vi "Core_Chem_User_Interface_v4.0_Scroll_Pump.vi"() -> ()   [LabVIEW 2014]
uses:
  <vilib>/dex/Stream Element Allocation Mode.ctl
  C:/Program Files (x86)/National Instruments/LabVIEW 2014/examples/Data Communication/Network Streams/Simple Network Streams/support/Network Stream Command.ctl
  <vilib>/Platform/TimedLoop/XDataNode/timing_clust.ctl
  <vilib>/Platform/TimedLoop/XDataNode/nitl_modes.ctl
  <vilib>/Platform/TimedLoop/XDataNode/wakeup.ctl
  <vilib>/NI/STM/TCP/Read Meta Data (TCP Ref).vi
  <vilib>/NI/STM/TCP/Get Connection Reference (TCP).vi
  <vilib>/Utility/tcp.llb/UDP Multicast Read-Only Open.vi
  <vilib>/NI/STM/TCP/Read Meta Data (TCP Clst).vi
  <vilib>/NI/STM/TCP/Read Message (TCP).vi
  <vilib>/platform/TimedLoop/XDataNode/XDataNode.xnode
  <vilib>/Platform/TimedLoop/XDataNode/XDNodeRunTimeDep.lvlib
  <vilib>/FTP/NI_FTP.lvlib
  <vilib>/NI/STM/NI STM.lvlib
panel:
  out "FGGA Scroll Pump\ncommand sender error out":errorcluster
  out "FGGA preflight Des 19":string="This tab controls ONLY for advanced operators."
  out "Scroll Pump not running":string
  out "Network Check error out":errorcluster
  out "Scroll Pump Read Error":errorcluster[](array[cluster])
  out "System status register":bool[](array[boolean])
  out "System status register 2":bool[](array[boolean])
  out "Warning register":bool[](array[boolean])
  out "Fault register":bool[](array[boolean])
  in  "Target IP Address":string="192.168.101.17"
  out "Network error out":errorcluster
  out "Create folder error out 3":errorcluster
  out "Network disconnected":bool
  out "cRIO connection status":bool
  out "SO2 Zeroing (Inflight)\nTime Remain (sec)":u32
  in  "eV6 User set time \n(Inflight) (sec)":i32=120
  in  "SO2 Inflight \nZeroing":bool
  out "Create folder error out 2":errorcluster
  out "Create folder error out":errorcluster
  in  "Confirm Flight Number":bool
  out "PRTAFT_UDP_In":string
  out "TWBOZO01":string
  out "CABOZO01":string
  out "TEIOZO01":string
  out "CHTSOO01":string
  out "CHFGGA01":string
  out "AL52CO01":string
  in  "Flight Number":string
  in  "Tab Control":T1(tab)
  out "FGGA preflight Des 17":string="Preflight - Start minimum 2 hours before take-off\n\n1. Ensure no bags/jackets are stowed on seat backs and behind seats in front of core chemistry rack at all times.\n\n2. Remove inlet covers if applicable.\n\n3. Connect Lilliput mini TFT/LCD VGA cable to FGGA VIDEO (back panel) and PS2 Keyboard/Mouse cables to FGGA Connectors (back panel). TFT/LCD screen kept in WAS/GAS rack Zargers Box. Keyboard/Mouse kept bottom of chemistry rack. (DO NOT disconnect PS2 cable). Connect TFT/LCD AC/DC PSU to 6026-8-98 Amphenol (SSP9) and make 230 Vac CB.\n\n4. Ensure all circuit breakers are pushed in, except 230Vac and 28Vdc, UPS switch off (down) and AL5002 CO Plasma Lamp switch off (down), WoW key to normal (horizontal).\n\n5. Wait for ALL network switches on the aircraft to be up and running before start-up. On the Flight Manager's Interface on the Flight Manager laptop, check SSP icons status (top row) should be all green.  \n\n6. Check AboutTime has synchronised laptop clock to aircraft timeservers (Filiberto/Gaston).\n\nClick the PowerUp Tab."
  out "FGGA preflight Des 16":string="PowerUp\n\n1.\tSSP9 forward face\tMake 3 CBs\n\n2.\tPWRDIST \t\tMake 230Vac CB \n                     Switch UPS On \t[UP]\n                     Make 28Vdc CB\n                     Check 28VDC OK Green Light comes on\n\n3.\tCore Chemistry e-Log\nComplete Core Chemistry e-Log in WordPad (Bnnn_CoreChemLog_v2.2), save on Flight Manager's laptop (192.168.101.180/      flt_folders/Bnnn); Fill in header with date, flight number and your name/initials.\n\n4. Wait for MFM flow rate to display non zero value.\n\n5.\tSAMPUMP\t\t\n - Switch WoW override key (vertical) to check pump starts, and MFM flowrate increase (>20 LPM) on the right hand plot. \n - Switch off WoW override\t\t\t\t [NORM, key horizontal]\n\nClick the 2B Ozone tab if operated, otherwise, click the UDP tab.\n\n\n"
  out "MFM":dbl(graph)
  in  "Ambient = OFF\nCabin = ON":bool
  out "FGGA preflight Des 15":string="2B Ozone Preflight\n\n1.\tSelect either Ambient or Cabin Air mode (default should be OFF for Ambient air mode).\n\n2. Check flowrate is greater than 2000 sccm on the right hand plot.\n\nClick the UDP tab."
  out "2B Ozone concentration":dbl(graph)
  out "2B Ozone flow rate":dbl(graph)
  out "2BOzone Event error out":errorcluster
  out "2BOzone command sender error out":errorcluster
  out "FGGA preflight Des 20":string="4. Check derived parameters in DECADES (192.168.101.110 & 192.168.101.108). 574 Ozone TEi49C; 588 CO AL5002; 611 SO2 TEi43i; 903 - 905 FGGA; 910 / 920 Ozone 2B."
  out "FGGA preflight Des 14":string="UDP Preflight\n1. Check all UDP packets are updating.  Unix time increasing by 1 sec (3rd parameter).\n2. Check flight number is correct.\n3. Confirm flight number and check it appears in the UDP packet (6th parameter). "
  in  "name":string="239.1.4.6"
  in  "Port":u16=50001
  out "FGGA":string
  out "CO":string
  out "TEi49 Ozone":string
  out "2B Cabin Ozone":string
  out "2B Ambient Ozone":string
  out "SO2":string
  in  "Ozone Zeroing Abort":bool
  out "Ozone Zeroing\nTime Remain (sec)":u32
  in  "Ozone Zeroing":bool
  out "TEI49 Sample Flow B":dbl(graph)
  out "TEi49 Concentration":dbl(graph)
  out "TEI49 Sample Flow A":dbl(graph)
  out "FGGA preflight Des 13":string="TEi49 Ozone PRE-FLIGHT - LAST ACTIONS BEFORE SEAT-BELTING DOWN (PRIOR TO ENGINES START)\n\n1. Ozone monitor zeroing\t\t[10 min minimum]\n\n\n2. Check TEi49 zero value and note down value in e-Log. \n"
  out "FGGA preflight Des 12":string="TEi49 Ozone Preflight\n\n1. Check nominal sample flowrate on both channels is ~0.7 LPM."
  out "Ozone Event error out":errorcluster
  out "Ozone command sender error out":errorcluster
  in  "Ozone UDP Time Offset":i32=1
  in  "eV8 span\n(sec)":i32=120
  in  "eV9 span\nflush (sec)":i32=60
  in  "SO2 Span Calibration":bool
  in  "eV9 zero\nflush (sec)":i32=15
  in  "SO2 Zero Calibration":bool
  in  "eV8 zero\n(sec)":i32=30
  in  "SO2 Calibration Abort":bool
  out "SO2 react pressure":dbl(graph)
  in  "Prepare SO2 Zero Gas":bool
  in  "Prepare SO2 Span Gas":bool
  in  "Auto Zeroing \ninterval (sec)":i32=600
  out "Next Auto Zero\nStarts in (sec)":u32
  out "Auto Zero\nIndicator":string="Auto Zero Inactive; Manual Zero Allow"
  out "SO2 Resume Zeroing\nCount down timer (sec)":u32
  in  "SO2 Pause\nAuto Zeroing":bool
  out "TEi43i Concentration scaled / raw":cluster{dbl, dbl}(graph)
  in  "SO2 Auto Zeroing":bool
  out "mean zero\ncal status":bool
  out "SO2 Sensitivity":dbl format="%.2g"
  out "SO2 Zero":dbl format="%.2g"
  in  "eV9 Flush User\nset time (sec)":i32=15
  in  "MFC_3 User Set Value":dbl=2.0
  in  "MFC_2 User Set Value":dbl=2.5
  in  "eV6 User\nset time (sec)":i32=600
  out "SO2 Flush\nTime Remain (sec)":u32
  out "TEI43i MFC3 Sample Flow":dbl(graph)
  out "TEI43C Sample Flow":dbl(graph)
  out "TEI43i MFC2 Cal Flow":dbl(graph)
  out "SO2 Zero CAL\nTime Remain (sec)":u32
  out "SO2 Zero CAL Flush\nTime Remain (sec)":u32
  in  "SO2 Zero CAL":bool
  out "FGGA preflight Des 11":string="TEi43 SO2 Inflight Zero Calibration"
  in  "SO2 GND Zeroing":bool
  out "SO2 Zeroing\nTime Remain (sec)":u32
  out "FGGA preflight Des 10":string="TEi43 SO2 PRE-FLIGHT - LAST ACTIONS BEFORE SEAT-BELTING DOWN (PRIOR TO ENGINES START)\n\n1. SO2 monitors zeroing\t\t[10 min minimum]\n\n2. Check TEi43i or TEi43C zero value and note down value in e-Log.\n\n3. Enable SO2 auto zeroing (if required) and check zeroing interval. "
  in  "SO2 Flush":bool
  out "FGGA preflight Des 9":string="TEi43 SO2 Preflight\n\n1. Check nominal sample flowrate is (2.0 LPM / 1.5 LPM) on the (TEi43i / TEi43c) right hand plot.\n\nSPAN GAS\n1. Connect SO2 Calibration gas to caldeck, then.\n\n2. Press SO2 flush button, MFC2 cal flow should increase to 2.5 SLPM.\nMonitor MFC2 flow rate to make sure the reading decreases from 2.5 SLPM to 0.0 SLPM.\nCheck pressure content and delivery gauges also reads zero.\nIf pressure content & delivery gauges do NOT read zero, press SO2 flush button again until they do.\n\n3. Back out V2, Quickly open and close cylinder valve 1, Set delivery pressure to 3 bar on V2. \n\n4. Repeat step 2) to 3) three times.\n\n5. Open cylinder valve 1, system is ready. Note down content pressure in elog.\n\n6. Press SO2 Span Calibration button to start Span calibration. \n\nZERO AIR\n1. Connect BTCA Zero Air gas to caldeck, then.\n\n2. Set ev9 flush user time to 60 secs and press SO2 Flush button.\n\n3. Press SO2 Zero Calibration button to start Zero Air calibration."
  in  "eV9 flush User\nset time (sec)":i32=30
  in  "eV8 User\nset time (sec)":i32=60
  out "SO2 Event error out":errorcluster
  out "SO2 command sender \nerror out":errorcluster
  in  "SO2 UDP Time Offset":i32=1
  in  "CO Monitor Troubleshooting":bool
  out "Lamp Temperature":dbl(graph)
  out "CO CAL Status":bool
  in  "CO CAL":bool
  out "FGGA preflight Des 8":string="CO Preflight and Inflight Calibrations\nHold down the CAL button for 2 secs then release, CAL status should then lit up.\nCheck CO LED lit up at front instrument. If not, refer to\nInflight calibration performed on 45 minutes interval or more frequently if lamp temperature > 35.5 degC."
  in  "Prepare Gases":bool
  out "FGGA preflight Des 7":string="AL5002 CO Preflight Checks\n\n1.\n\n2. Start CO Vacuum. NB: If there is problem with the software control, use manual override switch [up] on CALDECK front panel\n\n3. CO Checks - charts on the right hand side\n    Lamp Flow Controller ~ 40 ml/min\n    Monochromator Flow Controller ~ 30 ml/min\n    Fluorescence Cell Pressure ~ 7.5 Torr\n\nIf Lamp/Mono flows are low, manual valves (V1 -> V5) may still be shut, or pressure adjusting valves (ALREG1 & 2) have not been set > 2 bar\n\nIf Cell pressure is 10 Torr (max range), check that COPUMP is running and eV7 is opened (CO Vacuum eV7 is ON).\n\n4. Switch Plasma Lamp at the front panel UP\n\nDetector count rate (on 'Raw Signal' or F2 instrument touchscreen) should increase to >=10000 Hz within a minute.  Recycle plasma lamp switch (off/on) if no significant increase in count rate after 10 mins.  CO concentration should increase (100s ppb). \n     \n\n"
  in  "CO Vaccum (eV7)":bool
  out "Raw Signal":dbl(graph)
  out "CO Concentration":dbl(graph)
  out "Fluorescence Cell Pressure":dbl(graph)
  out "Monochromator Flow":dbl(graph)
  out "Lamp Flow Controller":dbl(graph)
  in  "CO UDP Time Offset":i32=1
  out "CO2 Pressure\nDelivery (PSIA)":dbl(slide) scale=0.0..100.0
  out "Std\nContent (barG)":dbl(slide) scale=0.0..220.0
  out "N2\nContent (barG)":dbl(slide) scale=0.0..220.0
  out "CO2\nContent (barG)":dbl(slide) scale=0.0..170.0
  out "CO Event error out":errorcluster
  out "CO command sender error out":errorcluster
  out "CO Zero":T2(array[cluster])
  out "CO Sensitivity":T3(array[cluster])
  in  "NEW\nFGGA Restart":bool
  in  "FGGA Calibration Abort":bool
  out "Ring Down Time RDA & RDB":cluster{dbl, dbl}(graph)
  in  "Line Lock Setting Change":bool
  out "Cell temperature":dbl(graph)
  out "Cell pressure":dbl(graph)
  in  "Manual FGGA Pump":bool
  out "CO2":dbl(graph)
  out "CH4":dbl(graph)
  out "H2O":dbl(graph)
  out "WoW Flag":string="0"
  in  "FGGA pump\nsync to WoW":bool
  out "CH4 Dry":dbl(graph)
  out "CO2 Dry":dbl(graph)
  out "MFC1 Cal Flow":dbl(graph)
  out "Flush Target Tank\nTime Remain (sec)":u32
  out "Flush Low Tank\nTime Remain (sec)":u32
  out "Flush High Tank\nTime Remain (sec)":u32
  in  "Flush Target Tank":bool
  in  "Flush Low Tank":bool
  in  "Flush High Tank":bool
  in  "OLD\nFGGA Restart":bool
  out "FGGA preflight Des 6":string="FGGA Instrument Controls"
  in  "High Cal":bool
  out "High Cal\nFlush Time Remain (sec)":u32
  out "High Cal\nCal Time Remain (sec)":u32
  in  "Low Cal":bool
  in  "Target Cal":bool
  in  "Span Cal - \nHigh Cal, CO Cal, Low Cal":bool
  out "Low Cal\nFlush Time Remain (sec)":u32
  out "Low Cal\nCal Time Remain (sec)":u32
  out "Target Cal\nFlush Time Remain (sec)":u32
  out "Target Cal\nCal Time Remain (sec)":u32
  in  "MFC_1 User Set Value":dbl=2.0
  out "FGGA preflight Des 5":string="FGGA Inflight Calibrations"
  out "FGGA preflight Des 4":string="FGGA Ground Preflight Checks\n\n1. Switch FGGA pump ON\n\n2. Check cavity pressure ~50 Torr\n\n3. Switch FGGA pump OFF\n\n4. Enable FGGA pump sync to WoW\n\n5.. Check Time Synchronisation\n\n6. Check CO2 & CH4 values\n\nIf CO2 & CH4 values are -1 ppm, follow the \nchange linelock settings procedure.\n\n\n\n\n\nLAST ACTION BEFORE SEAT-BELTING \nDOWN (PRIOR TO ENGINES START)\n\n1. Disconnect Monitor & stow away. Leave Keyboard & Mouse connected. Place keyboard at the bottom\nof the rack.\n\n"
  out "FGGA preflight Des 3":string="FGGA CAL Gas Purge\n\nFor each cylinder in gas stowage, check that,\n\n1. V1 Closed\n    V3 Closed\n    V4 Make sure arrow positioned downwards (i.e. flow points to gas line)\n\n2. V3 Open (turn anti-clockwise)\n\n3. Use the button on the right according to the operating cylinder to flush the line. Monitor the MFC flow rate to make sure the reading decreases from 3 to zero. (ie fully flushed). Pressure content & delivery gauges should also read zero.\n\n4. V3 Close (turn clockwise)\n\n5. V1 Open / Close quickly\n         Check delivery pressure gauge is ~ 40 PSI \n         (Use V2 to increase if necessary)\n\n6. Repeat steps 2) to 5) three times\n\n7. V3 Close (turn clockwise)\n\n8. V1 Open, check V2 ~ 40 PSIG\n\n9. V3 Open - System is ready"
  out "FGGA command sender error out":errorcluster
  out "FGGA Event Error out":errorcluster
  in  "FGGA UDP Time Offset":i32=1
  in  "Span Low Flush Time (seconds)":i32=21
  in  "Span Low Cal Time (seconds)":i32=30
  in  "Span High, High Low, Target\nCal Time (seconds)":i32=30
  in  "Span High, High, Low, Target  Cal\nContinue Flush Time (seconds)":i32=11
  in  "Span High, High, Low, Target Cal\nFlush Start Time (seconds)":i32=10
  in  "Time delay (msec) between\nvalves switching":u32=200
  in  "FLOW ALL OFF":bool
  in  "LOW FLOW MASTER SWITCH":bool
  in  "FGGA 140 Torr\nCalibration Abort":bool
  out "Ring Down Time RDA & RDB 2":cluster{dbl, dbl}(graph)
  out "Cell temperature 2":dbl(graph)
  out "Cell pressure 2":dbl(graph)
  out "CO2 2":dbl(graph)
  out "CH4 2":dbl(graph)
  out "H2O 2":dbl(graph)
  out "CH4 Dry 2":dbl(graph)
  out "CO2 Dry 2":dbl(graph)
  in  "High Cal\n140 Torr":bool
  out "High Cal 140 Torr\nFlush Time Remain (sec)":u32
  out "High Cal 140 Torr\nCal Time Remain (sec)":u32
  in  "Low Cal\n140 Torr":bool
  in  "Target Cal\n140 Torr":bool
  in  "Span Cal 140 Torr - \nHigh Cal, CO Cal, Low Cal":bool
  out "Low Cal 140 Torr\nFlush Time Remain (sec)":u32
  out "Low Cal 140 Torr\nCal Time Remain (sec)":u32
  out "Target Cal 140 Torr\nFlush Time Remain (sec)":u32
  out "Target Cal 140 Torr\nCal Time Remain (sec)":u32
  in  "MFC_1 140 Torr\nUser Set Value":dbl=4.0
  out "FGGA preflight Des 23":string="FGGA 140 Torr Inflight Calibrations"
  in  "eV10":bool
  out "Scroll Pump \nat Fault":bool
  out "Measured Motor Current (A)":dbl(graph)
  out "Measured Link Voltage (V)":dbl(graph)
  out "Measured Motor Power (W)":dbl(graph)
  out "Motor Frequency":i32(graph)
  out "Receiver Loop Count":i32
  in  "Standby Speed %\nDefault Set Value":u32=66 min=66 max=100
  in  "Normal Speed Threshold":u32(slide)=50 min=50 max=100 scale=50.0..100.0
  in  "Standby Speed\n66% - 100%":u32=66 min=66 max=100
  in  "Use Standby Speed":bool
  in  "Scroll Pump On/Off":bool
  in  "Scroll Pump Faults":bool
  out "FGGA Scroll Pump Monitoring":string[](array[string])
  out "Pump Controller Temperature":i32(slide) scale=0.0..100.0
  in  "HIGH FLOW MASTER SWITCH":bool
  in  "NEW FGGA Shutdown":bool
  in  "Transfer NEW FGGA Files":bool
  in  "OLD FGGA Shutdown":bool
  in  "Postflight Procedures":bool
  in  "FTP ASCII Files to Local":bool
  in  "Transfer OLD FGGA Files":bool
  out "FGGA preflight Des 18":string="Postflight\n\n1. Perform SO2 Span Gas Calibration (if necessary). \n\n2. Press the FTP ASCII File to Local button to transfer ASCII files to flight folder.\n\n\n3. Press the Transfer FGGA Files button to transfer FGGA files to flight folder. \n\n\n4. Shutdown FGGA.\n\n\n5. View Postflight Procedures."
  out "File List":string[](array[string])
  out "FGGA File Transfer Error out":errorcluster
  out "Move to FM Error out":errorcluster
  out "FGGA File Transfer Error out 2":errorcluster
  out "USB Disk Space Used %":dbl(slide) scale=0.0..100.0
  out "PTP Sync":bool
  out "CPU Total %":dbl(graph)
  out "PRTAFT_DLU":string
  in  "eV12":bool
  in  "eV11":bool
  in  "Pause Auto Zero Count \nDown set time (sec)":i32=600
  out "Calibration gas cylinder \nconcentration (ppb)":dbl format="%.4g"
  in  "Save Calibration gas\ncylinder concentration to file":bool
  in  "Calibration gas cylinder \nconcentration (ppb)":dbl=500.0 format="%.4g"
  in  "Simulate MOCCA Conc":dbl
  in  "MOCCA window \ndelay time (sec)":i32=30
  in  "MOCCA Limit":i32=800
  in  "SO2 Inflight MOCCA Alarm\n(default = OFF)":bool
  in  "Offset Mean Zero Calculation (default = ON)\nOFF = User input\nOn = Mean zero calculated with ev8":bool=TRUE
  in  "Inst_alm_thresh":i32=220
  in  "3hr_alm_thresh":i32=80
  in  "Simulate Inst Conc":i32
  in  "Simulate 3hr Average Conc":dbl
  in  "Simulate 2B Conc":bool
  in  "Ozone eV6":bool
  in  "Simulate Conc":bool
  in  "8hr TWA Limit":i32=490
  in  "10mins STEL Limit":i32=800
  in  "SO2 Sensitivity":dbl=1.1
  in  "SO2 Zero":dbl
  in  "Simulate TWA Conc":dbl
  in  "Simulate STEL Conc":dbl
  in  "MFC_3\nSLPM Value":dbl=2.0
  in  "MFC_2\nSLPM Value":dbl
  in  "SO2 eV6":bool
  in  "eV8":bool
  in  "eV9":bool
  in  "eV4":bool
  in  "eV3":bool
  in  "MFC_1\nSLPM Value":dbl
  in  "eV2":bool
  in  "eV1":bool
  in  "cRIO File IO Stop\n(USB Flash Drive Unmount)":bool
  # "Stop command received and pump is stopping"
  # "Power limit is active"
  # "Accelerating / running"
  # "Acceleration is limited"
  # "Standby Active"
  # "Deceleration is limited"
  # "Above normal speed"
  # "Operating above the ramp speed threshold"
  # "Operating above the overload speed threshold"
  # "Warning Condition"
  # "Control mode"
  # "Fault Condition"
  # "Serial enable active"
  # "Unix time"
  # "Flight Number"
  # "concentration (scaled)\npmt_volt\nlamp_volt\nlamp_intens\ninternal_temper\nreact_temper\nreact_press\nflow\nflags\nten_min_so2\neight_hr_so2\nten_min_so2_alm\neight_hr_so2_alm\nMFC_2absolute_pres\nMFC_2temperature\nMFC_2volumetic_flow\nMFC_2mass_flow\nMFC_2set_point\nMFC_3_absolute_pres\nMFC_3_temperature\nMFC_3volumetic_flow\nMFC_3mass_flow\nMFC_3set_point\nV6\nV8\nV9\nMFC2_Set_Value\nMFC3_Set_Value\nconcentration (raw)\nmean calculation status\noffset\nsensitivity\nev8_user_set_time\nauto_zeroing_control\nev8_zero_interval\nMOCCA_inflight_alarm\nMOCCA_time_window_delay\nMOCCA_SO2_limit\n10 min STEL limit\n8 hour TWA limit\nSO2 cal gas cylin conc\nsimulate_SO2_conc_control\nMOCCA_SO2_sim_value\nMOCCA_SO2_alarm"
  # "Unix time"
  # "Unix time"
  # "Unix time"
  # "Unix time"
  # "Flight Number"
  # "Flight Number"
  # "Flight Number"
  # "Flight Number"
  # "conc\ntemp\npress\nflow\nthreehr_oz\nInst_alarm\nthreehr_alarm"
  # "ch4\nco2\nh2o\npress_torr\ntemp_c\nfit_flag\nrda_usec\nrdb_usec\nch4_dry\nco2_dry\nMFC_1_absolute_pres\nMFC_1_temperature\nMFC_1volumetic_flow\nMFC_1mass_flow\nMFC_1set_point\nV1\nV2\nV3\nV4\nrestart_FGGA\nFGGA_Pump\nCAL_MFC_1Set_Value"
  # "conc\ntemp\npress\nflow"
  # "conc\nbenchtemp\npress\ncellAint\ncellBint\nFlowA\nFlowB\nlamptemp\nflag\nV6"
  # "conc\ncounts\nsens\nzero\nlampflow\nlamptemp\nmonoflow\nmonotemp\nmonopress\ncellpress\ncalpress\ntemppmt\ncalconc\nerr\ncal_counter\nerr_counter\nCO_vacuum_status\nIn_Cal\nALEG1_press_delivery\nALREG1_press_content\nALREG2_press_content\nALREG3_press_content"
  # "TEi43c"
  # "TEi43i"
  # "SO2 Inflight ZERO CAL SETTINGS"
  # "FGGA Scroll Pump"
  # "FGGA"
  # "2B Ozone"
  # "TEi49C  - Ozone"
  # "TEi43 - SO2"
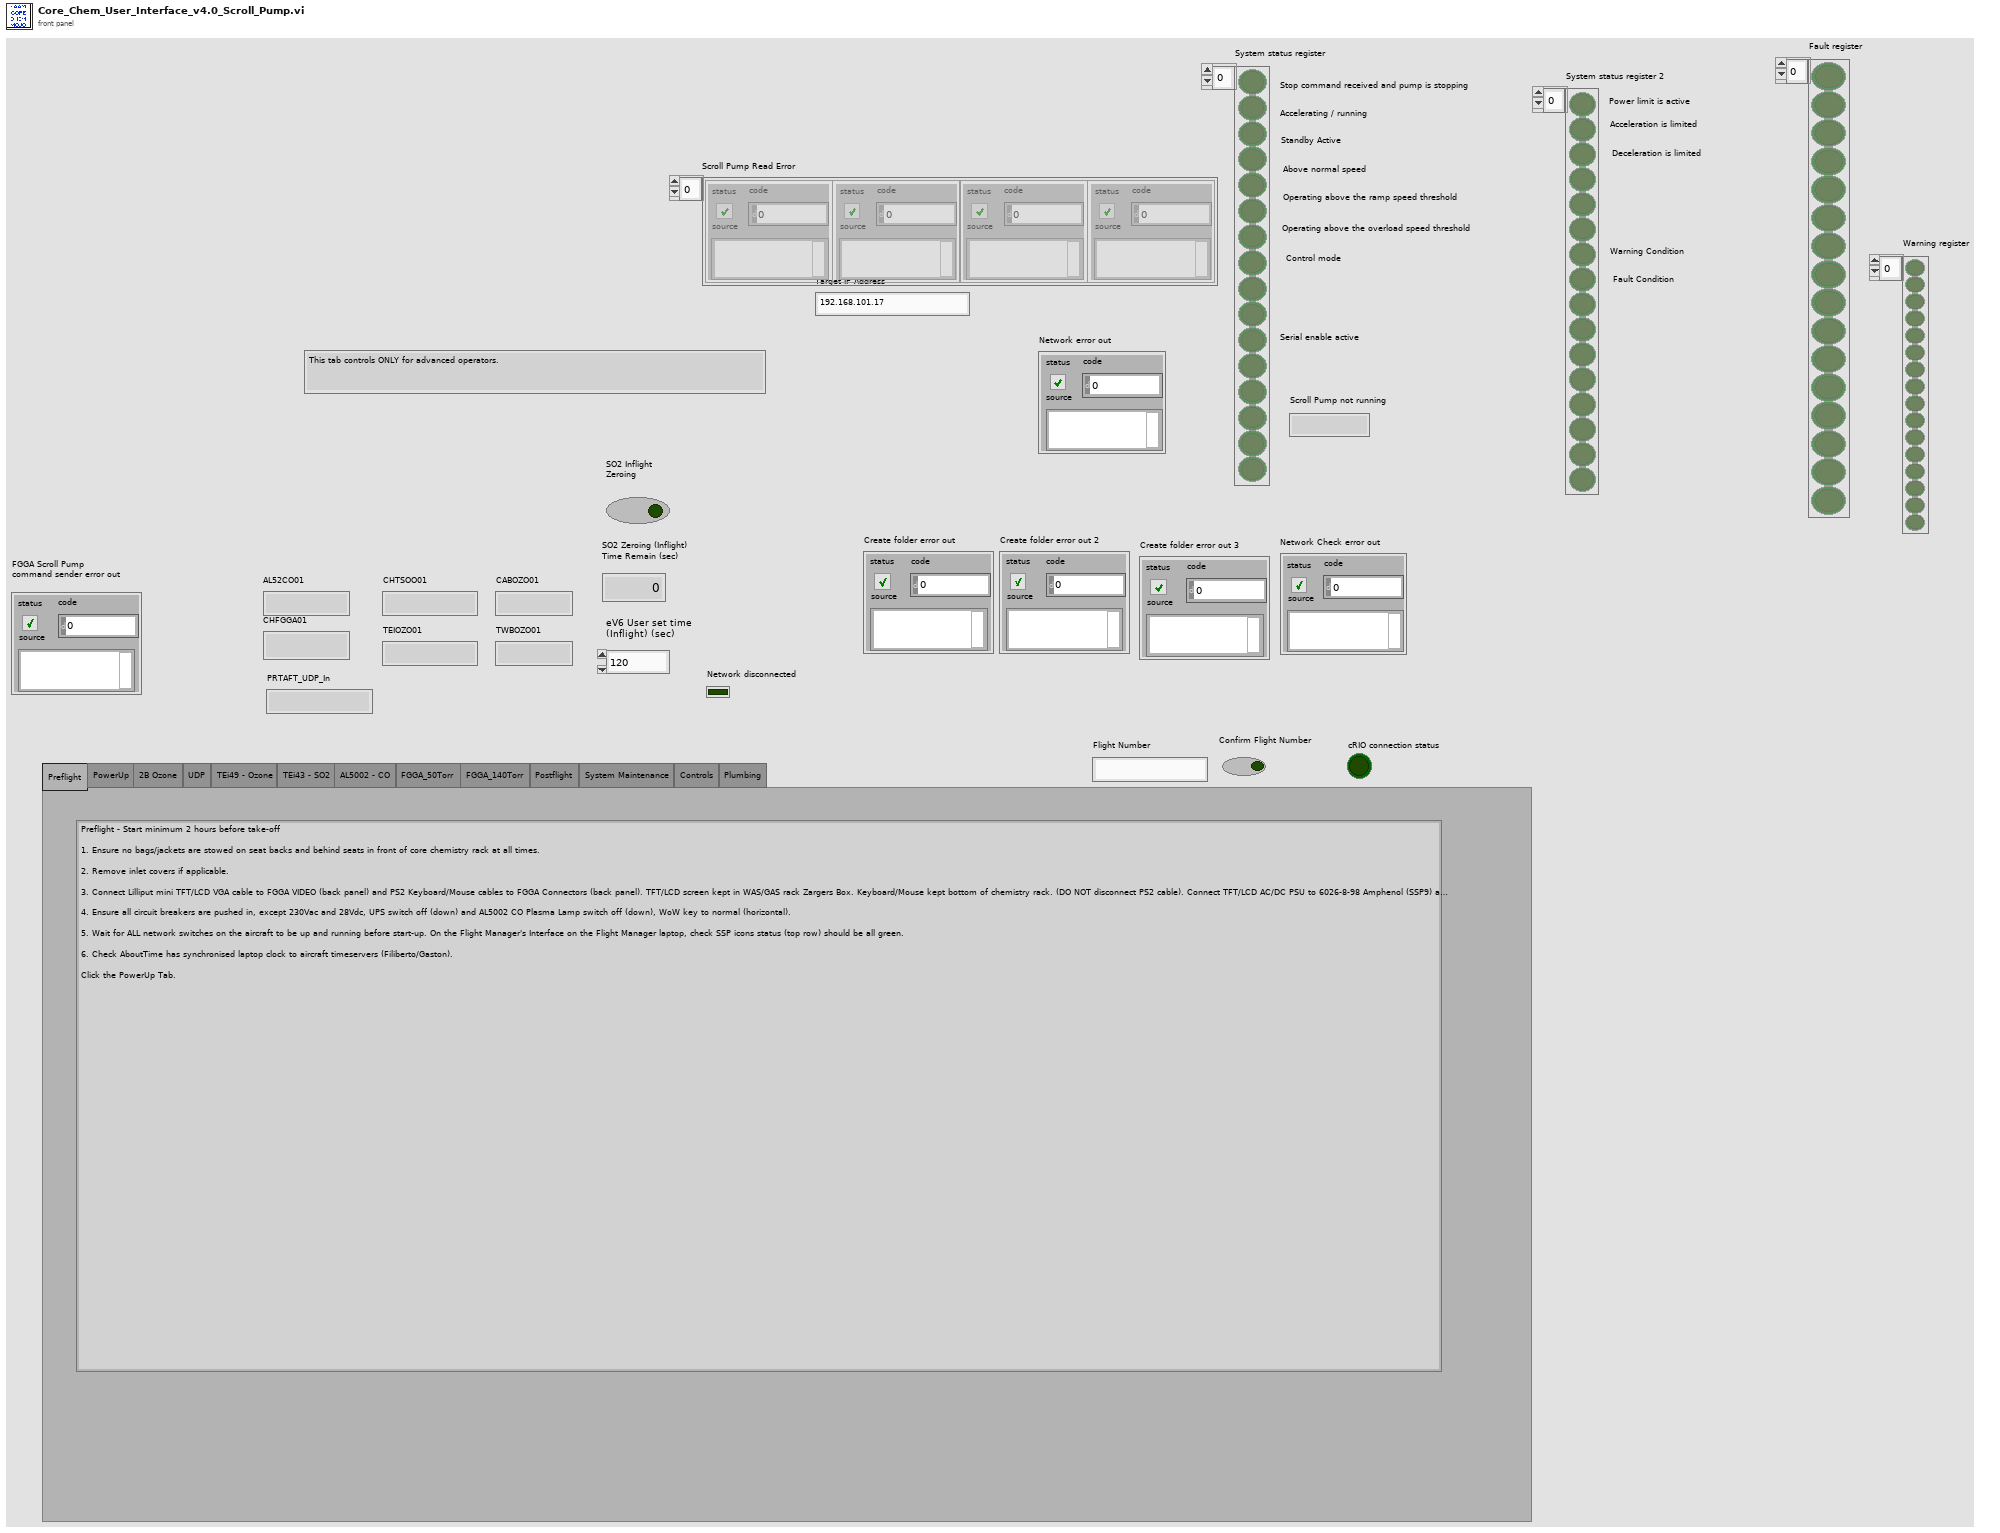
[diagram p1: front panel]
types:
  T1 = enum32{"Preflight", "PowerUp", "2B Ozone", "UDP", "TEi49 - Ozone", "TEi43 - SO2", "AL5002 - CO", "FGGA_50Torr", "FGGA_140Torr", "Postflight", "System Maintenance", "Controls", "Plumbing"}
  T2 = cluster{"time stamp":timestamp, "CO Offset":dbl}[]
  T3 = cluster{"time stamp":timestamp, "CO Sensitivity":dbl}[]
  T4 = typedef "Stream Element Allocation Mode.ctl" = u32
  T5 = typedef "Network Stream Command.ctl" = cluster{"Message":string, "Message Data":variant}
  T6 = typedef "XDNodeRunTimeDep.lvlib/timing_clust.ctl" = cluster{"Expected End [f-1]":u64, "Actual End [f-1]":u64, "Finished Late? [f-1]":bool, "Expected End [i-1]":u64, "Actual End [i-1]":u64, "Finished Late? [i-1]":bool, "Expected Start [i]":u64, "Actual Start [i]":u64, "Expected Start [f]":u64, "Actual Start [f]":u64, "Source Name":string, "Structure Name":string, "Period":i64, "Deadline":i64, "Offset":i64, "Start":i64, "Priority":i32, "Timeout":i32, "Mode":T7, "Wakeup Reason":T8, "Error":errorcluster, "Source Type":string, "Secondary Source Type":string, "Global End Time":u64, "Global Start Time":u64, "Frame Duration":u64, "Iteration Duration":u64, "Assigned CPU":i32, "I/O Scan Engine Mode":u32}
  T7 = typedef "XDNodeRunTimeDep.lvlib/nitl_modes.ctl" = enum32{"No Change", "Process missed periods, maintain original phase", "Discard missed periods, maintain original phase", "Process missed periods, ignore original phase", "Discard missed periods, ignore original phase"}
  T8 = typedef "XDNodeRunTimeDep.lvlib/wakeup.ctl" = enum32{"Normal", "Aborted", "Asynchronous wakeup", "Timing source error", "Timed loop error", "Timeout"}
  T9 = typedef "NI_FTP.lvlib/FTP Session.ctl" = refnum<k5>
  T10 = typedef "NI_FTP.lvlib/FTP File Info.ctl" = cluster{"type":enum16{"unknown", "file", "dir", "link"}, "permissions":string, "owner":string, "group":string, "size":i32, "date":string, "name":string, "link name":string}
  T11 = cluster{"Message":string, "Message 2":string, "Message 3":string}
  T12 = cluster{"Message":string, "Message 2":string, "Message 3":string, "Message 4":string}
  T13 = cluster{"Message 2":string, "Message 3":string, "Message 4":string}
  T14 = cluster{"Message":string, "Message 3":string, "Message 4":string}
  T15 = typedef "NI STM.lvlib/TCP Connection Info.ctl" = cluster{"connection ID":refnum<k5>, "meta data":T16[]}
  T16 = typedef "NI STM.lvlib/MetaDataElement.ctl" = string
  T17 = typedef "NI STM.lvlib/TCP Data Info.ctl" = cluster{"data size":i32}
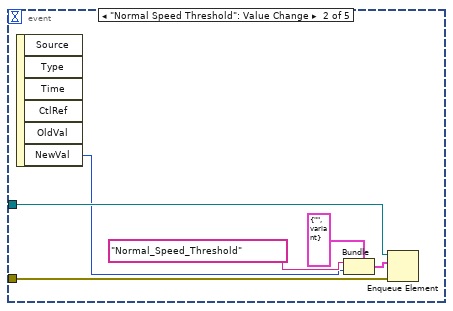
[diagram p3: hidden frame]
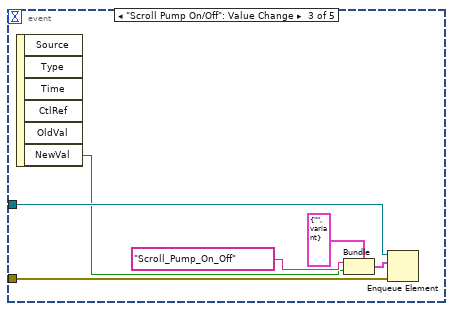
[diagram p4: hidden frame]
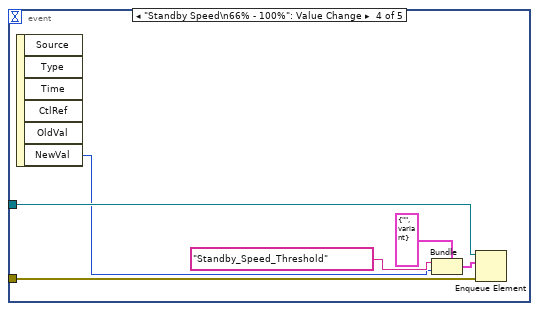
[diagram p5: hidden frame]
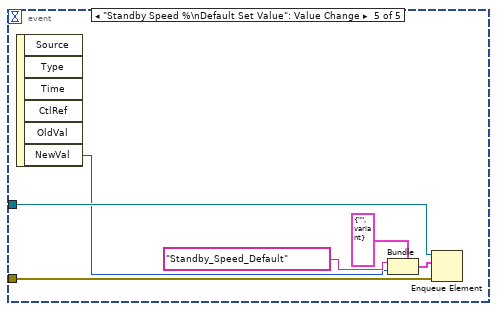
[diagram p6: hidden frame]
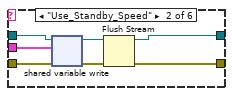
[diagram p8: hidden frame]
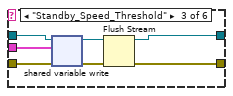
[diagram p9: hidden frame]
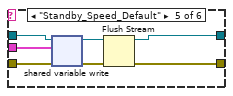
[diagram p10: hidden frame]
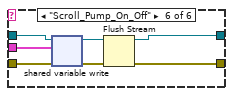
[diagram p11: hidden frame]
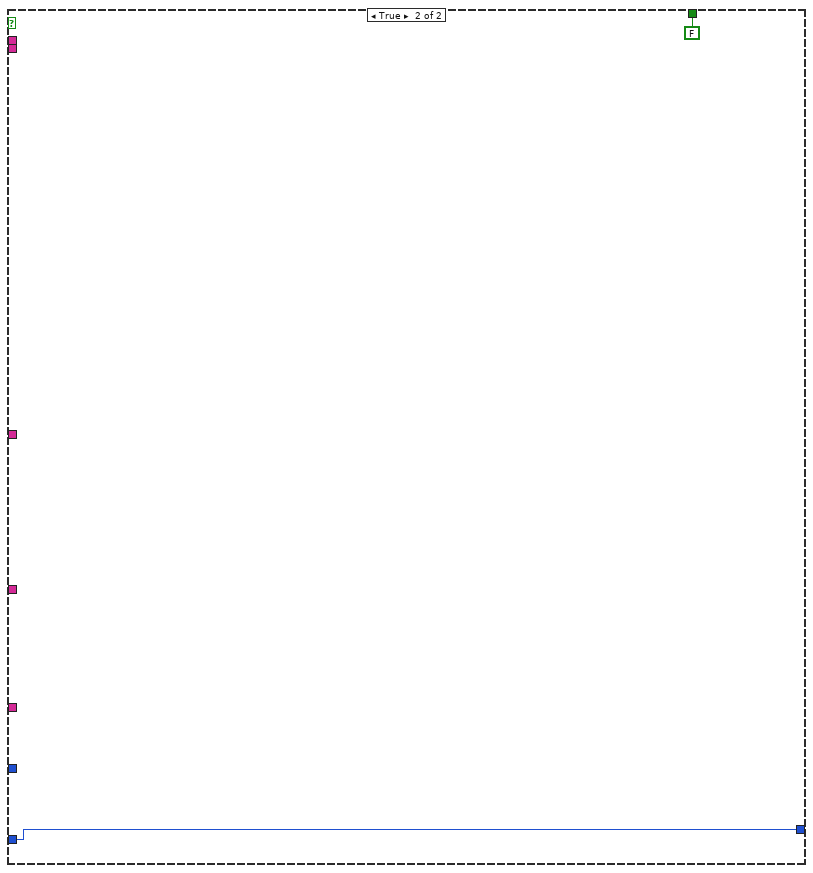
[diagram p16: hidden frame]
diagram:
  w8 = T4 0 items=["allocate as needed", "pre-allocate"] ("element allocation mode")
  w3 = T5 {"Message"="", "Message Data"=variant} ("Message Cluster")
  w19 = "XXXX"
  w21 = 0
  w22 = 0.0
  w28 = T5 {"Message"="", "Message Data"=variant} ("Message Cluster")
  w34 = T4 0 items=["allocate as needed", "pre-allocate"] ("element allocation mode")
  w40 = T5 {"Message"="", "Message Data"=variant} ("Message Cluster")
  w46 = T4 0 items=["allocate as needed", "pre-allocate"] ("element allocation mode")
  w51 = T5 {"Message"="", "Message Data"=variant} ("Message Cluster")
  w56 = T4 0 items=["allocate as needed", "pre-allocate"] ("element allocation mode")
  w65 = T4 0 items=["allocate as needed", "pre-allocate"] ("element allocation mode")
  w67 = T5 {"Message"="", "Message Data"=variant} ("Message Cluster")
  w74 = T4 0 items=["allocate as needed", "pre-allocate"] ("element allocation mode")
  w76 = T5 {"Message"="", "Message Data"=variant} ("Message Cluster")
  n1 = local write "cRIO File IO Stop\n(USB Flash Drive Unmount)"(FALSE ("Stop File Write")) -> ()
  n2 = local write "Flight Number"(w19) -> ()
  n3 = while {
    shift-right: [w80] -> _
    shift-left: w19 -> [w79]
    stop <- FALSE stop-if-true
    n4 = Not Equal?(x=w79, y="Flight Number") -> (x != y?=w82:bool)
    n5 = case shown="True" w82 {
      tunnel: [w85 w86] -> w80
      tunnel: "Flight Number" -> [_ w86]
      tunnel: w79 -> [w85 _]
      frame False {
      }
      frame True {
        n6 = One Button Dialog(message="Flight Number changed,\nPress flight number button to confirm") -> ()  [unwired: 1 in, 1 out]
      }
    }
    n7 = Wait (ms)(milliseconds to wait=u32 1000) -> ()  [unwired: 1 out]
  }
  n8 = while {
    stop <- FALSE stop-if-true
    # "UDP Read"
    n9 = String To IP(1:"name") -> (0:w93:u32)
    n10 = call-poly <vilib>:"UDP Multicast Open.vi"("multicast addr"=w93, "port"="Port") -> ("error out"=w91:errorcluster, "connection ID"=w90:refnum<k16>)  [unwired: 7 in, 1 out]
    n11 = Wait (ms)(milliseconds to wait=u32 1000) -> ()  [unwired: 1 out]
    n12 = case shown="No Error" w91 {
      selector: w91 -> [w97 _]
      tunnel: w90 -> [w96 _]
      frame No Error {
        w95 = ""
        n13 = while {
          tunnel: w97 -> [w143]
          tunnel: w96 -> [w142]
          shift-right: [w138] -> _
          shift-left: w95 -> [w139]
          shift-right: [w129] -> _
          shift-left: w95 -> [w131]
          shift-right: [w123] -> _
          shift-left: w95 -> [w125]
          shift-right: [w117] -> _
          shift-left: w95 -> [w118]
          shift-right: [w111] -> _
          shift-left: w95 -> [w112]
          shift-right: [w105] -> _
          shift-left: w95 -> [w106]
          shift-right: [w99] -> _
          shift-left: w95 -> [w100]
          stop <- w141 stop-if-true
          n14 = UDP Read(connection ID=w142, 8:w143) -> (data out=w98:string, error out=w141:errorcluster)  [unwired: 2 in, 3 out]
          n15 = Match Pattern(string=w98, regular expression="$TEIOZO") -> (match substring=w137:string, after substring=w136:string)  [unwired: 1 in, 2 out]
          n16 = Match Pattern(string=w98, regular expression="$TWBOZO01,") -> (match substring=w115:string, after substring=w114:string)  [unwired: 1 in, 2 out]
          n17 = Match Pattern(string=w98, regular expression="$CABOZO01,") -> (match substring=w121:string, after substring=w120:string)  [unwired: 1 in, 2 out]
          n18 = Match Pattern(string=w98, regular expression="$CHTSOO") -> (match substring=w109:string, after substring=w108:string)  [unwired: 1 in, 2 out]
          n19 = Match Pattern(string=w98, regular expression="$CHFGGA") -> (match substring=w133:string, after substring=w132:string)  [unwired: 1 in, 2 out]
          n20 = Match Pattern(string=w98, regular expression="$AL52CO01,") -> (match substring=w127:string, after substring=w126:string)  [unwired: 1 in, 2 out]
          n21 = Match Pattern(string=w98, regular expression="$PRTAFT01,") -> (match substring=w104:string, after substring=w103:string)  [unwired: 1 in, 2 out]
          n22 = Concatenate Strings(w137, w136) -> (w135:string)
          n23 = Concatenate Strings(w115, w114) -> (w113:string)
          n24 = Concatenate Strings(w121, w120) -> (w119:string)
          n25 = Concatenate Strings(w109, w108) -> (w107:string)
          n26 = Concatenate Strings(w133, w132) -> (w130:string)
          n27 = Concatenate Strings(w127, w126) -> (w124:string)
          n28 = Concatenate Strings(w104, w103) -> (w101:string)
          n29 = Replace Substring(4:w113, 5:w112) -> (1:w111:string)  [unwired: 2 in, 1 out]
          "TWBOZO01" <- w111
          n30 = Replace Substring(4:w135, 5:w139) -> (1:w138:string)  [unwired: 2 in, 1 out]
          "TEIOZO01" <- w138
          n31 = Replace Substring(4:w119, 5:w118) -> (1:w117:string)  [unwired: 2 in, 1 out]
          "CABOZO01" <- w117
          n32 = Replace Substring(4:w107, 5:w106) -> (1:w105:string)  [unwired: 2 in, 1 out]
          "CHTSOO01" <- w105
          n33 = Replace Substring(4:w124, 5:w125) -> (1:w123:string)  [unwired: 2 in, 1 out]
          "AL52CO01" <- w123
          n34 = Replace Substring(4:w130, 5:w131) -> (1:w129:string)  [unwired: 2 in, 1 out]
          "CHFGGA01" <- w129
          n35 = Replace Substring(4:w101, 5:w100) -> (1:w99:string)  [unwired: 2 in, 1 out]
          "PRTAFT_UDP_In" <- w99
        }
      }
      frame Error {
      }
    }
  }
  n36 = Obtain Queue(name (unnamed)="CO_Command", element data type=w76) -> (queue out=w27:refnum<queue>, error out=w70:errorcluster)  [unwired: 3 in, 1 out]
  n37 = Create Network Stream Writer Endpoint(6:w74, 7:10 ("writer buffer size"), 9:w76, 10:"//192.168.101.17/command/reader/CO" ("reader url"), 11:"/command/writer/CO" ("writer name")) -> (0:w73:errorcluster, 3:w72:refnum<k21>)  [unwired: 2 in]
  n38 = while {
    tunnel: w27 -> [w147]
    tunnel: w70 -> [w146]
    tunnel: [w144] -> _
    stop <- FALSE stop-if-true
    # "CO UI Event Handler Loop"
    n39 = event shown="[4] \"Confirm Flight Number\": Value Change" {
      selector: _ -> [_ _ _ _ _]
      dyn-events: _ -> [_ _ _ _ _]
      timeout: _ -> [_ _ _ _ _]
      tunnel: w147 -> [w154 w161 w165 w172 w180]
      tunnel: w146 -> [w153 w160 w164 w171 w179]
      tunnel: [w148 w155 w163 w170 w178] -> w144
      event "CO CAL": Value Change {
        n40 = event-data() -> ("NewVal"=w151:bool)  [unwired: 1 in]
        n41 = Bundle(cluster=T5 {"Message"="", "Message Data"=variant} ("Message Cluster"), "Message"="CO CAL", "Message Data"=w151) -> (w149:T5)
        n42 = Enqueue Element(queue=w154, element=w149, error in (no error)=w153) -> (error out=w148:errorcluster)  [unwired: 1 in, 2 out]
      }
      event "CO UDP Time Offset": Value Change {
        n43 = event-data() -> ("NewVal"=w158:i32)  [unwired: 1 in]
        n44 = Bundle(cluster=T5 {"Message"="", "Message Data"=variant} ("Message Cluster"), "Message"="UDP Time Offset", "Message Data"=w158) -> (w156:T5)
        n45 = Enqueue Element(queue=w161, element=w156, error in (no error)=w160) -> (error out=w155:errorcluster)  [unwired: 1 in, 2 out]
      }
      event "CO Vaccum (eV7)": Value Change {
        n46 = event-data() -> ("NewVal"=w162:bool)  [unwired: 1 in]
        n47 = Bundle(cluster=T5 {"Message"="", "Message Data"=variant} ("Message Cluster"), "Message"="CO Vacuum", "Message Data"=w162) -> (w166:T5)
        n48 = Enqueue Element(queue=w165, element=w166, error in (no error)=w164) -> (error out=w163:errorcluster)  [unwired: 1 in, 2 out]
      }
      event "cRIO File IO Stop\n(USB Flash Drive Unmount)": Value Change {
        n49 = event-data() -> ("NewVal"=w169:bool)  [unwired: 1 in]
        n50 = Bundle(cluster=T5 {"Message"="", "Message Data"=variant} ("Message Cluster"), "Message"="Stop File Write", "Message Data"=w169) -> (w173:T5)
        n51 = Enqueue Element(queue=w172, element=w173, error in (no error)=w171) -> (error out=w170:errorcluster)  [unwired: 1 in, 2 out]
      }
      event "Confirm Flight Number": Value Change {
        n52 = event-data() -> ()  [unwired: 1 in, 1 out]
        n53 = flat-sequence {
          tunnel: w179 -> [w182]
          tunnel: w180 -> [w183]
          tunnel: [w183] -> w177
          tunnel: [w182] -> w176
          tunnel: [w185] -> w178
          tunnel: w177 -> [w187]
          tunnel: w176 -> [w186]
          frame #0 {
            n54 = local write "cRIO File IO Stop\n(USB Flash Drive Unmount)"(FALSE ("cRIO File IO Stop\n(USB Flash Drive Unmount)")) -> ()
          }
          frame #1 {
            n55 = local read "Flight Number"() -> (w184:string)
            n56 = Bundle(cluster=T5 {"Message"="", "Message Data"=variant} ("Message Cluster"), "Message"="Flight Number", "Message Data"=w184) -> (w188:T5)
            n57 = Enqueue Element(queue=w187, element=w188, error in (no error)=w186) -> (error out=w185:errorcluster)  [unwired: 1 in, 2 out]
          }
        }
      }
    }
    "CO Event error out" <- w144
  }
  n58 = while {
    tunnel: w27 -> [w198]
    shift-right: [w193] -> _
    shift-left: w72 -> [w195]
    shift-right: [w191] -> w61
    shift-left: w73 -> [w197]
    tunnel: w70 -> [w192]
    stop <- w191 stop-if-true
    # "CO UI Command Sender"
    n59 = Dequeue Element(queue=w198, error in (no error)=w192) -> (element=w194:T5)  [unwired: 1 in, 3 out]
    n60 = Unbundle By Name(w194) -> ("Message"=w196:string)
    n61 = case shown="\"UDP Time Offset\"" w196 {
      tunnel: w197 -> [w199 w203 w210 w217 w224 w231]
      tunnel: w195 -> [w200 w206 w213 w220 w227 w234]
      tunnel: w194 -> [_ w205 w212 w219 w226 w233]
      tunnel: [w199 w202 w209 w216 w223 w230] -> w191
      tunnel: [w200 w201 w208 w215 w222 w229] -> w193
      frame "False", Default {
      }
      frame "CO CAL" {
        n62 = shared-variable-write(w206, w203, w205) -> (w204:refnum<k21>, w207:errorcluster)  [unwired: 1 in, 1 out]
        n63 = Flush Stream(8:w207, 11:w204) -> (0:w202:errorcluster, 3:w201:refnum<k21>)  [unwired: 2 in, 1 out]
      }
      frame "UDP Time Offset" {
        n64 = shared-variable-write(w213, w210, w212) -> (w211:refnum<k21>, w214:errorcluster)  [unwired: 1 in, 1 out]
        n65 = Flush Stream(8:w214, 11:w211) -> (0:w209:errorcluster, 3:w208:refnum<k21>)  [unwired: 2 in, 1 out]
      }
      frame "Stop File Write" {
        n66 = shared-variable-write(w220, w217, w219) -> (w218:refnum<k21>, w221:errorcluster)  [unwired: 1 in, 1 out]
        n67 = Flush Stream(8:w221, 11:w218) -> (0:w216:errorcluster, 3:w215:refnum<k21>)  [unwired: 2 in, 1 out]
      }
      frame "Flight Number" {
        n68 = shared-variable-write(w227, w224, w226) -> (w225:refnum<k21>, w228:errorcluster)  [unwired: 1 in, 1 out]
        n69 = Flush Stream(8:w228, 11:w225) -> (0:w223:errorcluster, 3:w222:refnum<k21>)  [unwired: 2 in, 1 out]
      }
      frame "CO Vacuum" {
        n70 = shared-variable-write(w234, w231, w233) -> (w232:refnum<k21>, w235:errorcluster)  [unwired: 1 in, 1 out]
        n71 = Flush Stream(8:w235, 11:w232) -> (0:w230:errorcluster, 3:w229:refnum<k21>)  [unwired: 2 in, 1 out]
      }
    }
  }
  "CO command sender error out" <- w61
  n72 = node-c288() -> (w26:T6)  [unwired: 4 in]
  n73 = Initialize Array(cluster{"time stamp":timestamp, "Y":dbl} {"time stamp"=timestamp(0 s since 1904-01-01), "Y"=0.0}, 30 ("dimension size")) -> (w23:cluster{"time stamp":timestamp, "Y":dbl}[])
  n74 = timed-loop {
    timing: w26 -> [_]
    timing-out: [_] -> w25
    stop <- _ stop-if-true
    # "PC Tasks"
    n75 = node-c288() -> ()  [unwired: 1 in, 1 out]
    n76 = event shown="[3] \"OLD FGGA Restart\": Value Change" {
      selector: _ -> [_ _ _ _ _ _ _]
      dyn-events: _ -> [_ _ _ _ _ _ _]
      timeout: _ -> [_ _ _ _ _ _ _]
      event "FTP ASCII Files to Local": Value Change {
        n77 = event-data() -> ()  [unwired: 1 in, 1 out]
        n78 = flat-sequence {
          tunnel: [w244] -> w238
          tunnel: [w256] -> w243
          tunnel: [w255] -> w241
          tunnel: [w254] -> w239
          tunnel: w238 -> [w254]
          tunnel: w243 -> [w314]
          tunnel: [w314] -> w242
          tunnel: w241 -> [w310]
          tunnel: [w309] -> w240
          tunnel: w239 -> [w309]
          tunnel: w242 -> [w320]
          tunnel: w240 -> [w315]
          frame #0 {
            n79 = local read "Flight Number"() -> (w246:string)
            n80 = Concatenate Strings("Confirm Flight Number" ("message"), "\n", w246) -> (w250:string)
            n81 = Two Button Dialog(message=w250, 1:"No" ("F button name (\"Cancel\")"), 2:"Yes" ("T button name (\"OK\")")) -> (T button?=w247:bool)
            n82 = case shown="False" w247 {
              tunnel: w246 -> [_ w253]
              tunnel: [w252 w253] -> w244
              frame False {
                n83 = call "Prompt User for Flight Number2"() -> ("Flight Number BXXX"=w252:string)  [unwired: 17 in, 2 out]
              }
              frame True {
              }
            }
          }
          frame #1 {
            n84 = Get Date/Time In Seconds() -> (seconds since 1Jan1904=w260:timestamp)
            n85 = Format Date/Time String(time format string (%c)="%Y%m%d", seconds (now)=w260) -> (date/time string=w258:string)  [unwired: 1 in]
            n86 = call <vilib>:"FTP Open Session.vi"("address"="192.168.101.17") -> ("error out"=w275:errorcluster, "ftp session"=w276:T9)  [unwired: 7 in, 2 out]
            n87 = Concatenate Strings("Use Today's Date" ("message"), "\r", w258) -> (w264:string)
            n88 = call <vilib>:"FTP Logon.vi"("error in (no error)"=w275, "password"="", "user"="anonymous", "ftp session"=w276) -> ("error out"=w272:errorcluster, "ftp session out"=w271:T9)  [unwired: 4 in, 2 out]
            n89 = Two Button Dialog(message=w264, 1:"No" ("F button name (\"Cancel\")"), 2:"Yes" ("T button name (\"OK\")")) -> (T button?=w261:bool)
            n90 = case shown="False" w261 {
              tunnel: [w279 w280] -> w255
              tunnel: w258 -> [_ w280]
              frame False {
                n91 = call "Prompt User for Date"() -> ("Date"=w279:string)  [unwired: 17 in, 2 out]
              }
              frame True {
              }
            }
            n92 = call <vilib>:"FTP Directory Listing.vi"("error in (no error)"=w272, "directory path"="/U:/data", "ftp session"=w271) -> ("dir list"=w270:T10[])  [unwired: 4 in, 4 out]
            n93 = for {
              tunnel: w270 -> [w300] mode=indexing
              tunnel: [w299] -> w267 mode=indexing
              tunnel: w255 -> [w298]
              # "Extract File Name According to the Date"
              n94 = Unbundle By Name(w300) -> ("name"=w306:string, "name"=w305:string)
              n95 = Match Pattern(string=w305, regular expression="_[0-9]+") -> (match substring=w303:string)  [unwired: 1 in, 3 out]
              n96 = String Subset(string=w303, offset (0)=1) -> (substring=w301:string)  [unwired: 1 in]
              n97 = Equal?(x=w301, y=w298) -> (x = y?=w307:bool)
              n98 = case shown="False" w307 {
                tunnel: w306 -> [_ w308]
                tunnel: [_ w308] -> w299
                frame False {
                }
                frame True {
                }
              }
            }
            n99 = Array Size(array=w267) -> (size(s)=w269:i32)
            n100 = for {
              N: w269 -> [_]
              shift-right: [w287] -> w257
              shift-left: w267 -> [w288]
              shift-right: [w285] -> _
              shift-left: 0 -> [w286]
              # "Remove Empty Array"
              n101 = Index Array(array=w288, index=w286) -> (element=w290:string)
              n102 = Equal?(x=w290, y="") -> (x = y?=w289:bool)
              n103 = case shown="True" w289 {
                tunnel: w288 -> [w294 w297]
                tunnel: w286 -> [w293 w295]
                tunnel: [w294 w296] -> w287
                tunnel: [w292 w295] -> w285
                frame False {
                  n104 = Increment(x=w293) -> (x+1=w292:i32)
                }
                frame True {
                  n105 = Delete From Array(array=w297, index=w295) -> (array with subset deleted=w296:string[])  [unwired: 1 in, 1 out]
                }
              }
            }
            "File List" <- w257
            n106 = for {
              tunnel: w257 -> [w283] mode=indexing
              tunnel: [w281] -> w256 mode=indexing
              # "Specify destination path for each file"
              n107 = Concatenate Strings("C:\\temp\\", w283) -> (w282:string)
              n108 = String To Path(string=w282) -> (path=w281:path)
            }
          }
          frame #2 {
            # "FTP a list of files"
            n109 = call <vilib>:"System Exec.vi"("wait until completion? (T)"=TRUE, "working directory"=path "C:/temp", "standard input"=w310, "command line"="C:\\temp\\transfer_ascii_files.bat") -> ()  [unwired: 4 in, 4 out]
          }
          frame #3 {
            # "Move file from local PC to Flight Folder"
            n110 = Build Path(base path=path "\\\\192.168.101.180\\flt_folders" ("path"), name or relative path=w315) -> (appended path=w322:path)
            n111 = Concatenate Strings(w315, "_" ("string"), "corechem" ("string")) -> (w321:string)
            n112 = Build Path(base path=w322, name or relative path=w321) -> (appended path=w317:path)
            n113 = Create Folder(path (use dialog)=w317) -> (created path=w316:path, error out=→"Create folder error out 2":errorcluster)  [unwired: 2 in, 1 out]
            n114 = for {
              tunnel: w316 -> [w329]
              tunnel: [w328] -> w319
              tunnel: w320 -> [w326] mode=indexing
              n115 = Copy(9:TRUE ("overwrite (F)"), 10:w329, 11:w326) -> (0:w328:errorcluster)  [unwired: 2 in, 2 out]
            }
            "Move to FM Error out" <- w319
          }
          frame #4 {
            n116 = local write "FTP ASCII Files to Local"(FALSE ("FTP Files to Local")) -> ()
          }
        }
      }
      event "Transfer OLD FGGA Files": Value Change {
        n117 = event-data() -> ()  [unwired: 1 in, 6 out]
        n118 = flat-sequence {
          tunnel: [w335] -> w334
          tunnel: w334 -> [w347]
          tunnel: [w347] -> w333
          tunnel: [w346] -> w332
          tunnel: [w345] -> w331
          tunnel: w333 -> [w357]
          tunnel: w332 -> [w356]
          tunnel: w331 -> [w358]
          frame #0 {
            n119 = local read "Flight Number"() -> (w336:string)
            n120 = Concatenate Strings("Confirm Flight Number" ("message"), "\n", w336) -> (w338:string)
            n121 = Two Button Dialog(message=w338, 1:"No" ("F button name (\"Cancel\")"), 2:"Yes" ("T button name (\"OK\")")) -> (T button?=w342:bool)
            n122 = case shown="False" w342 {
              tunnel: w336 -> [_ w344]
              tunnel: [w343 w344] -> w335
              frame False {
                n123 = call "Prompt User for Flight Number"() -> ("Flight Number CXXX"=w343:string)  [unwired: 17 in, 2 out]
              }
              frame True {
              }
            }
          }
          frame #1 {
            n124 = Two Button Dialog(message="Get FGGA Files\nof Today's Date?", 1:"No" ("F button name (\"Cancel\")"), 2:"Yes" ("T button name (\"OK\")")) -> (T button?=w351:bool)
            n125 = case shown="False" w351 {
              selector: w351 -> [w353 w354]
              tunnel: [w353 w354] -> w345
              tunnel: [w352 _] -> w346
              frame False {
                n126 = call "Prompt User for Date"() -> ("Date"=w352:string)  [unwired: 17 in, 2 out]
              }
              frame True {
              }
            }
          }
          frame #2 {
            n127 = Build Path(base path=path "\\\\192.168.101.180\\flt_folders" ("path"), name or relative path=w357) -> (appended path=w362:path)
            n128 = Concatenate Strings(w357, "_" ("string"), "corechem" ("string")) -> (w361:string)
            n129 = Build Path(base path=w362, name or relative path=w361) -> (appended path=w355:path)
            n130 = Create Folder(path (use dialog)=w355) -> (error out=→"Create folder error out":errorcluster)  [unwired: 2 in, 2 out]
            n131 = call "labSSH_FGGA_Files_Transfer.vi"("Flight_num"=w357, "Get current?"=w358, "Date"=w356, "Flight Folder Path"=w355) -> ("error IO"=→"FGGA File Transfer Error out":errorcluster)  [unwired: 11 in]
          }
          frame #3 {
            n132 = local write "Transfer OLD FGGA Files"(FALSE) -> ()
          }
        }
      }
      event "Transfer NEW FGGA Files": Value Change {
        n133 = event-data() -> ()  [unwired: 1 in, 6 out]
        n134 = flat-sequence {
          tunnel: [w371] -> w370
          tunnel: w370 -> [w383]
          tunnel: [w383] -> w369
          tunnel: [w382] -> w368
          tunnel: [w381] -> w367
          tunnel: w369 -> [w393]
          tunnel: w368 -> [w392]
          tunnel: w367 -> [w394]
          frame #0 {
            n135 = local read "Flight Number"() -> (w372:string)
            n136 = Concatenate Strings("Confirm Flight Number" ("message"), "\n", w372) -> (w374:string)
            n137 = Two Button Dialog(message=w374, 1:"No" ("F button name (\"Cancel\")"), 2:"Yes" ("T button name (\"OK\")")) -> (T button?=w378:bool)
            n138 = case shown="False" w378 {
              tunnel: w372 -> [_ w380]
              tunnel: [w379 w380] -> w371
              frame False {
                n139 = call "Prompt User for Flight Number3"() -> ("Flight Number CXXX"=w379:string)  [unwired: 17 in, 2 out]
              }
              frame True {
              }
            }
          }
          frame #1 {
            n140 = Two Button Dialog(message="Get FGGA Files\nof Today's Date?", 1:"No" ("F button name (\"Cancel\")"), 2:"Yes" ("T button name (\"OK\")")) -> (T button?=w387:bool)
            n141 = case shown="False" w387 {
              selector: w387 -> [w389 w390]
              tunnel: [w389 w390] -> w381
              tunnel: [w388 _] -> w382
              frame False {
                n142 = call "Prompt User for Date2"() -> ("Date"=w388:string)  [unwired: 17 in, 2 out]
              }
              frame True {
              }
            }
          }
          frame #2 {
            n143 = Build Path(base path=path "\\\\192.168.101.180\\flt_folders" ("path"), name or relative path=w393) -> (appended path=w398:path)
            n144 = Concatenate Strings(w393, "_" ("string"), "corechem" ("string")) -> (w397:string)
            n145 = Build Path(base path=w398, name or relative path=w397) -> (appended path=w391:path)
            n146 = Create Folder(path (use dialog)=w391) -> (error out=→"Create folder error out 3":errorcluster)  [unwired: 2 in, 2 out]
            n147 = call "labSSH_new_FGGA_Files_Transfer.vi"("Flight_num"=w393, "Get current?"=w394, "Date"=w392, "Flight Folder Path"=w391) -> ("error IO"=→"FGGA File Transfer Error out 2":errorcluster)  [unwired: 11 in]
          }
          frame #3 {
            n148 = local write "Transfer NEW FGGA Files"(FALSE) -> ()
          }
        }
      }
      event "OLD\nFGGA Restart": Value Change {
        n149 = event-data() -> ()  [unwired: 1 in, 6 out]
        n150 = flat-sequence {
          frame #0 {
            n151 = Two Button Dialog(message="FGGA will be restarted,\nARE YOU SURE?") -> (T button?=w404:bool)  [unwired: 2 in]
            n152 = case shown="True" w404 {
              frame False {
              }
              frame True {
                n153 = call "labSSH_Commands.vi"("Data"="reboot", "New_FGGA=T\nOld_FGGA=F"=FALSE ("New_FGGA=T\nOld_FGGA=F")) -> ()  [unwired: 13 in, 1 out]
              }
            }
          }
          frame #1 {
            n154 = local write "OLD\nFGGA Restart"(FALSE ("FGGA Restart")) -> ()
          }
        }
      }
      event "NEW\nFGGA Restart": Value Change {
        n155 = event-data() -> ()  [unwired: 1 in, 6 out]
        n156 = flat-sequence {
          frame #0 {
            n157 = Two Button Dialog(message="FGGA will be restarted,\nARE YOU SURE?") -> (T button?=w409:bool)  [unwired: 2 in]
            n158 = case shown="True" w409 {
              frame False {
              }
              frame True {
                n159 = call "labSSH_Commands.vi"("Data"="sudo -i reboot", "New_FGGA=T\nOld_FGGA=F"=TRUE ("New_FGGA=T\nOld_FGGA=F")) -> ()  [unwired: 13 in, 1 out]
              }
            }
          }
          frame #1 {
            n160 = local write "NEW\nFGGA Restart"(FALSE ("FGGA Restart")) -> ()
          }
        }
      }
      event "OLD FGGA Shutdown": Value Change {
        n161 = event-data() -> ()  [unwired: 1 in, 6 out]
        n162 = flat-sequence {
          frame #0 {
            n163 = Two Button Dialog(message="FGGA will be shutdown,\nARE YOU SURE?") -> (T button?=w414:bool)  [unwired: 2 in]
            n164 = case shown="True" w414 {
              frame False {
              }
              frame True {
                n165 = call "labSSH_Commands.vi"("Data"="halt", "New_FGGA=T\nOld_FGGA=F"=FALSE ("New_FGGA=T\nOld_FGGA=F")) -> ()  [unwired: 13 in, 1 out]
              }
            }
          }
          frame #1 {
            n166 = local write "OLD FGGA Shutdown"(FALSE ("FGGA Restart")) -> ()
          }
        }
      }
      event "NEW FGGA Shutdown": Value Change {
        n167 = event-data() -> ()  [unwired: 1 in, 6 out]
        n168 = flat-sequence {
          frame #0 {
            n169 = Two Button Dialog(message="FGGA will be shutdown,\nARE YOU SURE?") -> (T button?=w419:bool)  [unwired: 2 in]
            n170 = case shown="True" w419 {
              frame False {
              }
              frame True {
                n171 = call "labSSH_Commands.vi"("Data"="sudo -i halt", "New_FGGA=T\nOld_FGGA=F"=TRUE ("New_FGGA=T\nOld_FGGA=F")) -> ()  [unwired: 13 in, 1 out]
              }
            }
          }
          frame #1 {
            n172 = local write "NEW FGGA Shutdown"(FALSE ("FGGA Restart")) -> ()
          }
        }
      }
    }
    n173 = node-c288() -> ()  [unwired: 1 in, 1 out]
  }
  n174 = local write "Network disconnected"(FALSE ("Network disconnect")) -> ()
  n175 = while {
    shift-right: [w544] -> _
    shift-left: w22 -> [w542]
    shift-right: [w546] -> _
    shift-left: w21 -> [w547]
    shift-right: [w545] -> _
    shift-left: w23 -> [w549]
    shift-right: [w538] -> _
    shift-left: w23 -> [w540]
    shift-right: [w535] -> _
    shift-left: w22 -> [w534]
    shift-right: [w537] -> _
    shift-left: w21 -> [w539]
    stop <- FALSE stop-if-true
    w487 = ""
    w482 = "%s" ("format string")
    w666 = "%s" ("format string")
    w671 = "%s" ("format string")
    w676 = "%s" ("format string")
    w682 = "%s" ("format string")
    w688 = "%s" ("format string")
    w692 = "%s" ("format string")
    # "UDP Data Processing"
    n176 = local read "CHFGGA01"() -> (w695:string)
    n177 = local read "TWBOZO01"() -> (w670:string)
    n178 = local read "AL52CO01"() -> (w687:string)
    n179 = local read "CABOZO01"() -> (w675:string)
    n180 = local read "TEIOZO01"() -> (w681:string)
    n181 = local read "CHTSOO01"() -> (w665:string)
    n182 = local read "Ambient = OFF\nCabin = ON"() -> (w570:bool)
    n183 = Spreadsheet String To Array(delimiter (Tab)=",", format string=w692, spreadsheet string=w695, array type (2D Dbl)=string[] []) -> (array=w642:string[])
    n184 = Spreadsheet String To Array(delimiter (Tab)=",", format string=w688, spreadsheet string=w687, array type (2D Dbl)=string[] []) -> (array=w663:string[])
    n185 = Spreadsheet String To Array(delimiter (Tab)=",", format string=w676, spreadsheet string=w675, array type (2D Dbl)=string[] []) -> (array=w567:string[])
    n186 = Spreadsheet String To Array(delimiter (Tab)=",", format string=w682, spreadsheet string=w681, array type (2D Dbl)=string[] []) -> (array=w640:string[])
    n187 = Spreadsheet String To Array(delimiter (Tab)=",", format string=w671, spreadsheet string=w670, array type (2D Dbl)=string[] []) -> (array=w566:string[])
    n188 = Spreadsheet String To Array(delimiter (Tab)=",", format string=w666, spreadsheet string=w665, array type (2D Dbl)=string[] []) -> (array=w638:string[])
    n189 = Array To Spreadsheet String(delimiter (Tab)="\r", array=w642, 3:w692) -> (spreadsheet string=→"FGGA":string)
    n190 = Array To Spreadsheet String(delimiter (Tab)="\r", array=w663, 3:w688) -> (spreadsheet string=→"CO":string)
    n191 = Array To Spreadsheet String(delimiter (Tab)="\r", array=w567, 3:w676) -> (spreadsheet string=→"2B Cabin Ozone":string)
    n192 = Array To Spreadsheet String(delimiter (Tab)="\r", array=w640, 3:w682) -> (spreadsheet string=→"TEi49 Ozone":string)
    n193 = Array To Spreadsheet String(delimiter (Tab)="\r", array=w566, 3:w671) -> (spreadsheet string=→"2B Ambient Ozone":string)
    n194 = Array To Spreadsheet String(delimiter (Tab)="\r", array=w638, 3:w666) -> (spreadsheet string=→"SO2":string)
    n195 = Select(t=w567, s=w570, f=w566) -> (s? t:f=w565:string[])
    n196 = Index Array(array=w638, index #1=6 ("index"), index #2=4 ("index"), index #3=3 ("index"), index #4=7 ("index"), index #5=8 ("index"), index #6=15 ("index"), index #7=24 ("index"), index #8=29 ("index"), index #9=36 ("index"), index #10=37 ("index"), index #11=38 ("index"), index #12=39 ("index"), index #13=48 ("index"), index #14=14 ("index")) -> (element #1=w557:string, element #2=w621:string, element #3=w616:string, element #4=w609:string, element #5=w585:string, element #6=w584:string, element #7=w505:string, element #8=w504:string, element #9=w454:string, element #10=w450:string, element #11=w446:string, element #12=w444:string, element #13=w436:string, element #14=w434:string)
    n197 = Index Array(array=w565, index #1=8 ("index"), index #2=11 ("index")) -> (element #1=w559:string, element #2=w560:string)
    n198 = Index Array(array=w640, index #1=6 ("index"), index #2=4 ("index"), index #3=3 ("index"), index #4=7 ("index"), index #5=9 ("index"), index #6=14 ("index"), index #7=15 ("index")) -> (element #1=w634:string, element #2=w622:string, element #3=w617:string, element #4=w602:string, element #5=w576:string, element #6=w575:string, element #7=w574:string)
    n199 = Scan Value(string=w559, format string="%f") -> (value=→"2B Ozone concentration":dbl)  [unwired: 1 in, 1 out]
    n200 = Scan Value(string=w560, format string="%4f") -> (value=→"2B Ozone flow rate":dbl)  [unwired: 1 in, 1 out]
    n201 = Index Array(array=w642, index #1=6 ("index"), index #2=4 ("index"), index #3=3 ("index"), index #4=7 ("index"), index #5=8 ("index"), index #6=9 ("index"), index #7=10 ("index"), index #8=17 ("index"), index #9=16 ("index"), index #10=11 ("index"), index #11=12 ("index"), index #12=21 ("index"), index #13=14 ("index"), index #14=15 ("index")) -> (element #1=w636:string, element #2=w624:string, element #3=w619:string, element #4=w604:string, element #5=w522:string, element #6=w520:string, element #7=w516:string, element #8=w515:string, element #9=w514:string, element #10=w509:string, element #11=w508:string, element #12=w497:string, element #13=w463:string, element #14=w462:string)
    n202 = Index Array(array=w663, index #1=2 ("index"), index #2=27 ("index"), index #3=28 ("index"), index #4=29 ("index"), index #5=30 ("index"), index #6=31 ("index"), index #7=6 ("index"), index #8=4 ("index"), index #9=3 ("index"), index #10=8 ("index"), index #11=14 ("index"), index #12=16 ("index"), index #13=19 ("index"), index #14=12 ("index"), index #15=13 ("index"), index #16=10 ("index"), index #17=11 ("index"), index #18=15 ("index")) -> (element #1=w532:string, element #2=w606:string, element #3=w653:string, element #4=w647:string, element #5=w645:string, element #6=w646:string, element #7=w635:string, element #8=w623:string, element #9=w618:string, element #10=w607:string, element #11=w594:string, element #12=w591:string, element #13=w590:string, element #14=w552:string, element #15=w551:string, element #16=w493:string, element #17=w474:string, element #18=w468:string)
    n203 = Scan Value(string=w436, format string="%f") -> (value=→"Calibration gas cylinder \nconcentration (ppb)":dbl)  [unwired: 1 in, 1 out]
    n204 = Scan Value(string=w505, format string="%f") -> (value=→"TEI43i MFC2 Cal Flow":dbl)  [unwired: 1 in, 1 out]
    n205 = Scan Value(string=w504, format string="%f") -> (value=→"TEI43i MFC3 Sample Flow":dbl)  [unwired: 1 in, 1 out]
    n206 = Scan Value(string=w454, format string="%f") -> (value=w440:dbl)  [unwired: 1 in, 1 out]
    n207 = Scan Value(string=w450, format string="%d", default (0 dbl)=0) -> (value=w448:i32)  [unwired: 1 out]
    n208 = Scan Value(string=w434, format string="%f") -> (value=→"SO2 react pressure":dbl)  [unwired: 1 in, 1 out]
    n209 = Scan Value(string=w444, format string="%f") -> (value=→"SO2 Sensitivity":dbl)  [unwired: 1 in, 1 out]
    n210 = Scan Value(string=w446, format string="%f") -> (value=→"SO2 Zero":dbl)  [unwired: 1 in, 1 out]
    n211 = Scan Value(string=w585, format string="%f") -> (value=w441:dbl)  [unwired: 1 in, 1 out]
    n212 = Scan Value(string=w584, format string="%f") -> (value=→"TEI43C Sample Flow":dbl)  [unwired: 1 in, 1 out]
    n213 = Not Equal To 0?(x=w448) -> (x != 0?=→"mean zero\ncal status":bool)
    n214 = Decimal String To Number(string=w532) -> (number=w530:i32)  [unwired: 2 in, 1 out]
    n215 = call "Find_Data_SubVI.vi"("FGGA"=w636, "CO"=w635, "Ozone"=w634, "SO2"=w557) -> ("Output Value"=→"CPU Total %":dbl)  [unwired: 11 in]
    n216 = call "Find_Data_SubVI.vi"("FGGA"=w624, "CO"=w623, "Ozone"=w622, "SO2"=w621) -> ("Output Value"=→"MFM":dbl)  [unwired: 11 in]
    n217 = call "Find_Data_SubVI.vi"("FGGA"=w619, "CO"=w618, "Ozone"=w617, "SO2"=w616) -> ("Output Value"=w615:dbl)  [unwired: 11 in]
    n218 = call "Find_Data_SubVI.vi"("FGGA"=w604, "CO"=w607, "Ozone"=w602, "SO2"=w609) -> ("Output Value"=→"USB Disk Space Used %":dbl)  [unwired: 11 in]
    n219 = Not Equal To 0?(x=w615) -> (x != 0?=→"PTP Sync":bool)
    n220 = Add(x=w530, y=u32 2082844800) -> (x+y=w529:u32)
    n221 = Scan Value(string=w497, format string="%f") -> (value=→"MFC1 Cal Flow":dbl)  [unwired: 1 in, 1 out]
    n222 = Scan Value(string=w463, format string="%f") -> (value=w461:dbl)  [unwired: 1 in, 1 out]
    n223 = Scan Value(string=w462, format string="%f") -> (value=w460:dbl)  [unwired: 1 in, 1 out]
    n224 = Scan Value(string=w508, format string="%f") -> (value=→"Cell temperature" →"Cell temperature 2":dbl)  [unwired: 1 in, 1 out]
    n225 = Scan Value(string=w509, format string="%f") -> (value=→"Cell pressure" →"Cell pressure 2":dbl)  [unwired: 1 in, 1 out]
    n226 = Scan Value(string=w514, format string="%f") -> (value=→"CH4 Dry" →"CH4 Dry 2":dbl)  [unwired: 1 in, 1 out]
    n227 = Scan Value(string=w515, format string="%f") -> (value=→"CO2 Dry" →"CO2 Dry 2":dbl)  [unwired: 1 in, 1 out]
    n228 = Scan Value(string=w516, format string="%f") -> (value=→"H2O" →"H2O 2":dbl)  [unwired: 1 in, 1 out]
    n229 = Scan Value(string=w520, format string="%f") -> (value=→"CO2" →"CO2 2":dbl)  [unwired: 1 in, 1 out]
    n230 = Scan Value(string=w522, format string="%f") -> (value=→"CH4" →"CH4 2":dbl)  [unwired: 1 in, 1 out]
    n231 = local read "PRTAFT_UDP_In"() -> (w480:string)
    n232 = Scan Value(string=w646, format string="%f") -> (value=→"Std\nContent (barG)":dbl)  [unwired: 1 in, 1 out]
    n233 = Scan Value(string=w606, format string="%d", default (0 dbl)=u32 0) -> (value=w660:u32)  [unwired: 1 out]
    n234 = Scan Value(string=w645, format string="%f") -> (value=→"N2\nContent (barG)":dbl)  [unwired: 1 in, 1 out]
    n235 = Scan Value(string=w647, format string="%f") -> (value=→"CO2\nContent (barG)":dbl)  [unwired: 1 in, 1 out]
    n236 = Scan Value(string=w653, format string="%f") -> (value=→"CO2 Pressure\nDelivery (PSIA)":dbl)  [unwired: 1 in, 1 out]
    n237 = Bundle(w441, w440) -> (→"TEi43i Concentration scaled / raw":cluster{dbl, dbl})  [unwired: 1 in]
    n238 = To Time Stamp(1:w529) -> (0:w533:timestamp)
    n239 = Scan Value(string=w594, format string="%f") -> (value=→"Lamp Flow Controller":dbl)  [unwired: 1 in, 1 out]
    n240 = Scan Value(string=w474, format string="%f") -> (value=→"Raw Signal":dbl)  [unwired: 1 in, 1 out]
    n241 = Scan Value(string=w468, format string="%f") -> (value=→"Lamp Temperature":dbl)  [unwired: 1 in, 1 out]
    n242 = Scan Value(string=w493, format string="%f") -> (value=→"CO Concentration":dbl)  [unwired: 1 in, 1 out]
    n243 = Scan Value(string=w591, format string="%f") -> (value=→"Monochromator Flow":dbl)  [unwired: 1 in, 1 out]
    n244 = Scan Value(string=w590, format string="%f") -> (value=→"Fluorescence Cell Pressure":dbl)  [unwired: 1 in, 1 out]
    n245 = Not Equal To 0?(x=w660) -> (x != 0?=→"CO CAL Status":bool)
    n246 = Scan Value(string=w574, format string="%f") -> (value=→"TEI49 Sample Flow B":dbl)  [unwired: 1 in, 1 out]
    n247 = Scan Value(string=w576, format string="%f") -> (value=→"TEi49 Concentration":dbl)  [unwired: 1 in, 1 out]
    n248 = Scan Value(string=w575, format string="%f") -> (value=→"TEI49 Sample Flow A":dbl)  [unwired: 1 in, 1 out]
    n249 = Scan Value(string=w552, format string="%f") -> (value=w543:dbl)  [unwired: 1 in, 1 out]
    n250 = Scan Value(string=w551, format string="%f") -> (value=w536:dbl)  [unwired: 1 in, 1 out]
    n251 = Not Equal?(x=w542, y=w543) -> (x != y?=w548:bool)
    n252 = Not Equal?(x=w534, y=w536) -> (x != y?=w541:bool)
    n253 = Spreadsheet String To Array(delimiter (Tab)=",", format string=w482, spreadsheet string=w480, array type (2D Dbl)=string[] []) -> (array=w481:string[])
    n254 = case shown="True" w548 {
      tunnel: w549 -> [w716 w725]
      tunnel: w547 -> [w717 w724]
      tunnel: [w717 w723] -> w546
      tunnel: w533 -> [_ w719]
      tunnel: w543 -> [_ w720]
      tunnel: [w716 w722] -> w545
      tunnel: [w715 w721] -> w544
      tunnel: w543 -> [_ w721]
      tunnel: w542 -> [w715 _]
      frame False {
      }
      frame True {
        n255 = Bundle(w719, w720) -> (w718:cluster{timestamp, dbl})  [unwired: 1 in]
        n256 = Replace Array Subset(array=w725, new element=w718, index=w724) -> (w722:cluster{"time stamp":timestamp, "Y":dbl}[])
        n257 = Increment(x=w724) -> (x+1=w723:i32)
      }
    }
    "CO Sensitivity" <- w545
    n258 = case shown="True" w541 {
      tunnel: w540 -> [w705 w714]
      tunnel: w539 -> [w706 w713]
      tunnel: [w706 w712] -> w537
      tunnel: w533 -> [_ w711]
      tunnel: w536 -> [_ w710]
      tunnel: [w705 w709] -> w538
      tunnel: [w704 w708] -> w535
      tunnel: w536 -> [_ w708]
      tunnel: w534 -> [w704 _]
      frame False {
      }
      frame True {
        n259 = Bundle(w711, w710) -> (w707:cluster{timestamp, dbl})  [unwired: 1 in]
        n260 = Replace Array Subset(array=w714, new element=w707, index=w713) -> (w709:cluster{"time stamp":timestamp, "Y":dbl}[])
        n261 = Increment(x=w713) -> (x+1=w712:i32)
      }
    }
    "CO Zero" <- w538
    n262 = Array To Spreadsheet String(delimiter (Tab)="\r", array=w481, 3:w482) -> (spreadsheet string=→"PRTAFT_DLU":string)
    n263 = Index Array(array=w481, index #1=5 ("index"), index #2=19 ("index")) -> (element #1=w485:string, element #2=w483:string)
    n264 = Not Equal?(x=w485, y=w487) -> (x != y?=w486:bool)
    n265 = Not Equal?(x=w483, y=w487) -> (x != y?=w484:bool)
    n266 = Bundle(w461, w460) -> (→"Ring Down Time RDA & RDB" →"Ring Down Time RDA & RDB 2":cluster{dbl, dbl})  [unwired: 1 in]
    n267 = case shown="False" w484 {
      tunnel: ["1" w701] -> w477
      tunnel: w483 -> [_ w701]
      frame False {
      }
      frame True {
      }
    }
    n268 = case shown="False" w486 {
      tunnel: ["XXXX" w703] -> w478
      tunnel: w485 -> [_ w703]
      frame False {
      }
      frame True {
      }
    }
    n269 = Wait (ms)(milliseconds to wait=u32 1000) -> ()  [unwired: 1 out]
    n270 = local write "WoW Flag"(w477) -> ()
    n271 = local write "Flight Number"(w478) -> ()
  }
  n272 = while {
    stop <- FALSE stop-if-true
    # "Check Connection with the cRIO continuously"
    n273 = node-c288() -> (w727:T6)  [unwired: 4 in]
    n274 = TCP Open Connection(address="192.168.101.17", remote port or service name=u16 7001) -> (connection ID=w736:refnum<k5>, error out=w737:errorcluster)  [unwired: 3 in]
    n275 = timed-loop {
      tunnel: w737 -> [w752]
      tunnel: w736 -> [w749]
      tunnel: [w745] -> w729
      tunnel: [w746] -> w733
      shift-right: [w741] -> _
      shift-left: FALSE -> [w742]
      timing: w727 -> [_]
      timing-out: [_] -> w726
      stop <- w745 stop-if-true
      # "Maintain live connecton to cRIO for connection watchdog"
      n276 = node-c288() -> ()  [unwired: 1 in, 1 out]
      n277 = TCP Write(connection ID=w749, data in="1", error in (no error)=w752, 9:2000 ("timeout ms (25000)")) -> (connection ID out=w750:refnum<k5>, bytes written=w747:i32, error out=w751:errorcluster)
      n278 = Select(t=FALSE, s=w742, f=TRUE) -> (s? t:f=w741:bool)
      "cRIO connection status" <- w741
      n279 = local write "Network disconnected"(FALSE ("Network disconnect")) -> ()
      n280 = TCP Read(connection ID=w750, bytes to read=w747, error in (no error)=w751, 9:2000 ("timeout ms (25000)")) -> (connection ID out=w746:refnum<k5>, error out=w745:errorcluster)  [unwired: 1 in, 1 out]
      n281 = node-c288() -> ()  [unwired: 1 in, 1 out]
    }
    n282 = node-c288(w726) -> ()  [unwired: 1 out]
    n283 = TCP Close Connection(connection ID=w733, error in (no error)=w729) -> (error out=w728:errorcluster)  [unwired: 1 in, 1 out]
    "Network Check error out" <- w728
    n284 = Unbundle By Name(w728) -> ("status"=w730:bool)
    "Network disconnected" <- w730
    n285 = case shown="True" w730 {
      frame False {
      }
      frame True {
        n286 = One Button Dialog(message="Connection to cRIO lost\nAll Calibration(s) will be terminated") -> ()  [unwired: 1 in, 1 out]
      }
    }
  }
  n287 = while {
    stop <- FALSE stop-if-true
    # "Preflight Sub VI Descriptions"
    n288 = Wait (ms)(milliseconds to wait=u32 500) -> ()  [unwired: 1 out]
    n289 = case shown="True" "Line Lock Setting Change" {
      frame False {
      }
      frame True {
        n290 = call "FGGA Linelock Settings Procedures.vi"() -> ()  [unwired: 12 in]
      }
    }
  }
  n291 = while {
    stop <- FALSE stop-if-true
    # "Postflight Sub VI Descriptions"
    n292 = case shown="True" "Postflight Procedures" {
      frame False {
      }
      frame True {
        n293 = call "PostFlight Procedures.vi"() -> ()  [unwired: 12 in]
      }
    }
    n294 = Wait (ms)(milliseconds to wait=u32 500) -> ()  [unwired: 1 out]
  }
  n295 = while {
    stop <- FALSE stop-if-true
    # "Preflight Sub VI Descriptions"
    n296 = case shown="True" "Prepare Gases" {
      frame False {
      }
      frame True {
        n297 = call "CO Gas Preparation.vi"() -> ()  [unwired: 12 in]
      }
    }
    n298 = Wait (ms)(milliseconds to wait=u32 500) -> ()  [unwired: 1 out]
  }
  n299 = while {
    stop <- FALSE stop-if-true
    # "Preflight Sub VI Descriptions"
    n300 = case shown="True" "Prepare SO2 Span Gas" {
      frame False {
      }
      frame True {
        n301 = call "SO2 Span Gas Preparation.vi"() -> ()  [unwired: 12 in]
      }
    }
    n302 = Wait (ms)(milliseconds to wait=u32 500) -> ()  [unwired: 1 out]
  }
  n303 = while {
    stop <- FALSE stop-if-true
    # "Preflight Sub VI Descriptions"
    n304 = case shown="True" "Prepare SO2 Zero Gas" {
      frame False {
      }
      frame True {
        n305 = call "SO2 ZeroAir Gas Preparation.vi"() -> ()  [unwired: 12 in]
      }
    }
    n306 = Wait (ms)(milliseconds to wait=u32 500) -> ()  [unwired: 1 out]
  }
  n307 = Obtain Queue(name (unnamed)="FGGA_Command", element data type=w67) -> (queue out=w17:refnum<queue>, error out=w16:errorcluster)  [unwired: 3 in, 1 out]
  n308 = while {
    stop <- FALSE stop-if-true
    # "Preflight Sub VI Descriptions"
    n309 = case shown="True" "CO Monitor Troubleshooting" {
      frame False {
      }
      frame True {
        n310 = call "CO Monitor Troubleshooting.vi"() -> ()  [unwired: 12 in]
      }
    }
    n311 = Wait (ms)(milliseconds to wait=u32 500) -> ()  [unwired: 1 out]
  }
  n312 = while {
    shift-right: [w779] -> _
    shift-left: u8 1 -> [w780]
    tunnel: w17 -> [w777]
    tunnel: w16 -> [w776]
    stop <- FALSE stop-if-true
    # "FGGA pump synchronise to WoW Wait on Wheel Flag"
    n313 = Wait (ms)(milliseconds to wait=u32 1000) -> ()  [unwired: 1 out]
    n314 = case shown="True" "FGGA pump\nsync to WoW" {
      tunnel: [w783 w788] -> w779
      tunnel: w780 -> [w783 w787]
      tunnel: w777 -> [_ w786]
      tunnel: w776 -> [_ w785]
      frame False {
      }
      frame True {
        n315 = local read "WoW Flag"() -> (w784:string)
        n316 = Scan Value(string=w784, format string="%d", default (0 dbl)=u8 0) -> (value=w788:u8)  [unwired: 1 out]
        n317 = Not Equal?(x=w788, y=w787) -> (x != y?=w791:bool)
        n318 = case shown="True" w791 {
          tunnel: w788 -> [_ w794]
          tunnel: w786 -> [_ w793]
          tunnel: w785 -> [_ w792]
          frame False {
          }
          frame True {
            n319 = Equal?(x=w794, y=u8 0) -> (x = y?=w799:bool)
            n320 = case shown="True" w799 {
              selector: w799 -> [w801 w802]
              tunnel: [w801 w802] -> w795
              frame False {
              }
              frame True {
              }
            }
            n321 = local write "Manual FGGA Pump"(w795) -> ()
            n322 = Bundle(cluster=T5 {"Message"="", "Message Data"=variant} ("Message Cluster"), "Message"="FGGA_pump", "Message Data"=w795) -> (w796:T5)
            n323 = Enqueue Element(queue=w793, element=w796, error in (no error)=w792) -> ()  [unwired: 1 in, 3 out]
          }
        }
      }
    }
  }
  n324 = while {
    tunnel: w17 -> [w804]
    tunnel: w16 -> [w803]
    tunnel: [w806] -> _
    tunnel: w27 -> [w805]
    stop <- FALSE stop-if-true
    # "FGGA UI Event Handler Loop"
    n325 = event shown="[14] \"Span Cal 140 Torr -  High Cal, CO Cal, Low Cal\": Value Change" {
      selector: _ -> [_ _ _ _ _ _ _ _ _ _ _ _ _ _ _ _ _ _ _ _ _ _ _ _ _ _ _]
      dyn-events: _ -> [_ _ _ _ _ _ _ _ _ _ _ _ _ _ _ _ _ _ _ _ _ _ _ _ _ _ _]
      timeout: _ -> [_ _ _ _ _ _ _ _ _ _ _ _ _ _ _ _ _ _ _ _ _ _ _ _ _ _ _]
      tunnel: w804 -> [w814 w818 w825 w832 w839 w846 w853 w860 w868 w882 w889 w904 w1031 w1322 w1594 w1984 w2059 w2125 w2179 w2242 w2312 w2368 w2493 w2759 w2877 w3128 w3135]
      tunnel: w803 -> [w813 w817 w824 w831 w838 w845 w852 w859 w867 w881 w888 w903 w1030 w1321 w1593 w1983 w2058 w2124 w2178 w2241 w2311 w2367 w2492 w2758 w2876 w3127 w3134]
      tunnel: [w808 w816 w823 w830 w837 w844 w851 w858 w866 w880 w887 w894 w1025 w1301 w1575 w1976 w2055 w2123 w2177 w2234 w2304 w2358 w2485 w2751 w2871 w3126 w3133] -> w806
      tunnel: w805 -> [_ _ _ _ _ _ _ _ _ _ _ _ _ w1312 w1586 _ _ _ _ _ _ _ _ _ _ _ _]
      event "eV1": Value Change {
        n326 = event-data() -> ("NewVal"=w811:bool)  [unwired: 1 in]
        n327 = Bundle(cluster=T5 {"Message"="", "Message Data"=variant} ("Message Cluster"), "Message"="V1", "Message Data"=w811) -> (w809:T5)
        n328 = Enqueue Element(queue=w814, element=w809, error in (no error)=w813) -> (error out=w808:errorcluster)  [unwired: 1 in, 2 out]
      }
      event "eV2": Value Change {
        n329 = event-data() -> ("NewVal"=w815:bool)  [unwired: 1 in]
        n330 = Bundle(cluster=T5 {"Message"="", "Message Data"=variant} ("Message Cluster"), "Message"="V2", "Message Data"=w815) -> (w819:T5)
        n331 = Enqueue Element(queue=w818, element=w819, error in (no error)=w817) -> (error out=w816:errorcluster)  [unwired: 1 in, 2 out]
      }
      event "eV3": Value Change {
        n332 = event-data() -> ("NewVal"=w822:bool)  [unwired: 1 in]
        n333 = Bundle(cluster=T5 {"Message"="", "Message Data"=variant} ("Message Cluster"), "Message"="V3", "Message Data"=w822) -> (w826:T5)
        n334 = Enqueue Element(queue=w825, element=w826, error in (no error)=w824) -> (error out=w823:errorcluster)  [unwired: 1 in, 2 out]
      }
      event "eV4": Value Change {
        n335 = event-data() -> ("NewVal"=w829:bool)  [unwired: 1 in]
        n336 = Bundle(cluster=T5 {"Message"="", "Message Data"=variant} ("Message Cluster"), "Message"="V4", "Message Data"=w829) -> (w833:T5)
        n337 = Enqueue Element(queue=w832, element=w833, error in (no error)=w831) -> (error out=w830:errorcluster)  [unwired: 1 in, 2 out]
      }
      event "eV10": Value Change {
        n338 = event-data() -> ("NewVal"=w836:bool)  [unwired: 1 in]
        n339 = Bundle(cluster=T5 {"Message"="", "Message Data"=variant} ("Message Cluster"), "Message"="V10", "Message Data"=w836) -> (w840:T5)
        n340 = Enqueue Element(queue=w839, element=w840, error in (no error)=w838) -> (error out=w837:errorcluster)  [unwired: 1 in, 2 out]
      }
      event "eV11": Value Change {
        n341 = event-data() -> ("NewVal"=w843:bool)  [unwired: 1 in]
        n342 = Bundle(cluster=T5 {"Message"="", "Message Data"=variant} ("Message Cluster"), "Message"="V11", "Message Data"=w843) -> (w847:T5)
        n343 = Enqueue Element(queue=w846, element=w847, error in (no error)=w845) -> (error out=w844:errorcluster)  [unwired: 1 in, 2 out]
      }
      event "eV12": Value Change {
        n344 = event-data() -> ("NewVal"=w850:bool)  [unwired: 1 in]
        n345 = Bundle(cluster=T5 {"Message"="", "Message Data"=variant} ("Message Cluster"), "Message"="V12", "Message Data"=w850) -> (w854:T5)
        n346 = Enqueue Element(queue=w853, element=w854, error in (no error)=w852) -> (error out=w851:errorcluster)  [unwired: 1 in, 2 out]
      }
      event "Manual FGGA Pump": Value Change {
        n347 = event-data() -> ("NewVal"=w857:bool)  [unwired: 1 in]
        n348 = Bundle(cluster=T5 {"Message"="", "Message Data"=variant} ("Message Cluster"), "Message"="FGGA_pump", "Message Data"=w857) -> (w861:T5)
        n349 = Enqueue Element(queue=w860, element=w861, error in (no error)=w859) -> (error out=w858:errorcluster)  [unwired: 1 in, 2 out]
      }
      event "Confirm Flight Number": Value Change {
        n350 = event-data() -> ()  [unwired: 1 in, 6 out]
        n351 = flat-sequence {
          tunnel: w867 -> [w870]
          tunnel: w868 -> [w871]
          tunnel: [w871] -> w865
          tunnel: [w870] -> w864
          tunnel: [w873] -> w866
          tunnel: w865 -> [w875]
          tunnel: w864 -> [w874]
          frame #0 {
            n352 = local write "cRIO File IO Stop\n(USB Flash Drive Unmount)"(FALSE ("cRIO File IO Stop\n(USB Flash Drive Unmount)")) -> ()
          }
          frame #1 {
            n353 = local read "Flight Number"() -> (w872:string)
            n354 = Bundle(cluster=T5 {"Message"="", "Message Data"=variant} ("Message Cluster"), "Message"="Flight Number", "Message Data"=w872) -> (w876:T5)
            n355 = Enqueue Element(queue=w875, element=w876, error in (no error)=w874) -> (error out=w873:errorcluster)  [unwired: 1 in, 2 out]
          }
        }
      }
      event "OLD\nFGGA Restart": Value Change {
        n356 = event-data() -> ("NewVal"=w879:bool)  [unwired: 1 in]
        n357 = Bundle(cluster=T5 {"Message"="", "Message Data"=variant} ("Message Cluster"), "Message"="FGGA_restart", "Message Data"=w879) -> (w883:T5)
        n358 = Enqueue Element(queue=w882, element=w883, error in (no error)=w881) -> (error out=w880:errorcluster)  [unwired: 1 in, 2 out]
      }
      event "cRIO File IO Stop\n(USB Flash Drive Unmount)": Value Change {
        n359 = event-data() -> ("NewVal"=w886:bool)  [unwired: 1 in]
        n360 = Bundle(cluster=T5 {"Message"="", "Message Data"=variant} ("Message Cluster"), "Message"="Stop File Write", "Message Data"=w886) -> (w890:T5)
        n361 = Enqueue Element(queue=w889, element=w890, error in (no error)=w888) -> (error out=w887:errorcluster)  [unwired: 1 in, 2 out]
      }
      event "High Cal": Value Change {
        n362 = event-data() -> ()  [unwired: 1 in, 1 out]
        n363 = flat-sequence {
          tunnel: w904 -> [w909]
          tunnel: w903 -> [w908]
          tunnel: [w907] -> w902
          tunnel: [w906] -> w901
          tunnel: w902 -> [w925]
          tunnel: w901 -> [w924]
          tunnel: [w922] -> w900
          tunnel: [w921] -> w899
          tunnel: [w929] -> w898
          tunnel: [w930] -> w897
          tunnel: w899 -> [w934]
          tunnel: w900 -> [w933]
          tunnel: w898 -> [w987]
          tunnel: w897 -> [w986]
          tunnel: [w984] -> w896
          tunnel: [w983] -> w895
          tunnel: w896 -> [w1001]
          tunnel: w895 -> [w1000]
          tunnel: [w998] -> w893
          tunnel: [w1006] -> w894
          tunnel: w893 -> [w1006]
          frame #0 {
            w905 = TRUE
            n364 = Cluster To Array(cluster=T11 {"Message"="V2", "Message 2"="V3", "Message 3"="V4"}) -> (array=w910:string[])
            n365 = for {
              tunnel: w910 -> [w917] mode=indexing
              tunnel: w909 -> [w916]
              tunnel: w908 -> [w915]
              tunnel: [w914] -> w907
              tunnel: [w913] -> w906
              tunnel: w905 -> [w912]
              n366 = Bundle(cluster=T5 {"Message"="", "Message Data"=variant} ("Message Cluster"), "Message"=w917, "Message Data"=w912) -> (w919:T5)
              n367 = Enqueue Element(queue=w916, element=w919, error in (no error)=w915) -> (queue out=w914:refnum<queue>, error out=w913:errorcluster)  [unwired: 1 in, 1 out]
            }
            n368 = local write "eV2"(w905) -> ()
            n369 = local write "eV4"(w905) -> ()
            n370 = local write "eV3"(w905) -> ()
          }
          frame #1 {
            n371 = local read "MFC_1 User Set Value"() -> (w920:dbl)
            n372 = local write "MFC_1\nSLPM Value"(w920) -> ()
            n373 = Bundle(cluster=T5 {"Message"="", "Message Data"=variant} ("Message Cluster"), "Message"="MFC_1", "Message Data"=w920) -> (w923:T5)
            n374 = Enqueue Element(queue=w925, element=w923, error in (no error)=w924) -> (queue out=w922:refnum<queue>, error out=w921:errorcluster)  [unwired: 1 in, 1 out]
          }
          frame #2 {
            n375 = for {
              N: 45 -> [w977]
              tunnel: w934 -> [w967]
              tunnel: w933 -> [w968]
              tunnel: [w968] -> w932
              tunnel: [w967] -> w931
              tunnel: [w966] -> w928
              i -> [w976]
              stop <- w966 stop-if-true
              n376 = Subtract(x=w977, y=w976) -> (x-y=w975:i32)
              n377 = Decrement(x=w975) -> (x-1=w974:i32)
              n378 = local read "FGGA Calibration Abort"() -> (w971:bool)
              n379 = case shown="True" w971 {
                selector: w971 -> [w980 _]
                tunnel: [w980 w981] -> w969
                frame False {
                }
                frame True {
                  n380 = Two Button Dialog(message="Are you sure to abort FGGA High Cal?") -> (T button?=w981:bool)  [unwired: 2 in]
                }
              }
              n381 = Wait (ms)(milliseconds to wait=u32 1000) -> ()  [unwired: 1 out]
              n382 = local read "Network disconnected"() -> (w970:bool)
              n383 = Or(x=w970, y=w969) -> (x .or. y?=w966:bool)
              n384 = Select(t=0, s=w966, f=w974) -> (s? t:f=→"High Cal\nFlush Time Remain (sec)":i32)
              n385 = case shown="False" w969 {
                selector: w969 -> [w979 _]
                frame False {
                  n386 = local write "FGGA Calibration Abort"(w979) -> ()
                }
                frame True {
                }
              }
            }
            n387 = case shown="False" w928 {
              tunnel: w932 -> [w941 w965]
              tunnel: w931 -> [w940 w964]
              tunnel: [w937 w964] -> w930
              tunnel: [w936 w965] -> w929
              frame False {
                w942 = TRUE
                # "Carry on if connection to cRIO is made\nor calibration not abort"
                n388 = Bundle(cluster=T5 {"Message"="", "Message Data"=variant} ("Message Cluster"), "Message"="V1", "Message Data"=w942) -> (w943:T5)
                n389 = local write "eV1"(w942) -> ()
                n390 = Enqueue Element(queue=w941, element=w943, error in (no error)=w940) -> (queue out=w938:refnum<queue>, error out=w939:errorcluster)  [unwired: 1 in, 1 out]
                n391 = for {
                  N: 60 -> [w958]
                  tunnel: w939 -> [w948]
                  tunnel: w938 -> [w947]
                  tunnel: [w948] -> w937
                  tunnel: [w947] -> w936
                  i -> [w957]
                  stop <- w949 stop-if-true
                  n392 = local read "FGGA Calibration Abort"() -> (w952:bool)
                  n393 = Subtract(x=w958, y=w957) -> (x-y=w956:i32)
                  n394 = local read "Network disconnected"() -> (w951:bool)
                  n395 = Wait (ms)(milliseconds to wait=u32 1000) -> ()  [unwired: 1 out]
                  n396 = Decrement(x=w956) -> (x-1=w953:i32)
                  n397 = case shown="True" w952 {
                    selector: w952 -> [w961 _]
                    tunnel: [w961 w962] -> w950
                    frame False {
                    }
                    frame True {
                      n398 = Two Button Dialog(message="Are you sure to abort FGGA High Cal?") -> (T button?=w962:bool)  [unwired: 2 in]
                    }
                  }
                  n399 = Or(x=w951, y=w950) -> (x .or. y?=w949:bool)
                  n400 = case shown="False" w950 {
                    selector: w950 -> [w960 _]
                    frame False {
                      n401 = local write "FGGA Calibration Abort"(w960) -> ()
                    }
                    frame True {
                    }
                  }
                  n402 = Select(t=0, s=w949, f=w953) -> (s? t:f=→"High Cal\nCal Time Remain (sec)":i32)
                }
              }
              frame True {
              }
            }
          }
          frame #3 {
            w985 = FALSE
            n403 = Cluster To Array(cluster=T12 {"Message"="V2", "Message 2"="V3", "Message 3"="V4", "Message 4"="V1"}) -> (array=w988:string[])
            n404 = for {
              tunnel: w988 -> [w995] mode=indexing
              tunnel: [w994] -> w984
              tunnel: [w993] -> w983
              tunnel: w985 -> [w992]
              tunnel: w987 -> [w991]
              tunnel: w986 -> [w990]
              n405 = Bundle(cluster=T5 {"Message"="", "Message Data"=variant} ("Message Cluster"), "Message"=w995, "Message Data"=w992) -> (w997:T5)
              n406 = Enqueue Element(queue=w991, element=w997, error in (no error)=w990) -> (queue out=w994:refnum<queue>, error out=w993:errorcluster)  [unwired: 1 in, 1 out]
            }
            n407 = local write "eV2"(w985) -> ()
            n408 = local write "eV4"(w985) -> ()
            n409 = local write "eV3"(w985) -> ()
            n410 = local write "eV1"(w985) -> ()
          }
          frame #4 {
            w999 = 0.0 ("MFC_1\nSLPM Value")
            n411 = local write "MFC_1\nSLPM Value"(w999) -> ()
            n412 = Bundle(cluster=T5 {"Message"="", "Message Data"=variant} ("Message Cluster"), "Message"="MFC_1", "Message Data"=w999) -> (w1003:T5)
            n413 = Enqueue Element(queue=w1001, element=w1003, error in (no error)=w1000) -> (error out=w998:errorcluster)  [unwired: 1 in, 2 out]
          }
          frame #5 {
            w1005 = FALSE ("High Cal")
            n414 = local write "High Cal"(w1005) -> ()
            n415 = local write "FGGA Calibration Abort"(w1005) -> ()
          }
        }
      }
      event "High Cal\n140 Torr": Value Change {
        n416 = event-data() -> ()  [unwired: 1 in, 1 out]
        n417 = flat-sequence {
          tunnel: w1031 -> [w1036]
          tunnel: w1030 -> [w1035]
          tunnel: [w1034] -> w1029
          tunnel: [w1033] -> w1028
          tunnel: w1029 -> [w1052]
          tunnel: w1028 -> [w1051]
          tunnel: [w1049] -> w1016
          tunnel: [w1048] -> w1017
          tunnel: w1017 -> [w1058]
          tunnel: w1016 -> [w1059]
          tunnel: [w1057] -> w1015
          tunnel: [w1056] -> w1014
          tunnel: [w1055] -> w1009
          tunnel: w1015 -> [w1082]
          tunnel: w1014 -> [w1081]
          tunnel: [w1080] -> w1013
          tunnel: [w1079] -> w1012
          tunnel: [w1078] -> w1010
          tunnel: w1009 -> [w1078]
          tunnel: w1013 -> [w1143]
          tunnel: w1012 -> [w1142]
          tunnel: [w1141] -> w1011
          tunnel: w1010 -> [w1139]
          tunnel: [w1138] -> w1008
          tunnel: [w1137] -> w1007
          tunnel: [w1165] -> w1021
          tunnel: [w1166] -> w1019
          tunnel: w1011 -> [w1164]
          tunnel: w1008 -> [w1163]
          tunnel: w1007 -> [w1162]
          tunnel: w1021 -> [w1198]
          tunnel: [w1198] -> w1020
          tunnel: w1019 -> [w1197]
          tunnel: [w1197] -> w1018
          tunnel: w1020 -> [w1203]
          tunnel: w1018 -> [w1202]
          tunnel: [w1200] -> w1027
          tunnel: [w1199] -> w1026
          tunnel: w1027 -> [w1218]
          tunnel: w1026 -> [w1217]
          tunnel: [w1215] -> w1024
          tunnel: [w1214] -> w1022
          tunnel: w1024 -> [w1224]
          tunnel: [w1223] -> w1023
          tunnel: w1022 -> [w1225]
          tunnel: [w1287] -> w1025
          tunnel: w1023 -> [w1287]
          frame #0 {
            w1032 = TRUE
            n418 = Cluster To Array(cluster=T11 {"Message"="V2", "Message 2"="V3", "Message 3"="V4"}) -> (array=w1037:string[])
            n419 = for {
              tunnel: w1037 -> [w1044] mode=indexing
              tunnel: w1036 -> [w1043]
              tunnel: w1035 -> [w1042]
              tunnel: [w1041] -> w1034
              tunnel: [w1040] -> w1033
              tunnel: w1032 -> [w1039]
              n420 = Bundle(cluster=T5 {"Message"="", "Message Data"=variant} ("Message Cluster"), "Message"=w1044, "Message Data"=w1039) -> (w1046:T5)
              n421 = Enqueue Element(queue=w1043, element=w1046, error in (no error)=w1042) -> (queue out=w1041:refnum<queue>, error out=w1040:errorcluster)  [unwired: 1 in, 1 out]
            }
            n422 = local write "eV2"(w1032) -> ()
            n423 = local write "eV4"(w1032) -> ()
            n424 = local write "eV3"(w1032) -> ()
          }
          frame #1 {
            n425 = local read "MFC_1 140 Torr\nUser Set Value"() -> (w1047:dbl)
            n426 = local write "MFC_1\nSLPM Value"(w1047) -> ()
            n427 = Bundle(cluster=T5 {"Message"="", "Message Data"=variant} ("Message Cluster"), "Message"="MFC_1", "Message Data"=w1047) -> (w1050:T5)
            n428 = Enqueue Element(queue=w1052, element=w1050, error in (no error)=w1051) -> (queue out=w1049:refnum<queue>, error out=w1048:errorcluster)  [unwired: 1 in, 1 out]
          }
          frame #2 {
            n429 = local read "Span High, High, Low, Target Cal\nFlush Start Time (seconds)"() -> (w1060:i32)
            n430 = for {
              N: w1060 -> [w1072]
              tunnel: w1058 -> [w1063]
              tunnel: w1059 -> [w1064]
              tunnel: [w1064] -> w1057
              tunnel: [w1063] -> w1056
              tunnel: [w1062] -> w1055
              i -> [w1071]
              stop <- w1062 stop-if-true
              n431 = Subtract(x=w1072, y=w1071) -> (x-y=w1070:i32)
              n432 = Decrement(x=w1070) -> (x-1=w1069:i32)
              n433 = local read "FGGA 140 Torr\nCalibration Abort"() -> (w1067:bool)
              n434 = case shown="True" w1067 {
                selector: w1067 -> [w1075 _]
                tunnel: [w1075 w1076] -> w1065
                frame False {
                }
                frame True {
                  n435 = Two Button Dialog(message="Are you sure to abort FGGA High Cal?") -> (T button?=w1076:bool)  [unwired: 2 in]
                }
              }
              n436 = Wait (ms)(milliseconds to wait=u32 1000) -> ()  [unwired: 1 out]
              n437 = local read "Network disconnected"() -> (w1066:bool)
              n438 = Or(x=w1066, y=w1065) -> (x .or. y?=w1062:bool)
              n439 = case shown="False" w1065 {
                selector: w1065 -> [w1074 _]
                frame False {
                  n440 = local write "FGGA 140 Torr\nCalibration Abort"(w1074) -> ()
                }
                frame True {
                }
              }
              n441 = Select(t=0, s=w1062, f=w1069) -> (s? t:f=→"High Cal 140 Torr\nFlush Time Remain (sec)":i32)
            }
          }
          frame #3 {
            # "High to Low Flow"
            n442 = flat-sequence {
              tunnel: w1082 -> [w1099]
              tunnel: [w1098] -> w1095
              tunnel: w1081 -> [w1097]
              tunnel: [w1096] -> w1094
              tunnel: [w1106] -> w1093
              tunnel: w1095 -> [w1106]
              tunnel: [w1105] -> w1092
              tunnel: w1094 -> [w1105]
              tunnel: w1083 -> [w1104]
              tunnel: w1093 -> [w1110]
              tunnel: [w1109] -> w1091
              tunnel: w1092 -> [w1108]
              tunnel: [w1107] -> w1090
              tunnel: [w1117] -> w1089
              tunnel: w1091 -> [w1117]
              tunnel: [w1116] -> w1088
              tunnel: w1090 -> [w1116]
              tunnel: w1083 -> [w1115]
              tunnel: w1089 -> [w1121]
              tunnel: [w1120] -> w1087
              tunnel: w1088 -> [w1119]
              tunnel: [w1118] -> w1086
              tunnel: [w1128] -> w1085
              tunnel: w1087 -> [w1128]
              tunnel: [w1127] -> w1084
              tunnel: w1086 -> [w1127]
              tunnel: w1083 -> [w1126]
              tunnel: w1085 -> [w1132]
              tunnel: [w1131] -> w1080
              tunnel: w1084 -> [w1130]
              tunnel: [w1129] -> w1079
              frame #0 {
                w1103 = FALSE
                n443 = local write "eV10"(w1103) -> ()
                n444 = Bundle(cluster=T5 {"Message"="", "Message Data"=variant} ("Message Cluster"), "Message"="V10", "Message Data"=w1103) -> (w1101:T5)
                n445 = Enqueue Element(queue=w1099, element=w1101, error in (no error)=w1097) -> (queue out=w1098:refnum<queue>, error out=w1096:errorcluster)  [unwired: 1 in, 1 out]
              }
              frame #1 {
                n446 = Wait (ms)(milliseconds to wait=w1104) -> ()  [unwired: 1 out]
              }
              frame #2 {
                w1114 = FALSE
                n447 = Bundle(cluster=T5 {"Message"="", "Message Data"=variant} ("Message Cluster"), "Message"="V12" ("Message 2"), "Message Data"=w1114) -> (w1112:T5)
                n448 = local write "eV12"(w1114) -> ()
                n449 = Enqueue Element(queue=w1110, element=w1112, error in (no error)=w1108) -> (queue out=w1109:refnum<queue>, error out=w1107:errorcluster)  [unwired: 1 in, 1 out]
              }
              frame #3 {
                n450 = Wait (ms)(milliseconds to wait=w1115) -> ()  [unwired: 1 out]
              }
              frame #4 {
                w1122 = TRUE
                n451 = local write "eV11"(w1122) -> ()
                n452 = Bundle(cluster=T5 {"Message"="", "Message Data"=variant} ("Message Cluster"), "Message"="V11" ("Message 2"), "Message Data"=w1122) -> (w1123:T5)
                n453 = Enqueue Element(queue=w1121, element=w1123, error in (no error)=w1119) -> (queue out=w1120:refnum<queue>, error out=w1118:errorcluster)  [unwired: 1 in, 1 out]
              }
              frame #5 {
                n454 = Wait (ms)(milliseconds to wait=w1126) -> ()  [unwired: 1 out]
              }
              frame #6 {
                n455 = Bundle(cluster=T5 {"Message"="", "Message Data"=variant} ("Message Cluster"), "Message"="FGGA_pump", "Message Data"=TRUE) -> (w1136:T5)
                n456 = Enqueue Element(queue=w1132, element=w1136, error in (no error)=w1130) -> (queue out=w1131:refnum<queue>, error out=w1129:errorcluster)  [unwired: 1 in, 1 out]
              }
            }
            n457 = local read "Time delay (msec) between\nvalves switching"() -> (w1083:u32)
          }
          frame #4 {
            n458 = local read "Span High, High, Low, Target  Cal\nContinue Flush Time (seconds)"() -> (w1144:i32)
            n459 = for {
              N: w1144 -> [w1156]
              tunnel: w1142 -> [w1147]
              tunnel: w1143 -> [w1148]
              tunnel: [w1148] -> w1137
              tunnel: [w1147] -> w1138
              tunnel: [w1146] -> w1140
              i -> [w1155]
              stop <- w1146 stop-if-true
              n460 = Subtract(x=w1156, y=w1155) -> (x-y=w1154:i32)
              n461 = Decrement(x=w1154) -> (x-1=w1153:i32)
              n462 = local read "FGGA 140 Torr\nCalibration Abort"() -> (w1151:bool)
              n463 = case shown="True" w1151 {
                selector: w1151 -> [w1159 _]
                tunnel: [w1159 w1160] -> w1149
                frame False {
                }
                frame True {
                  n464 = Two Button Dialog(message="Are you sure to abort FGGA High Cal?") -> (T button?=w1160:bool)  [unwired: 2 in]
                }
              }
              n465 = Wait (ms)(milliseconds to wait=u32 1000) -> ()  [unwired: 1 out]
              n466 = local read "Network disconnected"() -> (w1150:bool)
              n467 = Or(x=w1150, y=w1149) -> (x .or. y?=w1146:bool)
              n468 = case shown="False" w1149 {
                selector: w1149 -> [w1158 _]
                frame False {
                  n469 = local write "FGGA 140 Torr\nCalibration Abort"(w1158) -> ()
                }
                frame True {
                }
              }
              n470 = Select(t=0, s=w1146, f=w1153) -> (s? t:f=w1145:i32)
              n471 = local write "High Cal 140 Torr\nFlush Time Remain (sec)"(w1145) -> ()
            }
            n472 = Or(x=w1140, y=w1139) -> (x .or. y?=w1141:bool)
          }
          frame #5 {
            n473 = case shown="False" w1164 {
              tunnel: w1162 -> [w1169 w1196]
              tunnel: w1163 -> [w1168 w1195]
              tunnel: [w1177 w1195] -> w1166
              tunnel: [w1176 w1196] -> w1165
              frame False {
                w1172 = TRUE
                # "Carry on if connection to cRIO is made\nor calibration not abort"
                n474 = local read "Span High, High Low, Target\nCal Time (seconds)"() -> (w1167:i32)
                n475 = local write "eV1"(w1172) -> ()
                n476 = Bundle(cluster=T5 {"Message"="", "Message Data"=variant} ("Message Cluster"), "Message"="V1", "Message Data"=w1172) -> (w1173:T5)
                n477 = Enqueue Element(queue=w1169, element=w1173, error in (no error)=w1168) -> (queue out=w1170:refnum<queue>, error out=w1171:errorcluster)  [unwired: 1 in, 1 out]
                n478 = for {
                  N: w1167 -> [w1189]
                  tunnel: w1171 -> [w1180]
                  tunnel: w1170 -> [w1179]
                  tunnel: [w1180] -> w1177
                  tunnel: [w1179] -> w1176
                  i -> [w1188]
                  stop <- w1181 stop-if-true
                  n479 = Subtract(x=w1189, y=w1188) -> (x-y=w1187:i32)
                  n480 = local read "FGGA 140 Torr\nCalibration Abort"() -> (w1184:bool)
                  n481 = case shown="True" w1184 {
                    selector: w1184 -> [w1192 _]
                    tunnel: [w1192 w1193] -> w1182
                    frame False {
                    }
                    frame True {
                      n482 = Two Button Dialog(message="Are you sure to abort FGGA High Cal?") -> (T button?=w1193:bool)  [unwired: 2 in]
                    }
                  }
                  n483 = local read "Network disconnected"() -> (w1183:bool)
                  n484 = Wait (ms)(milliseconds to wait=u32 1000) -> ()  [unwired: 1 out]
                  n485 = Decrement(x=w1187) -> (x-1=w1185:i32)
                  n486 = Or(x=w1183, y=w1182) -> (x .or. y?=w1181:bool)
                  n487 = case shown="False" w1182 {
                    selector: w1182 -> [w1191 _]
                    frame False {
                      n488 = local write "FGGA 140 Torr\nCalibration Abort"(w1191) -> ()
                    }
                    frame True {
                    }
                  }
                  n489 = Select(t=0, s=w1181, f=w1185) -> (s? t:f=→"High Cal 140 Torr\nCal Time Remain (sec)":i32)
                }
              }
              frame True {
              }
            }
          }
          frame #6 {
          }
          frame #7 {
            w1201 = FALSE
            n490 = Cluster To Array(cluster=T12 {"Message"="V2", "Message 2"="V3", "Message 3"="V4", "Message 4"="V1"}) -> (array=w1204:string[])
            n491 = for {
              tunnel: w1204 -> [w1211] mode=indexing
              tunnel: [w1210] -> w1200
              tunnel: [w1209] -> w1199
              tunnel: w1201 -> [w1208]
              tunnel: w1203 -> [w1207]
              tunnel: w1202 -> [w1206]
              n492 = Bundle(cluster=T5 {"Message"="", "Message Data"=variant} ("Message Cluster"), "Message"=w1211, "Message Data"=w1208) -> (w1213:T5)
              n493 = Enqueue Element(queue=w1207, element=w1213, error in (no error)=w1206) -> (queue out=w1210:refnum<queue>, error out=w1209:errorcluster)  [unwired: 1 in, 1 out]
            }
            n494 = local write "eV2"(w1201) -> ()
            n495 = local write "eV4"(w1201) -> ()
            n496 = local write "eV3"(w1201) -> ()
            n497 = local write "eV1"(w1201) -> ()
          }
          frame #8 {
            w1216 = 0.0 ("MFC_1\nSLPM Value")
            n498 = local write "MFC_1\nSLPM Value"(w1216) -> ()
            n499 = Bundle(cluster=T5 {"Message"="", "Message Data"=variant} ("Message Cluster"), "Message"="MFC_1", "Message Data"=w1216) -> (w1220:T5)
            n500 = Enqueue Element(queue=w1218, element=w1220, error in (no error)=w1217) -> (queue out=w1214:refnum<queue>, error out=w1215:errorcluster)  [unwired: 1 in, 1 out]
          }
          frame #9 {
            # "Set back to high flow only if High Flow master switch is ON"
            n501 = local read "Time delay (msec) between\nvalves switching"() -> (w1222:u32)
            n502 = local read "HIGH FLOW MASTER SWITCH"() -> (w1226:bool)
            n503 = case shown="True" w1226 {
              tunnel: w1225 -> [_ w1245]
              tunnel: w1224 -> [w1227 w1238]
              tunnel: [w1227 w1231] -> w1223
              tunnel: w1222 -> [_ w1230]
              tunnel: w1222 -> [_ w1229]
              tunnel: w1222 -> [_ w1228]
              frame False {
              }
              frame True {
                n504 = flat-sequence {
                  tunnel: w1245 -> [w1249]
                  tunnel: [w1248] -> w1243
                  tunnel: w1238 -> [w1247]
                  tunnel: [w1246] -> w1236
                  tunnel: [w1256] -> w1244
                  tunnel: w1243 -> [w1256]
                  tunnel: [w1255] -> w1237
                  tunnel: w1236 -> [w1255]
                  tunnel: w1230 -> [w1254]
                  tunnel: w1244 -> [w1260]
                  tunnel: [w1259] -> w1241
                  tunnel: w1237 -> [w1258]
                  tunnel: [w1257] -> w1234
                  tunnel: [w1267] -> w1242
                  tunnel: w1241 -> [w1267]
                  tunnel: [w1266] -> w1235
                  tunnel: w1234 -> [w1266]
                  tunnel: w1229 -> [w1265]
                  tunnel: w1242 -> [w1271]
                  tunnel: [w1270] -> w1239
                  tunnel: w1235 -> [w1269]
                  tunnel: [w1268] -> w1232
                  tunnel: [w1278] -> w1240
                  tunnel: w1239 -> [w1278]
                  tunnel: [w1277] -> w1233
                  tunnel: w1232 -> [w1277]
                  tunnel: w1228 -> [w1276]
                  tunnel: w1240 -> [w1281]
                  tunnel: w1233 -> [w1280]
                  tunnel: [w1279] -> w1231
                  frame #0 {
                    n505 = Bundle(cluster=T5 {"Message"="", "Message Data"=variant} ("Message Cluster"), "Message"="FGGA_pump", "Message Data"=FALSE) -> (w1250:T5)
                    n506 = Enqueue Element(queue=w1249, element=w1250, error in (no error)=w1247) -> (queue out=w1248:refnum<queue>, error out=w1246:errorcluster)  [unwired: 1 in, 1 out]
                  }
                  frame #1 {
                    n507 = Wait (ms)(milliseconds to wait=w1254) -> ()  [unwired: 1 out]
                  }
                  frame #2 {
                    w1264 = FALSE
                    n508 = local write "eV11"(w1264) -> ()
                    n509 = Bundle(cluster=T5 {"Message"="", "Message Data"=variant} ("Message Cluster"), "Message"="V11" ("Message 2"), "Message Data"=w1264) -> (w1263:T5)
                    n510 = Enqueue Element(queue=w1260, element=w1263, error in (no error)=w1258) -> (queue out=w1259:refnum<queue>, error out=w1257:errorcluster)  [unwired: 1 in, 1 out]
                  }
                  frame #3 {
                    n511 = Wait (ms)(milliseconds to wait=w1265) -> ()  [unwired: 1 out]
                  }
                  frame #4 {
                    w1272 = TRUE
                    n512 = Bundle(cluster=T5 {"Message"="", "Message Data"=variant} ("Message Cluster"), "Message"="V12" ("Message 2"), "Message Data"=w1272) -> (w1275:T5)
                    n513 = local write "eV12"(w1272) -> ()
                    n514 = Enqueue Element(queue=w1271, element=w1275, error in (no error)=w1269) -> (queue out=w1270:refnum<queue>, error out=w1268:errorcluster)  [unwired: 1 in, 1 out]
                  }
                  frame #5 {
                    n515 = Wait (ms)(milliseconds to wait=w1276) -> ()  [unwired: 1 out]
                  }
                  frame #6 {
                    w1282 = TRUE
                    n516 = local write "eV10"(w1282) -> ()
                    n517 = Bundle(cluster=T5 {"Message"="", "Message Data"=variant} ("Message Cluster"), "Message"="V10", "Message Data"=w1282) -> (w1285:T5)
                    n518 = Enqueue Element(queue=w1281, element=w1285, error in (no error)=w1280) -> (error out=w1279:errorcluster)  [unwired: 1 in, 2 out]
                  }
                }
              }
            }
          }
          frame #10 {
            w1286 = FALSE ("High Cal")
            n519 = local write "High Cal\n140 Torr"(w1286) -> ()
            n520 = local write "FGGA 140 Torr\nCalibration Abort"(w1286) -> ()
          }
        }
      }
      event "Span Cal - \nHigh Cal, CO Cal, Low Cal": Value Change {
        n521 = event-data() -> ()  [unwired: 1 in, 1 out]
        n522 = flat-sequence {
          tunnel: w1322 -> [w1328]
          tunnel: w1321 -> [w1327]
          tunnel: [w1326] -> w1320
          tunnel: [w1325] -> w1319
          tunnel: w1320 -> [w1344]
          tunnel: w1319 -> [w1343]
          tunnel: [w1341] -> w1317
          tunnel: [w1340] -> w1315
          tunnel: [w1350] -> w1318
          tunnel: w1317 -> [w1350]
          tunnel: [w1349] -> w1316
          tunnel: w1315 -> [w1349]
          tunnel: [w1347] -> w1300
          tunnel: [w1347] -> w1297
          tunnel: w1318 -> [w1368]
          tunnel: w1316 -> [w1369]
          tunnel: [w1369] -> w1307
          tunnel: w1312 -> [w1370]
          tunnel: [w1370] -> w1305
          tunnel: [w1368] -> w1303
          tunnel: w1300 -> [w1367]
          tunnel: [w1366] -> w1298
          tunnel: w1297 -> [w1366]
          tunnel: w1307 -> [w1380]
          tunnel: [w1380] -> w1306
          tunnel: w1305 -> [w1379]
          tunnel: [w1379] -> w1304
          tunnel: w1303 -> [w1377]
          tunnel: [w1377] -> w1302
          tunnel: [w1376] -> w1299
          tunnel: w1298 -> [w1376]
          tunnel: [w1384] -> w1314
          tunnel: [w1383] -> w1313
          tunnel: w1302 -> [w1385]
          tunnel: w1304 -> [w1391]
          tunnel: w1306 -> [w1386]
          tunnel: w1299 -> [w1382]
          tunnel: [w1382] -> w1295
          tunnel: [w1381] -> w1294
          tunnel: w1314 -> [w1430]
          tunnel: w1313 -> [w1429]
          tunnel: [w1427] -> w1293
          tunnel: w1295 -> [w1427]
          tunnel: [w1426] -> w1292
          tunnel: w1294 -> [w1426]
          tunnel: [w1425] -> w1290
          tunnel: [w1424] -> w1288
          tunnel: [w1445] -> w1296
          tunnel: w1293 -> [w1444]
          tunnel: w1292 -> [w1443]
          tunnel: [w1442] -> w1291
          tunnel: w1290 -> [w1442]
          tunnel: [w1441] -> w1289
          tunnel: w1288 -> [w1441]
          tunnel: [w1451] -> w1311
          tunnel: [w1450] -> w1310
          tunnel: w1296 -> [w1449]
          tunnel: w1291 -> [w1448]
          tunnel: w1289 -> [w1447]
          tunnel: w1311 -> [w1533]
          tunnel: w1310 -> [w1532]
          tunnel: [w1530] -> w1309
          tunnel: [w1529] -> w1308
          tunnel: w1309 -> [w1548]
          tunnel: w1308 -> [w1547]
          tunnel: [w1545] -> w1301
          frame #0 {
            w1324 = TRUE
            n523 = Cluster To Array(cluster=T11 {"Message"="V2", "Message 2"="V3", "Message 3"="V4"}) -> (array=w1329:string[])
            n524 = for {
              tunnel: w1329 -> [w1336] mode=indexing
              tunnel: w1328 -> [w1335]
              tunnel: w1327 -> [w1334]
              tunnel: [w1333] -> w1326
              tunnel: [w1332] -> w1325
              tunnel: w1324 -> [w1331]
              n525 = Bundle(cluster=T5 {"Message"="", "Message Data"=variant} ("Message Cluster"), "Message"=w1336, "Message Data"=w1331) -> (w1338:T5)
              n526 = Enqueue Element(queue=w1335, element=w1338, error in (no error)=w1334) -> (queue out=w1333:refnum<queue>, error out=w1332:errorcluster)  [unwired: 1 in, 1 out]
            }
            n527 = local write "High Cal"(TRUE ("High Cal")) -> ()
            n528 = local write "eV2"(w1324) -> ()
            n529 = local write "eV4"(w1324) -> ()
            n530 = local write "eV3"(w1324) -> ()
          }
          frame #1 {
            n531 = local read "MFC_1 User Set Value"() -> (w1339:dbl)
            n532 = local write "MFC_1\nSLPM Value"(w1339) -> ()
            n533 = Bundle(cluster=T5 {"Message"="", "Message Data"=variant} ("Message Cluster"), "Message"="MFC_1", "Message Data"=w1339) -> (w1342:T5)
            n534 = Enqueue Element(queue=w1344, element=w1342, error in (no error)=w1343) -> (queue out=w1341:refnum<queue>, error out=w1340:errorcluster)  [unwired: 1 in, 1 out]
          }
          frame #2 {
            n535 = for {
              N: 45 -> [w1360]
              tunnel: [w1352] -> w1347
              i -> [w1359]
              stop <- w1352 stop-if-true
              n536 = local read "FGGA Calibration Abort"() -> (w1353:bool)
              n537 = case shown="True" w1353 {
                selector: w1353 -> [w1363 _]
                tunnel: [w1363 w1364] -> w1351
                frame False {
                }
                frame True {
                  n538 = Two Button Dialog(message="Are you sure to abort FGGA Span Cal?") -> (T button?=w1364:bool)  [unwired: 2 in]
                }
              }
              n539 = local read "Network disconnected"() -> (w1354:bool)
              n540 = Subtract(x=w1360, y=w1359) -> (x-y=w1358:i32)
              n541 = Decrement(x=w1358) -> (x-1=w1356:i32)
              n542 = Wait (ms)(milliseconds to wait=u32 1000) -> ()  [unwired: 1 out]
              n543 = Or(x=w1354, y=w1351) -> (x .or. y?=w1352:bool)
              n544 = case shown="False" w1351 {
                selector: w1351 -> [w1362 _]
                frame False {
                  n545 = local write "FGGA Calibration Abort"(w1362) -> ()
                }
                frame True {
                }
              }
              n546 = Select(t=0, s=w1352, f=w1356) -> (s? t:f=w1355:i32)
              n547 = local write "High Cal\nFlush Time Remain (sec)"(w1355) -> ()
            }
          }
          frame #3 {
            n548 = case shown="False" w1367 {
              tunnel: w1370 -> [w1371 _]
              frame False {
                # "CO Cal if no network\ndisconnect or abort cal"
                n549 = Bundle(cluster=T5 {"Message"="", "Message Data"=variant} ("Message Cluster"), "Message"="CO CAL", "Message Data"=TRUE) -> (w1373:T5)
                n550 = Enqueue Element(queue=w1371, element=w1373) -> ()  [unwired: 2 in, 3 out]
              }
              frame True {
              }
            }
          }
          frame #4 {
            # "To Ensure\nCO CAL\nis certain"
            n551 = Wait (ms)(milliseconds to wait=u32 1000) -> ()  [unwired: 1 out]
          }
          frame #5 {
            n552 = Bundle(cluster=T5 {"Message"="", "Message Data"=variant} ("Message Cluster"), "Message"="CO CAL", "Message Data"=FALSE) -> (w1387:T5)
            n553 = Enqueue Element(queue=w1391, element=w1387) -> ()  [unwired: 2 in, 3 out]
            n554 = case shown="False" w1382 {
              selector: w1382 -> [_ w1421]
              tunnel: w1386 -> [w1398 w1422]
              tunnel: w1385 -> [w1397 w1423]
              tunnel: [w1394 w1423] -> w1384
              tunnel: [w1393 w1422] -> w1383
              tunnel: [w1392 w1421] -> w1381
              frame False {
                w1402 = TRUE
                # "Carry on if connection to cRIO is made\nor calibration not abort"
                n555 = Bundle(cluster=T5 {"Message"="", "Message Data"=variant} ("Message Cluster"), "Message"="V1", "Message Data"=w1402) -> (w1401:T5)
                n556 = local write "eV1"(w1402) -> ()
                n557 = Enqueue Element(queue=w1397, element=w1401, error in (no error)=w1398) -> (queue out=w1396:refnum<queue>, error out=w1395:errorcluster)  [unwired: 1 in, 1 out]
                n558 = for {
                  N: 60 -> [w1415]
                  tunnel: w1396 -> [w1406]
                  tunnel: w1395 -> [w1405]
                  tunnel: [w1406] -> w1394
                  tunnel: [w1405] -> w1393
                  tunnel: [w1404] -> w1392
                  i -> [w1414]
                  stop <- w1404 stop-if-true
                  n559 = local read "FGGA Calibration Abort"() -> (w1409:bool)
                  n560 = case shown="True" w1409 {
                    selector: w1409 -> [w1418 _]
                    tunnel: [w1418 w1419] -> w1407
                    frame False {
                    }
                    frame True {
                      n561 = Two Button Dialog(message="Are you sure to abort FGGA Span Cal?") -> (T button?=w1419:bool)  [unwired: 2 in]
                    }
                  }
                  n562 = Subtract(x=w1415, y=w1414) -> (x-y=w1413:i32)
                  n563 = Decrement(x=w1413) -> (x-1=w1411:i32)
                  n564 = Wait (ms)(milliseconds to wait=u32 1000) -> ()  [unwired: 1 out]
                  n565 = local read "Network disconnected"() -> (w1408:bool)
                  n566 = Or(x=w1408, y=w1407) -> (x .or. y?=w1404:bool)
                  n567 = Select(t=0, s=w1404, f=w1411) -> (s? t:f=w1410:i32)
                  n568 = local write "High Cal\nCal Time Remain (sec)"(w1410) -> ()
                  n569 = case shown="False" w1407 {
                    selector: w1407 -> [w1417 _]
                    frame False {
                      n570 = local write "FGGA Calibration Abort"(w1417) -> ()
                    }
                    frame True {
                    }
                  }
                }
              }
              frame True {
              }
            }
          }
          frame #6 {
            w1428 = FALSE
            # "Note: eV2 and MFC 1 stays ON"
            n571 = Cluster To Array(cluster=T13 {"Message 2"="V3", "Message 3"="V4", "Message 4"="V1"}) -> (array=w1431:string[])
            n572 = for {
              tunnel: w1431 -> [w1438] mode=indexing
              tunnel: [w1437] -> w1425
              tunnel: [w1436] -> w1424
              tunnel: w1428 -> [w1435]
              tunnel: w1430 -> [w1434]
              tunnel: w1429 -> [w1433]
              n573 = Bundle(cluster=T5 {"Message"="", "Message Data"=variant} ("Message Cluster"), "Message"=w1438, "Message Data"=w1435) -> (w1440:T5)
              n574 = Enqueue Element(queue=w1434, element=w1440, error in (no error)=w1433) -> (queue out=w1437:refnum<queue>, error out=w1436:errorcluster)  [unwired: 1 in, 1 out]
            }
            n575 = local write "eV3"(w1428) -> ()
            n576 = local write "eV4"(w1428) -> ()
            n577 = local write "eV1"(w1428) -> ()
          }
          frame #7 {
            n578 = local write "High Cal"(FALSE ("High Cal")) -> ()
            n579 = Or(x=w1444, y=w1443) -> (x .or. y?=w1445:bool)
          }
          frame #8 {
            n580 = case shown="False" w1449 {
              tunnel: [w1456 w1527] -> w1451
              tunnel: [w1455 w1528] -> w1450
              tunnel: w1448 -> [w1453 w1527]
              tunnel: w1447 -> [w1452 w1528]
              frame False {
                w1461 = TRUE
                n581 = Cluster To Array(cluster=cluster{"Message":string, "Message 3":string} {"Message"="V2", "Message 3"="V4"}) -> (array=w1464:string[])
                n582 = local write "eV4"(w1461) -> ()
                n583 = local write "eV2"(w1461) -> ()
                n584 = for {
                  tunnel: w1464 -> [w1507] mode=indexing
                  tunnel: [w1506] -> w1465
                  tunnel: [w1505] -> w1467
                  tunnel: w1461 -> [w1504]
                  tunnel: w1453 -> [w1503]
                  tunnel: w1452 -> [w1502]
                  n585 = Bundle(cluster=T5 {"Message"="", "Message Data"=variant} ("Message Cluster"), "Message"=w1507, "Message Data"=w1504) -> (w1509:T5)
                  n586 = Enqueue Element(queue=w1503, element=w1509, error in (no error)=w1502) -> (queue out=w1506:refnum<queue>, error out=w1505:errorcluster)  [unwired: 1 in, 1 out]
                }
                n587 = local write "Low Cal"(TRUE ("Low Cal")) -> ()
                n588 = local read "MFC_1 User Set Value"() -> (w1468:dbl)
                n589 = local write "MFC_1\nSLPM Value"(w1468) -> ()
                n590 = Bundle(cluster=T5 {"Message"="", "Message Data"=variant} ("Message Cluster"), "Message"="MFC_1", "Message Data"=w1468) -> (w1469:T5)
                n591 = Enqueue Element(queue=w1465, element=w1469, error in (no error)=w1467) -> (queue out=w1460:refnum<queue>, error out=w1458:errorcluster)  [unwired: 1 in, 1 out]
                n592 = for {
                  N: 45 -> [w1521]
                  tunnel: [w1512] -> w1459
                  tunnel: w1460 -> [w1512]
                  tunnel: [w1511] -> w1457
                  tunnel: w1458 -> [w1511]
                  tunnel: [w1510] -> w1454
                  i -> [w1520]
                  stop <- w1510 stop-if-true
                  n593 = local read "FGGA Calibration Abort"() -> (w1515:bool)
                  n594 = case shown="True" w1515 {
                    selector: w1515 -> [w1524 _]
                    tunnel: [w1524 w1525] -> w1513
                    frame False {
                    }
                    frame True {
                      n595 = Two Button Dialog(message="Are you sure to abort FGGA Span Cal?") -> (T button?=w1525:bool)  [unwired: 2 in]
                    }
                  }
                  n596 = Subtract(x=w1521, y=w1520) -> (x-y=w1519:i32)
                  n597 = Decrement(x=w1519) -> (x-1=w1516:i32)
                  n598 = Wait (ms)(milliseconds to wait=u32 1000) -> ()  [unwired: 1 out]
                  n599 = local read "Network disconnected"() -> (w1514:bool)
                  n600 = Or(x=w1514, y=w1513) -> (x .or. y?=w1510:bool)
                  n601 = Select(t=0, s=w1510, f=w1516) -> (s? t:f=w1517:i32)
                  n602 = local write "Low Cal\nFlush Time Remain (sec)"(w1517) -> ()
                  n603 = case shown="False" w1513 {
                    selector: w1513 -> [w1523 _]
                    frame False {
                      n604 = local write "FGGA Calibration Abort"(w1523) -> ()
                    }
                    frame True {
                    }
                  }
                }
                n605 = case shown="False" w1454 {
                  tunnel: w1459 -> [w1477 w1501]
                  tunnel: w1457 -> [w1476 w1500]
                  tunnel: [w1474 w1501] -> w1456
                  tunnel: [w1472 w1500] -> w1455
                  frame False {
                    w1478 = TRUE
                    n606 = local write "eV1"(w1478) -> ()
                    n607 = Bundle(cluster=T5 {"Message"="", "Message Data"=variant} ("Message Cluster"), "Message"="V1", "Message Data"=w1478) -> (w1480:T5)
                    n608 = Enqueue Element(queue=w1477, element=w1480, error in (no error)=w1476) -> (queue out=w1475:refnum<queue>, error out=w1473:errorcluster)  [unwired: 1 in, 1 out]
                    n609 = for {
                      N: 60 -> [w1494]
                      tunnel: [w1484] -> w1474
                      tunnel: w1475 -> [w1484]
                      tunnel: w1473 -> [w1483]
                      tunnel: [w1483] -> w1472
                      i -> [w1493]
                      stop <- w1485 stop-if-true
                      n610 = local read "FGGA Calibration Abort"() -> (w1488:bool)
                      n611 = case shown="True" w1488 {
                        selector: w1488 -> [w1497 _]
                        tunnel: [w1497 w1498] -> w1486
                        frame False {
                        }
                        frame True {
                          n612 = Two Button Dialog(message="Are you sure to abort FGGA Span Cal?") -> (T button?=w1498:bool)  [unwired: 2 in]
                        }
                      }
                      n613 = Wait (ms)(milliseconds to wait=u32 1000) -> ()  [unwired: 1 out]
                      n614 = local read "Network disconnected"() -> (w1487:bool)
                      n615 = Subtract(x=w1494, y=w1493) -> (x-y=w1492:i32)
                      n616 = Decrement(x=w1492) -> (x-1=w1489:i32)
                      n617 = Or(x=w1487, y=w1486) -> (x .or. y?=w1485:bool)
                      n618 = Select(t=0, s=w1485, f=w1489) -> (s? t:f=w1490:i32)
                      n619 = local write "Low Cal\nCal Time Remain (sec)"(w1490) -> ()
                      n620 = case shown="False" w1486 {
                        selector: w1486 -> [w1496 _]
                        frame False {
                          n621 = local write "FGGA Calibration Abort"(w1496) -> ()
                        }
                        frame True {
                        }
                      }
                    }
                  }
                  frame True {
                    # "Ignore Cal if connection problem or abort button pressed"
                  }
                }
              }
              frame True {
                # "Ignore Cal if connection problem or abort button pressed"
              }
            }
          }
          frame #9 {
            w1531 = FALSE
            n622 = Cluster To Array(cluster=T14 {"Message"="V2", "Message 3"="V4", "Message 4"="V1"}) -> (array=w1534:string[])
            n623 = local write "eV1"(w1531) -> ()
            n624 = local write "eV2"(w1531) -> ()
            n625 = local write "eV4"(w1531) -> ()
            n626 = for {
              tunnel: w1534 -> [w1541] mode=indexing
              tunnel: [w1540] -> w1530
              tunnel: [w1539] -> w1529
              tunnel: w1531 -> [w1538]
              tunnel: w1533 -> [w1537]
              tunnel: w1532 -> [w1536]
              n627 = Bundle(cluster=T5 {"Message"="", "Message Data"=variant} ("Message Cluster"), "Message"=w1541, "Message Data"=w1538) -> (w1543:T5)
              n628 = Enqueue Element(queue=w1537, element=w1543, error in (no error)=w1536) -> (queue out=w1540:refnum<queue>, error out=w1539:errorcluster)  [unwired: 1 in, 1 out]
            }
          }
          frame #10 {
            w1544 = FALSE
            w1546 = 0.0 ("MFC_1\nSLPM Value")
            n629 = local write "MFC_1\nSLPM Value"(w1546) -> ()
            n630 = local write "Span Cal - \nHigh Cal, CO Cal, Low Cal"(w1544) -> ()
            n631 = local write "FGGA Calibration Abort"(w1544) -> ()
            n632 = local write "Low Cal"(w1544) -> ()
            n633 = Bundle(cluster=T5 {"Message"="", "Message Data"=variant} ("Message Cluster"), "Message"="MFC_1", "Message Data"=w1546) -> (w1550:T5)
            n634 = Enqueue Element(queue=w1548, element=w1550, error in (no error)=w1547) -> (error out=w1545:errorcluster)  [unwired: 1 in, 2 out]
          }
        }
      }
      event "Span Cal 140 Torr - \nHigh Cal, CO Cal, Low Cal": Value Change {
        n635 = event-data() -> ()  [unwired: 1 in, 1 out]
        n636 = flat-sequence {
          tunnel: w1594 -> [w1600]
          tunnel: w1593 -> [w1599]
          tunnel: [w1598] -> w1592
          tunnel: [w1597] -> w1591
          tunnel: w1592 -> [w1616]
          tunnel: w1591 -> [w1615]
          tunnel: [w1613] -> w1590
          tunnel: [w1612] -> w1589
          tunnel: [w1622] -> w1561
          tunnel: w1590 -> [w1622]
          tunnel: [w1621] -> w1560
          tunnel: w1589 -> [w1621]
          tunnel: [w1619] -> w1559
          tunnel: w1561 -> [w1641]
          tunnel: [w1639] -> w1558
          tunnel: w1560 -> [w1640]
          tunnel: [w1638] -> w1556
          tunnel: w1559 -> [w1642]
          tunnel: [w1642] -> w1553
          tunnel: w1558 -> [w1708]
          tunnel: [w1708] -> w1557
          tunnel: w1556 -> [w1707]
          tunnel: [w1707] -> w1555
          tunnel: [w1703] -> w1554
          tunnel: w1553 -> [w1704]
          tunnel: [w1703] -> w1552
          tunnel: w1557 -> [w1726]
          tunnel: w1555 -> [w1727]
          tunnel: [w1727] -> w1581
          tunnel: w1586 -> [w1728]
          tunnel: [w1728] -> w1579
          tunnel: [w1726] -> w1577
          tunnel: w1554 -> [w1725]
          tunnel: [w1724] -> w1573
          tunnel: w1552 -> [w1724]
          tunnel: w1581 -> [w1738]
          tunnel: [w1738] -> w1580
          tunnel: w1579 -> [w1737]
          tunnel: [w1737] -> w1578
          tunnel: w1577 -> [w1735]
          tunnel: [w1735] -> w1576
          tunnel: [w1734] -> w1574
          tunnel: w1573 -> [w1734]
          tunnel: [w1742] -> w1588
          tunnel: [w1741] -> w1587
          tunnel: w1576 -> [w1743]
          tunnel: w1578 -> [w1749]
          tunnel: w1580 -> [w1744]
          tunnel: w1574 -> [w1740]
          tunnel: [w1740] -> w1571
          tunnel: [w1739] -> w1570
          tunnel: w1588 -> [w1791]
          tunnel: w1587 -> [w1790]
          tunnel: [w1788] -> w1569
          tunnel: w1571 -> [w1788]
          tunnel: [w1787] -> w1568
          tunnel: w1570 -> [w1787]
          tunnel: [w1786] -> w1566
          tunnel: [w1785] -> w1564
          tunnel: [w1796] -> w1572
          tunnel: w1569 -> [w1795]
          tunnel: w1568 -> [w1794]
          tunnel: [w1793] -> w1567
          tunnel: w1566 -> [w1793]
          tunnel: [w1792] -> w1565
          tunnel: w1564 -> [w1792]
          tunnel: [w1802] -> w1585
          tunnel: [w1801] -> w1584
          tunnel: w1572 -> [w1800]
          tunnel: w1567 -> [w1799]
          tunnel: w1565 -> [w1798]
          tunnel: w1585 -> [w1891]
          tunnel: w1584 -> [w1890]
          tunnel: [w1888] -> w1583
          tunnel: [w1887] -> w1582
          tunnel: w1583 -> [w1906]
          tunnel: w1582 -> [w1905]
          tunnel: [w1903] -> w1563
          tunnel: [w1902] -> w1562
          tunnel: [w1912] -> w1575
          tunnel: w1563 -> [w1913]
          tunnel: w1562 -> [w1914]
          frame #0 {
            w1596 = TRUE
            n637 = Cluster To Array(cluster=T11 {"Message"="V2", "Message 2"="V3", "Message 3"="V4"}) -> (array=w1601:string[])
            n638 = for {
              tunnel: w1601 -> [w1608] mode=indexing
              tunnel: w1600 -> [w1607]
              tunnel: w1599 -> [w1606]
              tunnel: [w1605] -> w1598
              tunnel: [w1604] -> w1597
              tunnel: w1596 -> [w1603]
              n639 = Bundle(cluster=T5 {"Message"="", "Message Data"=variant} ("Message Cluster"), "Message"=w1608, "Message Data"=w1603) -> (w1610:T5)
              n640 = Enqueue Element(queue=w1607, element=w1610, error in (no error)=w1606) -> (queue out=w1605:refnum<queue>, error out=w1604:errorcluster)  [unwired: 1 in, 1 out]
            }
            n641 = local write "High Cal\n140 Torr"(TRUE ("High Cal")) -> ()
            n642 = local write "eV2"(w1596) -> ()
            n643 = local write "eV4"(w1596) -> ()
            n644 = local write "eV3"(w1596) -> ()
          }
          frame #1 {
            n645 = local read "MFC_1 140 Torr\nUser Set Value"() -> (w1611:dbl)
            n646 = local write "MFC_1\nSLPM Value"(w1611) -> ()
            n647 = Bundle(cluster=T5 {"Message"="", "Message Data"=variant} ("Message Cluster"), "Message"="MFC_1", "Message Data"=w1611) -> (w1614:T5)
            n648 = Enqueue Element(queue=w1616, element=w1614, error in (no error)=w1615) -> (queue out=w1613:refnum<queue>, error out=w1612:errorcluster)  [unwired: 1 in, 1 out]
          }
          frame #2 {
            n649 = for {
              N: "Span High, High, Low, Target Cal\nFlush Start Time (seconds)" -> [w1632]
              tunnel: [w1624] -> w1619
              i -> [w1631]
              stop <- w1624 stop-if-true
              n650 = local read "FGGA 140 Torr\nCalibration Abort"() -> (w1625:bool)
              n651 = case shown="True" w1625 {
                selector: w1625 -> [w1635 _]
                tunnel: [w1635 w1636] -> w1623
                frame False {
                }
                frame True {
                  n652 = Two Button Dialog(message="Are you sure to abort FGGA Span Cal?") -> (T button?=w1636:bool)  [unwired: 2 in]
                }
              }
              n653 = local read "Network disconnected"() -> (w1626:bool)
              n654 = Subtract(x=w1632, y=w1631) -> (x-y=w1630:i32)
              n655 = Decrement(x=w1630) -> (x-1=w1628:i32)
              n656 = Wait (ms)(milliseconds to wait=u32 1000) -> ()  [unwired: 1 out]
              n657 = Or(x=w1626, y=w1623) -> (x .or. y?=w1624:bool)
              n658 = case shown="False" w1623 {
                selector: w1623 -> [w1634 _]
                frame False {
                  n659 = local write "FGGA 140 Torr\nCalibration Abort"(w1634) -> ()
                }
                frame True {
                }
              }
              n660 = Select(t=0, s=w1624, f=w1628) -> (s? t:f=w1627:i32)
              n661 = local write "High Cal 140 Torr\nFlush Time Remain (sec)"(w1627) -> ()
            }
          }
          frame #3 {
            n662 = case shown="False" w1642 {
              tunnel: w1641 -> [w1647 w1702]
              tunnel: w1640 -> [w1646 w1701]
              tunnel: [w1644 w1702] -> w1639
              tunnel: [w1643 w1701] -> w1638
              frame False {
                # "High to Low Flow"
                # "Carry on if connection to cRIO is made\nor calibration not abort"
                n663 = flat-sequence {
                  tunnel: [w1664] -> w1659
                  tunnel: w1647 -> [w1663]
                  tunnel: [w1662] -> w1658
                  tunnel: w1646 -> [w1660]
                  tunnel: [w1670] -> w1657
                  tunnel: w1659 -> [w1670]
                  tunnel: [w1669] -> w1656
                  tunnel: w1658 -> [w1669]
                  tunnel: w1645 -> [w1668]
                  tunnel: w1657 -> [w1672]
                  tunnel: w1656 -> [w1671]
                  tunnel: [w1677] -> w1655
                  tunnel: [w1676] -> w1654
                  tunnel: w1655 -> [w1681]
                  tunnel: w1654 -> [w1680]
                  tunnel: [w1681] -> w1653
                  tunnel: [w1680] -> w1652
                  tunnel: w1645 -> [w1679]
                  tunnel: w1653 -> [w1685]
                  tunnel: w1652 -> [w1684]
                  tunnel: [w1683] -> w1651
                  tunnel: [w1682] -> w1650
                  tunnel: [w1692] -> w1649
                  tunnel: w1651 -> [w1692]
                  tunnel: [w1691] -> w1648
                  tunnel: w1650 -> [w1691]
                  tunnel: w1645 -> [w1690]
                  tunnel: w1649 -> [w1696]
                  tunnel: w1648 -> [w1695]
                  tunnel: [w1694] -> w1644
                  tunnel: [w1693] -> w1643
                  frame #0 {
                    w1661 = FALSE
                    n664 = Bundle(cluster=T5 {"Message"="", "Message Data"=variant} ("Message Cluster"), "Message"="V10", "Message Data"=w1661) -> (w1667:T5)
                    n665 = local write "eV10"(w1661) -> ()
                    n666 = Enqueue Element(queue=w1663, element=w1667, error in (no error)=w1660) -> (queue out=w1662:refnum<queue>, error out=w1664:errorcluster)  [unwired: 1 in, 1 out]
                  }
                  frame #1 {
                    n667 = Wait (ms)(milliseconds to wait=w1668) -> ()  [unwired: 1 out]
                  }
                  frame #2 {
                    w1678 = FALSE
                    n668 = Bundle(cluster=T5 {"Message"="", "Message Data"=variant} ("Message Cluster"), "Message"="V12" ("Message 2"), "Message Data"=w1678) -> (w1675:T5)
                    n669 = local write "eV12"(w1678) -> ()
                    n670 = Enqueue Element(queue=w1671, element=w1675, error in (no error)=w1672) -> (queue out=w1677:refnum<queue>, error out=w1676:errorcluster)  [unwired: 1 in, 1 out]
                  }
                  frame #3 {
                    n671 = Wait (ms)(milliseconds to wait=w1679) -> ()  [unwired: 1 out]
                  }
                  frame #4 {
                    w1686 = TRUE
                    n672 = local write "eV11"(w1686) -> ()
                    n673 = Bundle(cluster=T5 {"Message"="", "Message Data"=variant} ("Message Cluster"), "Message"="V11" ("Message 2"), "Message Data"=w1686) -> (w1687:T5)
                    n674 = Enqueue Element(queue=w1685, element=w1687, error in (no error)=w1684) -> (queue out=w1683:refnum<queue>, error out=w1682:errorcluster)  [unwired: 1 in, 1 out]
                  }
                  frame #5 {
                    n675 = Wait (ms)(milliseconds to wait=w1690) -> ()  [unwired: 1 out]
                  }
                  frame #6 {
                    n676 = Bundle(cluster=T5 {"Message"="", "Message Data"=variant} ("Message Cluster"), "Message"="FGGA_pump", "Message Data"=TRUE) -> (w1700:T5)
                    n677 = Enqueue Element(queue=w1696, element=w1700, error in (no error)=w1695) -> (queue out=w1694:refnum<queue>, error out=w1693:errorcluster)  [unwired: 1 in, 1 out]
                  }
                }
                n678 = local read "Time delay (msec) between\nvalves switching"() -> (w1645:u32)
              }
              frame True {
              }
            }
          }
          frame #4 {
            n679 = for {
              N: "Span High, High, Low, Target  Cal\nContinue Flush Time (seconds)" -> [w1718]
              tunnel: [w1710] -> w1705
              i -> [w1717]
              stop <- w1710 stop-if-true
              n680 = local read "FGGA 140 Torr\nCalibration Abort"() -> (w1711:bool)
              n681 = case shown="True" w1711 {
                selector: w1711 -> [w1721 _]
                tunnel: [w1721 w1722] -> w1709
                frame False {
                }
                frame True {
                  n682 = Two Button Dialog(message="Are you sure to abort FGGA Span Cal?") -> (T button?=w1722:bool)  [unwired: 2 in]
                }
              }
              n683 = local read "Network disconnected"() -> (w1712:bool)
              n684 = Subtract(x=w1718, y=w1717) -> (x-y=w1716:i32)
              n685 = Decrement(x=w1716) -> (x-1=w1714:i32)
              n686 = Wait (ms)(milliseconds to wait=u32 1000) -> ()  [unwired: 1 out]
              n687 = Or(x=w1712, y=w1709) -> (x .or. y?=w1710:bool)
              n688 = case shown="False" w1709 {
                selector: w1709 -> [w1720 _]
                frame False {
                  n689 = local write "FGGA 140 Torr\nCalibration Abort"(w1720) -> ()
                }
                frame True {
                }
              }
              n690 = Select(t=0, s=w1710, f=w1714) -> (s? t:f=w1713:i32)
              n691 = local write "High Cal 140 Torr\nFlush Time Remain (sec)"(w1713) -> ()
            }
            n692 = Or(x=w1705, y=w1704) -> (x .or. y?=w1703:bool)
          }
          frame #5 {
            n693 = case shown="False" w1725 {
              tunnel: w1728 -> [w1729 _]
              frame False {
                # "CO Cal if no network\ndisconnect or abort cal"
                n694 = Bundle(cluster=T5 {"Message"="", "Message Data"=variant} ("Message Cluster"), "Message"="CO CAL", "Message Data"=TRUE) -> (w1731:T5)
                n695 = Enqueue Element(queue=w1729, element=w1731) -> ()  [unwired: 2 in, 3 out]
              }
              frame True {
              }
            }
          }
          frame #6 {
            # "To Ensure\nCO CAL\nis certain"
            n696 = Wait (ms)(milliseconds to wait=u32 1000) -> ()  [unwired: 1 out]
          }
          frame #7 {
            n697 = Bundle(cluster=T5 {"Message"="", "Message Data"=variant} ("Message Cluster"), "Message"="CO CAL", "Message Data"=FALSE) -> (w1745:T5)
            n698 = Enqueue Element(queue=w1749, element=w1745) -> ()  [unwired: 2 in, 3 out]
            n699 = case shown="False" w1740 {
              selector: w1740 -> [_ w1779]
              tunnel: w1744 -> [w1750 w1780]
              tunnel: w1743 -> [w1751 w1781]
              tunnel: [w1760 w1781] -> w1742
              tunnel: [w1759 w1780] -> w1741
              tunnel: [w1758 w1779] -> w1739
              frame False {
                w1757 = TRUE
                # "Carry on if connection to cRIO is made\nor calibration not abort"
                n700 = Bundle(cluster=T5 {"Message"="", "Message Data"=variant} ("Message Cluster"), "Message"="V1", "Message Data"=w1757) -> (w1756:T5)
                n701 = local write "eV1"(w1757) -> ()
                n702 = Enqueue Element(queue=w1751, element=w1756, error in (no error)=w1750) -> (queue out=w1752:refnum<queue>, error out=w1753:errorcluster)  [unwired: 1 in, 1 out]
                n703 = for {
                  N: "Span High, High Low, Target\nCal Time (seconds)" -> [w1773]
                  tunnel: w1752 -> [w1764]
                  tunnel: w1753 -> [w1763]
                  tunnel: [w1764] -> w1760
                  tunnel: [w1763] -> w1759
                  tunnel: [w1762] -> w1758
                  i -> [w1772]
                  stop <- w1762 stop-if-true
                  n704 = local read "FGGA 140 Torr\nCalibration Abort"() -> (w1767:bool)
                  n705 = case shown="True" w1767 {
                    selector: w1767 -> [w1776 _]
                    tunnel: [w1776 w1777] -> w1765
                    frame False {
                    }
                    frame True {
                      n706 = Two Button Dialog(message="Are you sure to abort FGGA Span Cal?") -> (T button?=w1777:bool)  [unwired: 2 in]
                    }
                  }
                  n707 = Subtract(x=w1773, y=w1772) -> (x-y=w1771:i32)
                  n708 = Decrement(x=w1771) -> (x-1=w1769:i32)
                  n709 = Wait (ms)(milliseconds to wait=u32 1000) -> ()  [unwired: 1 out]
                  n710 = local read "Network disconnected"() -> (w1766:bool)
                  n711 = Or(x=w1766, y=w1765) -> (x .or. y?=w1762:bool)
                  n712 = case shown="False" w1765 {
                    selector: w1765 -> [w1775 _]
                    frame False {
                      n713 = local write "FGGA 140 Torr\nCalibration Abort"(w1775) -> ()
                    }
                    frame True {
                    }
                  }
                  n714 = Select(t=0, s=w1762, f=w1769) -> (s? t:f=w1768:i32)
                  n715 = local write "High Cal 140 Torr\nCal Time Remain (sec)"(w1768) -> ()
                }
              }
              frame True {
              }
            }
          }
          frame #8 {
            w1789 = FALSE
            # "Note: eV2, eV4, eV1 and MFC 1 stays ON"
            n716 = local write "eV3"(w1789) -> ()
            n717 = Bundle(cluster=T5 {"Message"="", "Message Data"=variant} ("Message Cluster"), "Message"="V3" ("Message 2"), "Message Data"=w1789) -> (w1784:T5)
            n718 = Enqueue Element(queue=w1791, element=w1784, error in (no error)=w1790) -> (queue out=w1786:refnum<queue>, error out=w1785:errorcluster)  [unwired: 1 in, 1 out]
          }
          frame #9 {
            n719 = local write "High Cal\n140 Torr"(FALSE ("High Cal")) -> ()
            n720 = Or(x=w1795, y=w1794) -> (x .or. y?=w1796:bool)
          }
          frame #10 {
            n721 = case shown="False" w1800 {
              tunnel: [w1810 w1885] -> w1802
              tunnel: [w1809 w1886] -> w1801
              tunnel: w1799 -> [w1807 w1885]
              tunnel: w1798 -> [w1806 w1886]
              frame False {
                w1815 = TRUE
                n722 = local write "eV2"(w1815) -> ()
                n723 = local write "Low Cal\n140 Torr"(TRUE ("Low Cal")) -> ()
                n724 = Bundle(cluster=T5 {"Message"="", "Message Data"=variant} ("Message Cluster"), "Message"="V2", "Message Data"=w1815) -> (w1805:T5)
                n725 = Enqueue Element(queue=w1807, element=w1805, error in (no error)=w1806) -> (queue out=w1817:refnum<queue>, error out=w1819:errorcluster)  [unwired: 1 in, 1 out]
                n726 = local read "MFC_1 140 Torr\nUser Set Value"() -> (w1820:dbl)
                n727 = local write "MFC_1\nSLPM Value"(w1820) -> ()
                n728 = Bundle(cluster=T5 {"Message"="", "Message Data"=variant} ("Message Cluster"), "Message"="MFC_1", "Message Data"=w1820) -> (w1821:T5)
                n729 = Enqueue Element(queue=w1817, element=w1821, error in (no error)=w1819) -> (queue out=w1814:refnum<queue>, error out=w1812:errorcluster)  [unwired: 1 in, 1 out]
                n730 = disable-structure shown="Enabled" {
                  disable-tunnel: w1814 -> [w1827 w1846]
                  disable-tunnel: [w1826 w1846] -> w1813
                  disable-tunnel: w1812 -> [w1825 w1847]
                  disable-tunnel: [w1824 w1847] -> w1811
                  disable-tunnel: [w1823 FALSE] -> w1808
                  frame Disabled {
                    n731 = for {
                      N: "Span Low Flush Time (seconds)" -> [w1840]
                      tunnel: [w1831] -> w1826
                      tunnel: w1827 -> [w1831]
                      tunnel: [w1830] -> w1824
                      tunnel: w1825 -> [w1830]
                      tunnel: [w1829] -> w1823
                      i -> [w1839]
                      stop <- w1829 stop-if-true
                      n732 = local read "FGGA 140 Torr\nCalibration Abort"() -> (w1834:bool)
                      n733 = case shown="True" w1834 {
                        selector: w1834 -> [w1843 _]
                        tunnel: [w1843 w1844] -> w1832
                        frame False {
                        }
                        frame True {
                          n734 = Two Button Dialog(message="Are you sure to abort FGGA Span Cal?") -> (T button?=w1844:bool)  [unwired: 2 in]
                        }
                      }
                      n735 = Subtract(x=w1840, y=w1839) -> (x-y=w1838:i32)
                      n736 = Decrement(x=w1838) -> (x-1=w1835:i32)
                      n737 = Wait (ms)(milliseconds to wait=u32 1000) -> ()  [unwired: 1 out]
                      n738 = local read "Network disconnected"() -> (w1833:bool)
                      n739 = case shown="False" w1832 {
                        selector: w1832 -> [w1842 _]
                        frame False {
                          n740 = local write "FGGA 140 Torr\nCalibration Abort"(w1842) -> ()
                        }
                        frame True {
                        }
                      }
                      n741 = Or(x=w1833, y=w1832) -> (x .or. y?=w1829:bool)
                      n742 = Select(t=0, s=w1829, f=w1835) -> (s? t:f=w1836:i32)
                      n743 = local write "Low Cal 140 Torr\nFlush Time Remain (sec)"(w1836) -> ()
                    }
                  }
                  frame Enabled {
                  }
                }
                n744 = case shown="False" w1808 {
                  tunnel: w1813 -> [w1854 w1884]
                  tunnel: w1811 -> [w1853 w1883]
                  tunnel: [w1851 w1884] -> w1810
                  tunnel: [w1849 w1883] -> w1809
                  frame False {
                    n745 = disable-structure shown="Enabled" {
                      disable-tunnel: w1854 -> [w1859 w1865]
                      disable-tunnel: w1853 -> [w1858 w1864]
                      disable-tunnel: [w1857 w1865] -> w1852
                      disable-tunnel: [w1856 w1864] -> w1850
                      frame Disabled {
                        w1860 = TRUE
                        n746 = local write "eV1"(w1860) -> ()
                        n747 = Bundle(cluster=T5 {"Message"="", "Message Data"=variant} ("Message Cluster"), "Message"="V1", "Message Data"=w1860) -> (w1862:T5)
                        n748 = Enqueue Element(queue=w1859, element=w1862, error in (no error)=w1858) -> (queue out=w1857:refnum<queue>, error out=w1856:errorcluster)  [unwired: 1 in, 1 out]
                      }
                      frame Enabled {
                      }
                    }
                    n749 = for {
                      N: "Span Low Cal Time (seconds)" -> [w1877]
                      tunnel: [w1867] -> w1851
                      tunnel: w1852 -> [w1867]
                      tunnel: w1850 -> [w1866]
                      tunnel: [w1866] -> w1849
                      i -> [w1876]
                      stop <- w1868 stop-if-true
                      n750 = local read "FGGA 140 Torr\nCalibration Abort"() -> (w1871:bool)
                      n751 = case shown="True" w1871 {
                        selector: w1871 -> [w1880 _]
                        tunnel: [w1880 w1881] -> w1869
                        frame False {
                        }
                        frame True {
                          n752 = Two Button Dialog(message="Are you sure to abort FGGA Span Cal?") -> (T button?=w1881:bool)  [unwired: 2 in]
                        }
                      }
                      n753 = Wait (ms)(milliseconds to wait=u32 1000) -> ()  [unwired: 1 out]
                      n754 = local read "Network disconnected"() -> (w1870:bool)
                      n755 = Subtract(x=w1877, y=w1876) -> (x-y=w1875:i32)
                      n756 = Decrement(x=w1875) -> (x-1=w1872:i32)
                      n757 = Or(x=w1870, y=w1869) -> (x .or. y?=w1868:bool)
                      n758 = case shown="False" w1869 {
                        selector: w1869 -> [w1879 _]
                        frame False {
                          n759 = local write "FGGA 140 Torr\nCalibration Abort"(w1879) -> ()
                        }
                        frame True {
                        }
                      }
                      n760 = Select(t=0, s=w1868, f=w1872) -> (s? t:f=w1873:i32)
                      n761 = local write "Low Cal 140 Torr\nCal Time Remain (sec)"(w1873) -> ()
                    }
                  }
                  frame True {
                    # "Ignore Cal if connection problem or abort button pressed"
                  }
                }
              }
              frame True {
                # "Ignore Cal if connection problem or abort button pressed"
              }
            }
          }
          frame #11 {
            w1889 = FALSE
            n762 = Cluster To Array(cluster=T14 {"Message"="V2", "Message 3"="V4", "Message 4"="V1"}) -> (array=w1892:string[])
            n763 = local write "eV1"(w1889) -> ()
            n764 = local write "eV2"(w1889) -> ()
            n765 = local write "eV4"(w1889) -> ()
            n766 = for {
              tunnel: w1892 -> [w1899] mode=indexing
              tunnel: [w1898] -> w1888
              tunnel: [w1897] -> w1887
              tunnel: w1889 -> [w1896]
              tunnel: w1891 -> [w1895]
              tunnel: w1890 -> [w1894]
              n767 = Bundle(cluster=T5 {"Message"="", "Message Data"=variant} ("Message Cluster"), "Message"=w1899, "Message Data"=w1896) -> (w1901:T5)
              n768 = Enqueue Element(queue=w1895, element=w1901, error in (no error)=w1894) -> (queue out=w1898:refnum<queue>, error out=w1897:errorcluster)  [unwired: 1 in, 1 out]
            }
          }
          frame #12 {
            w1904 = 0.0 ("MFC_1\nSLPM Value")
            n769 = local write "MFC_1\nSLPM Value"(w1904) -> ()
            n770 = Bundle(cluster=T5 {"Message"="", "Message Data"=variant} ("Message Cluster"), "Message"="MFC_1", "Message Data"=w1904) -> (w1908:T5)
            n771 = Enqueue Element(queue=w1906, element=w1908, error in (no error)=w1905) -> (queue out=w1902:refnum<queue>, error out=w1903:errorcluster)  [unwired: 1 in, 1 out]
          }
          frame #13 {
            w1911 = FALSE
            # "Set back to high flow only if High Flow master switch is ON"
            n772 = local read "Time delay (msec) between\nvalves switching"() -> (w1910:u32)
            n773 = local read "HIGH FLOW MASTER SWITCH"() -> (w1915:bool)
            n774 = case shown="True" w1915 {
              tunnel: w1914 -> [_ w1926]
              tunnel: w1913 -> [w1916 w1918]
              tunnel: [w1916 w1925] -> w1912
              tunnel: w1910 -> [_ w1917]
              frame False {
              }
              frame True {
                n775 = flat-sequence {
                  tunnel: [w1936] -> w1928
                  tunnel: w1926 -> [w1935]
                  tunnel: [w1934] -> w1920
                  tunnel: w1918 -> [w1933]
                  tunnel: w1928 -> [w1943]
                  tunnel: [w1943] -> w1927
                  tunnel: w1920 -> [w1942]
                  tunnel: [w1942] -> w1919
                  tunnel: w1917 -> [w1941]
                  tunnel: [w1947] -> w1930
                  tunnel: w1927 -> [w1946]
                  tunnel: [w1945] -> w1922
                  tunnel: w1919 -> [w1944]
                  tunnel: w1930 -> [w1954]
                  tunnel: [w1954] -> w1929
                  tunnel: w1922 -> [w1953]
                  tunnel: [w1953] -> w1921
                  tunnel: w1917 -> [w1952]
                  tunnel: [w1958] -> w1932
                  tunnel: w1929 -> [w1957]
                  tunnel: [w1956] -> w1924
                  tunnel: w1921 -> [w1955]
                  tunnel: w1932 -> [w1965]
                  tunnel: [w1965] -> w1931
                  tunnel: w1924 -> [w1964]
                  tunnel: [w1964] -> w1923
                  tunnel: w1917 -> [w1963]
                  tunnel: w1931 -> [w1969]
                  tunnel: [w1967] -> w1925
                  tunnel: w1923 -> [w1966]
                  frame #0 {
                    n776 = Bundle(cluster=T5 {"Message"="", "Message Data"=variant} ("Message Cluster"), "Message"="FGGA_pump", "Message Data"=FALSE) -> (w1937:T5)
                    n777 = Enqueue Element(queue=w1935, element=w1937, error in (no error)=w1933) -> (queue out=w1936:refnum<queue>, error out=w1934:errorcluster)  [unwired: 1 in, 1 out]
                  }
                  frame #1 {
                    n778 = Wait (ms)(milliseconds to wait=w1941) -> ()  [unwired: 1 out]
                  }
                  frame #2 {
                    w1948 = FALSE
                    n779 = Bundle(cluster=T5 {"Message"="", "Message Data"=variant} ("Message Cluster"), "Message"="V11" ("Message 2"), "Message Data"=w1948) -> (w1949:T5)
                    n780 = Enqueue Element(queue=w1946, element=w1949, error in (no error)=w1944) -> (queue out=w1947:refnum<queue>, error out=w1945:errorcluster)  [unwired: 1 in, 1 out]
                    n781 = local write "eV11"(w1948) -> ()
                  }
                  frame #3 {
                    n782 = Wait (ms)(milliseconds to wait=w1952) -> ()  [unwired: 1 out]
                  }
                  frame #4 {
                    w1959 = TRUE
                    n783 = local write "eV12"(w1959) -> ()
                    n784 = Bundle(cluster=T5 {"Message"="", "Message Data"=variant} ("Message Cluster"), "Message"="V12" ("Message 2"), "Message Data"=w1959) -> (w1961:T5)
                    n785 = Enqueue Element(queue=w1957, element=w1961, error in (no error)=w1955) -> (queue out=w1958:refnum<queue>, error out=w1956:errorcluster)  [unwired: 1 in, 1 out]
                  }
                  frame #5 {
                    n786 = Wait (ms)(milliseconds to wait=w1963) -> ()  [unwired: 1 out]
                  }
                  frame #6 {
                    w1970 = TRUE
                    n787 = Bundle(cluster=T5 {"Message"="", "Message Data"=variant} ("Message Cluster"), "Message"="V10", "Message Data"=w1970) -> (w1971:T5)
                    n788 = local write "eV10"(w1970) -> ()
                    n789 = Enqueue Element(queue=w1969, element=w1971, error in (no error)=w1966) -> (error out=w1967:errorcluster)  [unwired: 1 in, 2 out]
                  }
                }
              }
            }
            n790 = local write "Span Cal 140 Torr - \nHigh Cal, CO Cal, Low Cal"(w1911) -> ()
            n791 = local write "FGGA 140 Torr\nCalibration Abort"(w1911) -> ()
            n792 = local write "Low Cal\n140 Torr"(w1911) -> ()
          }
        }
      }
      event "Flush High Tank": Value Change {
        n793 = event-data() -> ()  [unwired: 1 in, 6 out]
        n794 = flat-sequence {
          tunnel: w1984 -> [w1989]
          tunnel: w1983 -> [w1988]
          tunnel: [w1987] -> w1982
          tunnel: [w1986] -> w1981
          tunnel: w1982 -> [w2005]
          tunnel: w1981 -> [w2004]
          tunnel: [w2002] -> w1980
          tunnel: [w2001] -> w1979
          tunnel: w1980 -> [w2008]
          tunnel: w1979 -> [w2009]
          tunnel: [w2009] -> w1974
          tunnel: [w2008] -> w1973
          tunnel: [w2022] -> w1978
          tunnel: [w2021] -> w1977
          tunnel: w1974 -> [w2020]
          tunnel: w1973 -> [w2019]
          tunnel: w1978 -> [w2037]
          tunnel: w1977 -> [w2036]
          tunnel: [w2034] -> w1975
          tunnel: [w2042] -> w1976
          tunnel: w1975 -> [w2042]
          frame #0 {
            w1985 = TRUE
            n795 = Cluster To Array(cluster=T11 {"Message"="V2", "Message 2"="V3", "Message 3"="V4"}) -> (array=w1990:string[])
            n796 = for {
              tunnel: w1990 -> [w1997] mode=indexing
              tunnel: w1989 -> [w1996]
              tunnel: w1988 -> [w1995]
              tunnel: [w1994] -> w1987
              tunnel: [w1993] -> w1986
              tunnel: w1985 -> [w1992]
              n797 = Bundle(cluster=T5 {"Message"="", "Message Data"=variant} ("Message Cluster"), "Message"=w1997, "Message Data"=w1992) -> (w1999:T5)
              n798 = Enqueue Element(queue=w1996, element=w1999, error in (no error)=w1995) -> (queue out=w1994:refnum<queue>, error out=w1993:errorcluster)  [unwired: 1 in, 1 out]
            }
            n799 = local write "eV2"(w1985) -> ()
            n800 = local write "eV4"(w1985) -> ()
            n801 = local write "eV3"(w1985) -> ()
          }
          frame #1 {
            n802 = local read "MFC_1 User Set Value"() -> (w2000:dbl)
            n803 = local write "MFC_1\nSLPM Value"(w2000) -> ()
            n804 = Bundle(cluster=T5 {"Message"="", "Message Data"=variant} ("Message Cluster"), "Message"="MFC_1", "Message Data"=w2000) -> (w2003:T5)
            n805 = Enqueue Element(queue=w2005, element=w2003, error in (no error)=w2004) -> (queue out=w2002:refnum<queue>, error out=w2001:errorcluster)  [unwired: 1 in, 1 out]
          }
          frame #2 {
            n806 = for {
              N: 15 -> [w2017]
              i -> [w2016]
              stop <- w2012 stop-if-true
              n807 = Subtract(x=w2017, y=w2016) -> (x-y=w2015:i32)
              n808 = Decrement(x=w2015) -> (x-1=w2013:i32)
              n809 = local read "Network disconnected"() -> (w2012:bool)
              n810 = Wait (ms)(milliseconds to wait=u32 1000) -> ()  [unwired: 1 out]
              n811 = Select(t=0, s=w2012, f=w2013) -> (s? t:f=→"Flush High Tank\nTime Remain (sec)":i32)
            }
          }
          frame #3 {
            w2023 = FALSE
            n812 = Cluster To Array(cluster=T11 {"Message"="V2", "Message 2"="V3", "Message 3"="V4"}) -> (array=w2024:string[])
            n813 = for {
              tunnel: w2024 -> [w2031] mode=indexing
              tunnel: [w2030] -> w2022
              tunnel: [w2029] -> w2021
              tunnel: w2023 -> [w2028]
              tunnel: w2019 -> [w2027]
              tunnel: w2020 -> [w2026]
              n814 = Bundle(cluster=T5 {"Message"="", "Message Data"=variant} ("Message Cluster"), "Message"=w2031, "Message Data"=w2028) -> (w2033:T5)
              n815 = Enqueue Element(queue=w2027, element=w2033, error in (no error)=w2026) -> (queue out=w2030:refnum<queue>, error out=w2029:errorcluster)  [unwired: 1 in, 1 out]
            }
            n816 = local write "eV2"(w2023) -> ()
            n817 = local write "eV4"(w2023) -> ()
            n818 = local write "eV3"(w2023) -> ()
          }
          frame #4 {
            w2035 = 0.0 ("MFC_1\nSLPM Value")
            n819 = local write "MFC_1\nSLPM Value"(w2035) -> ()
            n820 = Bundle(cluster=T5 {"Message"="", "Message Data"=variant} ("Message Cluster"), "Message"="MFC_1", "Message Data"=w2035) -> (w2039:T5)
            n821 = Enqueue Element(queue=w2037, element=w2039, error in (no error)=w2036) -> (error out=w2034:errorcluster)  [unwired: 1 in, 2 out]
          }
          frame #5 {
            n822 = local write "Flush High Tank"(FALSE ("High Cal")) -> ()
          }
        }
      }
      event "LOW FLOW MASTER SWITCH": Value Change {
        # "High Flow to Low Flow"
        n823 = event-data() -> ()  [unwired: 1 in, 6 out]
        n824 = flat-sequence {
          tunnel: w2058 -> [w2060]
          tunnel: w2059 -> [w2063]
          tunnel: [w2062] -> w2057
          tunnel: [w2061] -> w2056
          tunnel: w2057 -> [w2075]
          tunnel: w2056 -> [w2074]
          tunnel: [w2072] -> w2046
          tunnel: [w2073] -> w2044
          tunnel: w2046 -> [w2079]
          tunnel: [w2079] -> w2045
          tunnel: w2044 -> [w2078]
          tunnel: [w2078] -> w2043
          tunnel: w2045 -> [w2082]
          tunnel: [w2081] -> w2048
          tunnel: w2043 -> [w2084]
          tunnel: [w2083] -> w2047
          tunnel: w2048 -> [w2090]
          tunnel: [w2090] -> w2054
          tunnel: w2047 -> [w2089]
          tunnel: [w2089] -> w2053
          tunnel: w2054 -> [w2095]
          tunnel: [w2094] -> w2052
          tunnel: w2053 -> [w2093]
          tunnel: [w2092] -> w2050
          tunnel: w2052 -> [w2101]
          tunnel: [w2101] -> w2051
          tunnel: w2050 -> [w2100]
          tunnel: [w2100] -> w2049
          tunnel: [w2102] -> w2055
          tunnel: w2051 -> [w2104]
          tunnel: w2049 -> [w2103]
          frame #0 {
            n825 = local write "HIGH FLOW MASTER SWITCH"(FALSE ("HIGH FLOW MASTER SWITCH")) -> ()
            n826 = Bundle(cluster=T5 {"Message"="", "Message Data"=variant} ("Message Cluster"), "Message"="Low_Flow", "Message Data"=TRUE) -> (w2066:T5)
            n827 = Enqueue Element(queue=w2063, element=w2066, error in (no error)=w2060) -> (queue out=w2062:refnum<queue>, error out=w2061:errorcluster)  [unwired: 1 in, 1 out]
          }
          frame #1 {
            w2076 = FALSE
            n828 = local write "eV10"(w2076) -> ()
            n829 = Bundle(cluster=T5 {"Message"="", "Message Data"=variant} ("Message Cluster"), "Message"="V10", "Message Data"=w2076) -> (w2071:T5)
            n830 = Enqueue Element(queue=w2075, element=w2071, error in (no error)=w2074) -> (queue out=w2073:refnum<queue>, error out=w2072:errorcluster)  [unwired: 1 in, 1 out]
          }
          frame #2 {
            n831 = local read "Time delay (msec) between\nvalves switching"() -> (w2077:u32)
            n832 = Wait (ms)(milliseconds to wait=w2077) -> ()  [unwired: 1 out]
          }
          frame #3 {
            w2080 = FALSE
            n833 = Bundle(cluster=T5 {"Message"="", "Message Data"=variant} ("Message Cluster"), "Message"="V12" ("Message 2"), "Message Data"=w2080) -> (w2087:T5)
            n834 = local write "eV12"(w2080) -> ()
            n835 = Enqueue Element(queue=w2084, element=w2087, error in (no error)=w2082) -> (queue out=w2083:refnum<queue>, error out=w2081:errorcluster)  [unwired: 1 in, 1 out]
          }
          frame #4 {
            n836 = local read "Time delay (msec) between\nvalves switching"() -> (w2088:u32)
            n837 = Wait (ms)(milliseconds to wait=w2088) -> ()  [unwired: 1 out]
          }
          frame #5 {
            w2091 = TRUE
            n838 = local write "eV11"(w2091) -> ()
            n839 = Bundle(cluster=T5 {"Message"="", "Message Data"=variant} ("Message Cluster"), "Message"="V11" ("Message 2"), "Message Data"=w2091) -> (w2098:T5)
            n840 = Enqueue Element(queue=w2093, element=w2098, error in (no error)=w2095) -> (queue out=w2092:refnum<queue>, error out=w2094:errorcluster)  [unwired: 1 in, 1 out]
          }
          frame #6 {
            n841 = local read "Time delay (msec) between\nvalves switching"() -> (w2099:u32)
            n842 = Wait (ms)(milliseconds to wait=w2099) -> ()  [unwired: 1 out]
          }
          frame #7 {
            n843 = Bundle(cluster=T5 {"Message"="", "Message Data"=variant} ("Message Cluster"), "Message"="FGGA_pump", "Message Data"=TRUE) -> (w2108:T5)
            n844 = Enqueue Element(queue=w2103, element=w2108, error in (no error)=w2104) -> (error out=w2102:errorcluster)  [unwired: 1 in, 2 out]
          }
        }
      }
      event "HIGH FLOW MASTER SWITCH": Value Change {
        # "Low Flow to High Flow"
        n845 = event-data() -> ()  [unwired: 1 in, 6 out]
        n846 = flat-sequence {
          tunnel: w2124 -> [w2128]
          tunnel: w2125 -> [w2129]
          tunnel: [w2127] -> w2122
          tunnel: [w2126] -> w2121
          tunnel: w2122 -> [w2138]
          tunnel: w2121 -> [w2137]
          tunnel: [w2136] -> w2120
          tunnel: [w2135] -> w2118
          tunnel: w2120 -> [w2145]
          tunnel: [w2145] -> w2119
          tunnel: w2118 -> [w2144]
          tunnel: [w2144] -> w2117
          tunnel: w2119 -> [w2150]
          tunnel: w2117 -> [w2149]
          tunnel: [w2147] -> w2116
          tunnel: [w2146] -> w2114
          tunnel: w2116 -> [w2156]
          tunnel: [w2156] -> w2115
          tunnel: w2114 -> [w2155]
          tunnel: [w2155] -> w2113
          tunnel: w2115 -> [w2164]
          tunnel: w2113 -> [w2163]
          tunnel: [w2159] -> w2112
          tunnel: [w2158] -> w2110
          tunnel: w2112 -> [w2167]
          tunnel: [w2167] -> w2111
          tunnel: w2110 -> [w2166]
          tunnel: [w2166] -> w2109
          tunnel: [w2169] -> w2123
          tunnel: w2111 -> [w2171]
          tunnel: w2109 -> [w2170]
          frame #0 {
            n847 = local write "LOW FLOW MASTER SWITCH"(FALSE ("LOW FLOW MASTER SWITCH")) -> ()
            n848 = Bundle(cluster=T5 {"Message"="", "Message Data"=variant} ("Message Cluster"), "Message"="High_Flow", "Message Data"=TRUE) -> (w2133:T5)
            n849 = Enqueue Element(queue=w2129, element=w2133, error in (no error)=w2128) -> (queue out=w2127:refnum<queue>, error out=w2126:errorcluster)  [unwired: 1 in, 1 out]
          }
          frame #1 {
            n850 = Bundle(cluster=T5 {"Message"="", "Message Data"=variant} ("Message Cluster"), "Message"="FGGA_pump", "Message Data"=FALSE) -> (w2142:T5)
            n851 = Enqueue Element(queue=w2138, element=w2142, error in (no error)=w2137) -> (queue out=w2136:refnum<queue>, error out=w2135:errorcluster)  [unwired: 1 in, 1 out]
          }
          frame #2 {
            n852 = local read "Time delay (msec) between\nvalves switching"() -> (w2143:u32)
            n853 = Wait (ms)(milliseconds to wait=w2143) -> ()  [unwired: 1 out]
          }
          frame #3 {
            w2148 = FALSE
            n854 = local write "eV11"(w2148) -> ()
            n855 = Bundle(cluster=T5 {"Message"="", "Message Data"=variant} ("Message Cluster"), "Message"="V11" ("Message 2"), "Message Data"=w2148) -> (w2151:T5)
            n856 = Enqueue Element(queue=w2150, element=w2151, error in (no error)=w2149) -> (queue out=w2147:refnum<queue>, error out=w2146:errorcluster)  [unwired: 1 in, 1 out]
          }
          frame #4 {
            n857 = local read "Time delay (msec) between\nvalves switching"() -> (w2154:u32)
            n858 = Wait (ms)(milliseconds to wait=w2154) -> ()  [unwired: 1 out]
          }
          frame #5 {
            w2157 = TRUE
            n859 = local write "eV12"(w2157) -> ()
            n860 = Bundle(cluster=T5 {"Message"="", "Message Data"=variant} ("Message Cluster"), "Message"="V12", "Message Data"=w2157) -> (w2162:T5)
            n861 = Enqueue Element(queue=w2164, element=w2162, error in (no error)=w2163) -> (queue out=w2158:refnum<queue>, error out=w2159:errorcluster)  [unwired: 1 in, 1 out]
          }
          frame #6 {
            n862 = local read "Time delay (msec) between\nvalves switching"() -> (w2165:u32)
            n863 = Wait (ms)(milliseconds to wait=w2165) -> ()  [unwired: 1 out]
          }
          frame #7 {
            w2168 = TRUE
            n864 = local write "eV10"(w2168) -> ()
            n865 = Bundle(cluster=T5 {"Message"="", "Message Data"=variant} ("Message Cluster"), "Message"="V10" ("Message 2"), "Message Data"=w2168) -> (w2174:T5)
            n866 = Enqueue Element(queue=w2170, element=w2174, error in (no error)=w2171) -> (error out=w2169:errorcluster)  [unwired: 1 in, 2 out]
          }
        }
      }
      event "FLOW ALL OFF": Value Change {
        n867 = event-data() -> ()  [unwired: 1 in, 6 out]
        n868 = Two Button Dialog(message="FGGA pump, eV11, eV10 and eV12 will be OFF\nARE YOU SURE?") -> (T button?=w2175:bool)  [unwired: 2 in]
        n869 = case shown="True" w2175 {
          tunnel: w2179 -> [_ w2185]
          tunnel: w2178 -> [w2180 w2184]
          tunnel: [w2180 w2183] -> w2177
          frame False {
          }
          frame True {
            # "ALL OFF"
            n870 = flat-sequence {
              tunnel: w2184 -> [w2193]
              tunnel: w2185 -> [w2194]
              tunnel: [w2191] -> w2182
              tunnel: [w2192] -> w2181
              tunnel: [w2200] -> w2190
              tunnel: [w2199] -> w2189
              tunnel: w2182 -> [w2203]
              tunnel: w2181 -> [w2202]
              tunnel: w2190 -> [w2214]
              tunnel: w2189 -> [w2213]
              tunnel: [w2208] -> w2188
              tunnel: [w2207] -> w2187
              tunnel: w2188 -> [w2216]
              tunnel: w2187 -> [w2215]
              tunnel: [w2217] -> w2186
              tunnel: [w2230] -> w2183
              tunnel: w2186 -> [w2230]
              frame #0 {
                n871 = Bundle(cluster=T5 {"Message"="", "Message Data"=variant} ("Message Cluster"), "Message"="No_Flow", "Message Data"=TRUE) -> (w2195:T5)
                n872 = Enqueue Element(queue=w2194, element=w2195, error in (no error)=w2193) -> (queue out=w2191:refnum<queue>, error out=w2192:errorcluster)  [unwired: 1 in, 1 out]
              }
              frame #1 {
                n873 = Bundle(cluster=T5 {"Message"="", "Message Data"=variant} ("Message Cluster"), "Message"="FGGA_pump", "Message Data"=FALSE) -> (w2201:T5)
                n874 = Enqueue Element(queue=w2203, element=w2201, error in (no error)=w2202) -> (queue out=w2200:refnum<queue>, error out=w2199:errorcluster)  [unwired: 1 in, 1 out]
              }
              frame #2 {
                w2212 = FALSE
                n875 = local write "eV11"(w2212) -> ()
                n876 = Bundle(cluster=T5 {"Message"="", "Message Data"=variant} ("Message Cluster"), "Message"="V11" ("Message 2"), "Message Data"=w2212) -> (w2211:T5)
                n877 = Enqueue Element(queue=w2214, element=w2211, error in (no error)=w2213) -> (queue out=w2208:refnum<queue>, error out=w2207:errorcluster)  [unwired: 1 in, 1 out]
              }
              frame #3 {
                w2218 = FALSE
                n878 = Cluster To Array(cluster=cluster{"Message":string, "Message 2":string} {"Message"="V10", "Message 2"="V12"}) -> (array=w2219:string[])
                n879 = for {
                  tunnel: w2219 -> [w2226] mode=indexing
                  tunnel: [w2225] -> _
                  tunnel: [w2224] -> w2217
                  tunnel: w2218 -> [w2223]
                  tunnel: w2216 -> [w2222]
                  tunnel: w2215 -> [w2221]
                  n880 = Bundle(cluster=T5 {"Message"="", "Message Data"=variant} ("Message Cluster"), "Message"=w2226, "Message Data"=w2223) -> (w2228:T5)
                  n881 = Enqueue Element(queue=w2222, element=w2228, error in (no error)=w2221) -> (queue out=w2225:refnum<queue>, error out=w2224:errorcluster)  [unwired: 1 in, 1 out]
                }
                n882 = local write "eV12"(w2218) -> ()
                n883 = local write "eV10"(w2218) -> ()
              }
              frame #4 {
                w2229 = FALSE ("LOW FLOW MASTER SWITCH")
                n884 = local write "LOW FLOW MASTER SWITCH"(w2229) -> ()
                n885 = local write "HIGH FLOW MASTER SWITCH"(w2229) -> ()
                n886 = local write "FLOW ALL OFF"(w2229) -> ()
              }
            }
          }
        }
      }
      event "Flush Low Tank": Value Change {
        n887 = event-data() -> ()  [unwired: 1 in, 1 out]
        n888 = flat-sequence {
          tunnel: w2242 -> [w2247]
          tunnel: w2241 -> [w2246]
          tunnel: [w2245] -> w2240
          tunnel: [w2244] -> w2239
          tunnel: w2240 -> [w2263]
          tunnel: w2239 -> [w2262]
          tunnel: [w2260] -> w2238
          tunnel: [w2259] -> w2237
          tunnel: w2238 -> [w2266]
          tunnel: w2237 -> [w2267]
          tunnel: [w2267] -> w2232
          tunnel: [w2266] -> w2231
          tunnel: [w2280] -> w2236
          tunnel: [w2279] -> w2235
          tunnel: w2232 -> [w2278]
          tunnel: w2231 -> [w2277]
          tunnel: w2236 -> [w2295]
          tunnel: w2235 -> [w2294]
          tunnel: [w2292] -> w2233
          tunnel: [w2300] -> w2234
          tunnel: w2233 -> [w2300]
          frame #0 {
            w2243 = TRUE
            n889 = Cluster To Array(cluster=cluster{"Message":string, "Message 3":string} {"Message"="V2", "Message 3"="V4"}) -> (array=w2248:string[])
            n890 = for {
              tunnel: w2248 -> [w2255] mode=indexing
              tunnel: w2247 -> [w2254]
              tunnel: w2246 -> [w2253]
              tunnel: [w2252] -> w2245
              tunnel: [w2251] -> w2244
              tunnel: w2243 -> [w2250]
              n891 = Bundle(cluster=T5 {"Message"="", "Message Data"=variant} ("Message Cluster"), "Message"=w2255, "Message Data"=w2250) -> (w2257:T5)
              n892 = Enqueue Element(queue=w2254, element=w2257, error in (no error)=w2253) -> (queue out=w2252:refnum<queue>, error out=w2251:errorcluster)  [unwired: 1 in, 1 out]
            }
            n893 = local write "eV2"(w2243) -> ()
            n894 = local write "eV4"(w2243) -> ()
          }
          frame #1 {
            n895 = local read "MFC_1 User Set Value"() -> (w2258:dbl)
            n896 = local write "MFC_1\nSLPM Value"(w2258) -> ()
            n897 = Bundle(cluster=T5 {"Message"="", "Message Data"=variant} ("Message Cluster"), "Message"="MFC_1", "Message Data"=w2258) -> (w2261:T5)
            n898 = Enqueue Element(queue=w2263, element=w2261, error in (no error)=w2262) -> (queue out=w2260:refnum<queue>, error out=w2259:errorcluster)  [unwired: 1 in, 1 out]
          }
          frame #2 {
            n899 = for {
              N: 15 -> [w2275]
              i -> [w2274]
              stop <- w2269 stop-if-true
              n900 = Subtract(x=w2275, y=w2274) -> (x-y=w2273:i32)
              n901 = Decrement(x=w2273) -> (x-1=w2270:i32)
              n902 = local read "Network disconnected"() -> (w2269:bool)
              n903 = Wait (ms)(milliseconds to wait=u32 1000) -> ()  [unwired: 1 out]
              n904 = Select(t=0, s=w2269, f=w2270) -> (s? t:f=→"Flush Low Tank\nTime Remain (sec)":i32)
            }
          }
          frame #3 {
            w2281 = FALSE
            n905 = Cluster To Array(cluster=cluster{"Message":string, "Message 3":string} {"Message"="V2", "Message 3"="V4"}) -> (array=w2282:string[])
            n906 = for {
              tunnel: w2282 -> [w2289] mode=indexing
              tunnel: [w2288] -> w2280
              tunnel: [w2287] -> w2279
              tunnel: w2281 -> [w2286]
              tunnel: w2277 -> [w2285]
              tunnel: w2278 -> [w2284]
              n907 = Bundle(cluster=T5 {"Message"="", "Message Data"=variant} ("Message Cluster"), "Message"=w2289, "Message Data"=w2286) -> (w2291:T5)
              n908 = Enqueue Element(queue=w2285, element=w2291, error in (no error)=w2284) -> (queue out=w2288:refnum<queue>, error out=w2287:errorcluster)  [unwired: 1 in, 1 out]
            }
            n909 = local write "eV2"(w2281) -> ()
            n910 = local write "eV4"(w2281) -> ()
          }
          frame #4 {
            w2293 = 0.0 ("MFC_1\nSLPM Value")
            n911 = local write "MFC_1\nSLPM Value"(w2293) -> ()
            n912 = Bundle(cluster=T5 {"Message"="", "Message Data"=variant} ("Message Cluster"), "Message"="MFC_1", "Message Data"=w2293) -> (w2297:T5)
            n913 = Enqueue Element(queue=w2295, element=w2297, error in (no error)=w2294) -> (error out=w2292:errorcluster)  [unwired: 1 in, 2 out]
          }
          frame #5 {
            n914 = local write "Flush Low Tank"(FALSE ("High Cal")) -> ()
          }
        }
      }
      event "Flush Target Tank": Value Change {
        n915 = event-data() -> ()  [unwired: 1 in, 1 out]
        n916 = flat-sequence {
          tunnel: w2312 -> [w2320]
          tunnel: w2311 -> [w2319]
          tunnel: [w2318] -> w2310
          tunnel: [w2317] -> w2309
          tunnel: w2310 -> [w2326]
          tunnel: w2309 -> [w2325]
          tunnel: [w2323] -> w2308
          tunnel: [w2322] -> w2307
          tunnel: w2308 -> [w2329]
          tunnel: w2307 -> [w2330]
          tunnel: [w2330] -> w2302
          tunnel: [w2329] -> w2301
          tunnel: [w2346] -> w2306
          tunnel: [w2345] -> w2305
          tunnel: w2302 -> [w2344]
          tunnel: w2301 -> [w2343]
          tunnel: w2306 -> [w2351]
          tunnel: w2305 -> [w2350]
          tunnel: [w2348] -> w2303
          tunnel: [w2356] -> w2304
          tunnel: w2303 -> [w2356]
          frame #0 {
            w2316 = TRUE
            n917 = local write "eV4"(w2316) -> ()
            n918 = Bundle(cluster=T5 {"Message"="", "Message Data"=variant} ("Message Cluster"), "Message"="V4" ("Message 3"), "Message Data"=w2316) -> (w2315:T5)
            n919 = Enqueue Element(queue=w2320, element=w2315, error in (no error)=w2319) -> (queue out=w2318:refnum<queue>, error out=w2317:errorcluster)  [unwired: 1 in, 1 out]
          }
          frame #1 {
            n920 = local read "MFC_1 User Set Value"() -> (w2321:dbl)
            n921 = local write "MFC_1\nSLPM Value"(w2321) -> ()
            n922 = Bundle(cluster=T5 {"Message"="", "Message Data"=variant} ("Message Cluster"), "Message"="MFC_1", "Message Data"=w2321) -> (w2324:T5)
            n923 = Enqueue Element(queue=w2326, element=w2324, error in (no error)=w2325) -> (queue out=w2323:refnum<queue>, error out=w2322:errorcluster)  [unwired: 1 in, 1 out]
          }
          frame #2 {
            n924 = for {
              N: 15 -> [w2338]
              i -> [w2337]
              stop <- w2333 stop-if-true
              n925 = Subtract(x=w2338, y=w2337) -> (x-y=w2336:i32)
              n926 = Decrement(x=w2336) -> (x-1=w2334:i32)
              n927 = Wait (ms)(milliseconds to wait=u32 1000) -> ()  [unwired: 1 out]
              n928 = local read "Network disconnected"() -> (w2333:bool)
              n929 = Select(t=0, s=w2333, f=w2334) -> (s? t:f=→"Flush Target Tank\nTime Remain (sec)":i32)
            }
          }
          frame #3 {
            w2347 = FALSE
            n930 = Bundle(cluster=T5 {"Message"="", "Message Data"=variant} ("Message Cluster"), "Message"="V4" ("Message 3"), "Message Data"=w2347) -> (w2342:T5)
            n931 = local write "eV4"(w2347) -> ()
            n932 = Enqueue Element(queue=w2343, element=w2342, error in (no error)=w2344) -> (queue out=w2346:refnum<queue>, error out=w2345:errorcluster)  [unwired: 1 in, 1 out]
          }
          frame #4 {
            w2349 = 0.0 ("MFC_1\nSLPM Value")
            n933 = local write "MFC_1\nSLPM Value"(w2349) -> ()
            n934 = Bundle(cluster=T5 {"Message"="", "Message Data"=variant} ("Message Cluster"), "Message"="MFC_1", "Message Data"=w2349) -> (w2353:T5)
            n935 = Enqueue Element(queue=w2351, element=w2353, error in (no error)=w2350) -> (error out=w2348:errorcluster)  [unwired: 1 in, 2 out]
          }
          frame #5 {
            n936 = local write "Flush Target Tank"(FALSE ("High Cal")) -> ()
          }
        }
      }
      event "Low Cal": Value Change {
        n937 = event-data() -> ()  [unwired: 1 in, 1 out]
        n938 = flat-sequence {
          tunnel: w2368 -> [w2373]
          tunnel: w2367 -> [w2372]
          tunnel: [w2371] -> w2366
          tunnel: [w2370] -> w2365
          tunnel: w2366 -> [w2389]
          tunnel: w2365 -> [w2388]
          tunnel: [w2386] -> w2364
          tunnel: [w2385] -> w2363
          tunnel: [w2394] -> w2362
          tunnel: [w2393] -> w2361
          tunnel: w2363 -> [w2397]
          tunnel: w2364 -> [w2398]
          tunnel: w2362 -> [w2451]
          tunnel: w2361 -> [w2450]
          tunnel: [w2448] -> w2360
          tunnel: [w2447] -> w2359
          tunnel: w2360 -> [w2465]
          tunnel: w2359 -> [w2464]
          tunnel: [w2462] -> w2357
          tunnel: [w2470] -> w2358
          tunnel: w2357 -> [w2470]
          frame #0 {
            w2369 = TRUE
            n939 = Cluster To Array(cluster=cluster{"Message":string, "Message 3":string} {"Message"="V2", "Message 3"="V4"}) -> (array=w2374:string[])
            n940 = for {
              tunnel: w2374 -> [w2381] mode=indexing
              tunnel: w2373 -> [w2380]
              tunnel: w2372 -> [w2379]
              tunnel: [w2378] -> w2371
              tunnel: [w2377] -> w2370
              tunnel: w2369 -> [w2376]
              n941 = Bundle(cluster=T5 {"Message"="", "Message Data"=variant} ("Message Cluster"), "Message"=w2381, "Message Data"=w2376) -> (w2383:T5)
              n942 = Enqueue Element(queue=w2380, element=w2383, error in (no error)=w2379) -> (queue out=w2378:refnum<queue>, error out=w2377:errorcluster)  [unwired: 1 in, 1 out]
            }
            n943 = local write "eV2"(w2369) -> ()
            n944 = local write "eV4"(w2369) -> ()
          }
          frame #1 {
            n945 = local read "MFC_1 User Set Value"() -> (w2384:dbl)
            n946 = local write "MFC_1\nSLPM Value"(w2384) -> ()
            n947 = Bundle(cluster=T5 {"Message"="", "Message Data"=variant} ("Message Cluster"), "Message"="MFC_1", "Message Data"=w2384) -> (w2387:T5)
            n948 = Enqueue Element(queue=w2389, element=w2387, error in (no error)=w2388) -> (queue out=w2386:refnum<queue>, error out=w2385:errorcluster)  [unwired: 1 in, 1 out]
          }
          frame #2 {
            n949 = for {
              N: 45 -> [w2441]
              tunnel: w2398 -> [w2432]
              tunnel: w2397 -> [w2431]
              tunnel: [w2432] -> w2396
              tunnel: [w2431] -> w2395
              tunnel: [w2430] -> w2392
              i -> [w2440]
              stop <- w2430 stop-if-true
              n950 = local read "FGGA Calibration Abort"() -> (w2435:bool)
              n951 = case shown="True" w2435 {
                selector: w2435 -> [w2444 _]
                tunnel: [w2444 w2445] -> w2433
                frame False {
                }
                frame True {
                  n952 = Two Button Dialog(message="Are you sure to abort FGGA Low Cal?") -> (T button?=w2445:bool)  [unwired: 2 in]
                }
              }
              n953 = local read "Network disconnected"() -> (w2434:bool)
              n954 = Subtract(x=w2441, y=w2440) -> (x-y=w2439:i32)
              n955 = Decrement(x=w2439) -> (x-1=w2437:i32)
              n956 = Wait (ms)(milliseconds to wait=u32 1000) -> ()  [unwired: 1 out]
              n957 = Or(x=w2434, y=w2433) -> (x .or. y?=w2430:bool)
              n958 = Select(t=0, s=w2430, f=w2437) -> (s? t:f=→"Low Cal\nFlush Time Remain (sec)":i32)
              n959 = case shown="False" w2433 {
                selector: w2433 -> [w2443 _]
                frame False {
                  n960 = local write "FGGA Calibration Abort"(w2443) -> ()
                }
                frame True {
                }
              }
            }
            n961 = case shown="False" w2392 {
              tunnel: w2396 -> [w2405 w2429]
              tunnel: w2395 -> [w2404 w2428]
              tunnel: [w2402 w2429] -> w2394
              tunnel: [w2400 w2428] -> w2393
              frame False {
                w2406 = TRUE
                # "Carry on if connection to cRIO is made\nor calibration not abort"
                n962 = Bundle(cluster=T5 {"Message"="", "Message Data"=variant} ("Message Cluster"), "Message"="V1", "Message Data"=w2406) -> (w2407:T5)
                n963 = local write "eV1"(w2406) -> ()
                n964 = Enqueue Element(queue=w2405, element=w2407, error in (no error)=w2404) -> (queue out=w2403:refnum<queue>, error out=w2401:errorcluster)  [unwired: 1 in, 1 out]
                n965 = for {
                  N: 60 -> [w2422]
                  tunnel: w2403 -> [w2412]
                  tunnel: [w2412] -> w2402
                  tunnel: w2401 -> [w2411]
                  tunnel: [w2411] -> w2400
                  i -> [w2421]
                  stop <- w2413 stop-if-true
                  n966 = Subtract(x=w2422, y=w2421) -> (x-y=w2420:i32)
                  n967 = local read "FGGA Calibration Abort"() -> (w2415:bool)
                  n968 = case shown="True" w2415 {
                    selector: w2415 -> [w2425 _]
                    tunnel: [w2425 w2426] -> w2414
                    frame False {
                    }
                    frame True {
                      n969 = Two Button Dialog(message="Are you sure to abort FGGA Low Cal?") -> (T button?=w2426:bool)  [unwired: 2 in]
                    }
                  }
                  n970 = Decrement(x=w2420) -> (x-1=w2417:i32)
                  n971 = Wait (ms)(milliseconds to wait=u32 1000) -> ()  [unwired: 1 out]
                  n972 = local read "Network disconnected"() -> (w2416:bool)
                  n973 = Or(x=w2416, y=w2414) -> (x .or. y?=w2413:bool)
                  n974 = case shown="False" w2414 {
                    selector: w2414 -> [w2424 _]
                    frame False {
                      n975 = local write "FGGA Calibration Abort"(w2424) -> ()
                    }
                    frame True {
                    }
                  }
                  n976 = Select(t=0, s=w2413, f=w2417) -> (s? t:f=→"Low Cal\nCal Time Remain (sec)":i32)
                }
              }
              frame True {
              }
            }
          }
          frame #3 {
            w2449 = FALSE
            n977 = Cluster To Array(cluster=T14 {"Message"="V2", "Message 3"="V4", "Message 4"="V1"}) -> (array=w2452:string[])
            n978 = for {
              tunnel: w2452 -> [w2459] mode=indexing
              tunnel: [w2458] -> w2448
              tunnel: [w2457] -> w2447
              tunnel: w2449 -> [w2456]
              tunnel: w2451 -> [w2455]
              tunnel: w2450 -> [w2454]
              n979 = Bundle(cluster=T5 {"Message"="", "Message Data"=variant} ("Message Cluster"), "Message"=w2459, "Message Data"=w2456) -> (w2461:T5)
              n980 = Enqueue Element(queue=w2455, element=w2461, error in (no error)=w2454) -> (queue out=w2458:refnum<queue>, error out=w2457:errorcluster)  [unwired: 1 in, 1 out]
            }
            n981 = local write "eV2"(w2449) -> ()
            n982 = local write "eV4"(w2449) -> ()
            n983 = local write "eV1"(w2449) -> ()
          }
          frame #4 {
            w2463 = 0.0 ("MFC_1\nSLPM Value")
            n984 = local write "MFC_1\nSLPM Value"(w2463) -> ()
            n985 = Bundle(cluster=T5 {"Message"="", "Message Data"=variant} ("Message Cluster"), "Message"="MFC_1", "Message Data"=w2463) -> (w2467:T5)
            n986 = Enqueue Element(queue=w2465, element=w2467, error in (no error)=w2464) -> (error out=w2462:errorcluster)  [unwired: 1 in, 2 out]
          }
          frame #5 {
            w2469 = FALSE ("High Cal")
            n987 = local write "Low Cal"(w2469) -> ()
            n988 = local write "FGGA Calibration Abort"(w2469) -> ()
          }
        }
      }
      event "Low Cal\n140 Torr": Value Change {
        n989 = event-data() -> ()  [unwired: 1 in, 1 out]
        n990 = flat-sequence {
          tunnel: w2493 -> [w2498]
          tunnel: w2492 -> [w2497]
          tunnel: [w2496] -> w2491
          tunnel: [w2495] -> w2490
          tunnel: w2491 -> [w2514]
          tunnel: w2490 -> [w2513]
          tunnel: [w2511] -> w2480
          tunnel: [w2510] -> w2481
          tunnel: w2481 -> [w2520]
          tunnel: w2480 -> [w2521]
          tunnel: [w2519] -> w2479
          tunnel: [w2518] -> w2478
          tunnel: [w2517] -> w2472
          tunnel: w2479 -> [w2544]
          tunnel: w2478 -> [w2543]
          tunnel: [w2542] -> w2477
          tunnel: [w2541] -> w2476
          tunnel: [w2540] -> w2473
          tunnel: w2472 -> [w2540]
          tunnel: w2477 -> [w2605]
          tunnel: w2476 -> [w2604]
          tunnel: [w2603] -> w2475
          tunnel: [w2602] -> w2474
          tunnel: w2473 -> [w2600]
          tunnel: [w2599] -> w2471
          tunnel: [w2628] -> w2489
          tunnel: [w2627] -> w2488
          tunnel: w2475 -> [w2626]
          tunnel: w2474 -> [w2625]
          tunnel: w2471 -> [w2624]
          tunnel: w2489 -> [w2663]
          tunnel: w2488 -> [w2662]
          tunnel: [w2660] -> w2487
          tunnel: [w2659] -> w2486
          tunnel: w2487 -> [w2678]
          tunnel: w2486 -> [w2677]
          tunnel: [w2675] -> w2484
          tunnel: [w2674] -> w2482
          tunnel: w2484 -> [w2684]
          tunnel: [w2683] -> w2483
          tunnel: w2482 -> [w2686]
          tunnel: [w2747] -> w2485
          tunnel: w2483 -> [w2747]
          frame #0 {
            w2494 = TRUE
            n991 = Cluster To Array(cluster=cluster{"Message":string, "Message 3":string} {"Message"="V2", "Message 3"="V4"}) -> (array=w2499:string[])
            n992 = for {
              tunnel: w2499 -> [w2506] mode=indexing
              tunnel: w2498 -> [w2505]
              tunnel: w2497 -> [w2504]
              tunnel: [w2503] -> w2496
              tunnel: [w2502] -> w2495
              tunnel: w2494 -> [w2501]
              n993 = Bundle(cluster=T5 {"Message"="", "Message Data"=variant} ("Message Cluster"), "Message"=w2506, "Message Data"=w2501) -> (w2508:T5)
              n994 = Enqueue Element(queue=w2505, element=w2508, error in (no error)=w2504) -> (queue out=w2503:refnum<queue>, error out=w2502:errorcluster)  [unwired: 1 in, 1 out]
            }
            n995 = local write "eV2"(w2494) -> ()
            n996 = local write "eV4"(w2494) -> ()
          }
          frame #1 {
            n997 = local read "MFC_1 140 Torr\nUser Set Value"() -> (w2509:dbl)
            n998 = local write "MFC_1\nSLPM Value"(w2509) -> ()
            n999 = Bundle(cluster=T5 {"Message"="", "Message Data"=variant} ("Message Cluster"), "Message"="MFC_1", "Message Data"=w2509) -> (w2512:T5)
            n1000 = Enqueue Element(queue=w2514, element=w2512, error in (no error)=w2513) -> (queue out=w2511:refnum<queue>, error out=w2510:errorcluster)  [unwired: 1 in, 1 out]
          }
          frame #2 {
            n1001 = local read "Span High, High, Low, Target Cal\nFlush Start Time (seconds)"() -> (w2522:i32)
            n1002 = for {
              N: w2522 -> [w2534]
              tunnel: w2521 -> [w2526]
              tunnel: w2520 -> [w2525]
              tunnel: [w2526] -> w2519
              tunnel: [w2525] -> w2518
              tunnel: [w2524] -> w2517
              i -> [w2533]
              stop <- w2524 stop-if-true
              n1003 = local read "FGGA 140 Torr\nCalibration Abort"() -> (w2529:bool)
              n1004 = case shown="True" w2529 {
                selector: w2529 -> [w2537 _]
                tunnel: [w2537 w2538] -> w2527
                frame False {
                }
                frame True {
                  n1005 = Two Button Dialog(message="Are you sure to abort FGGA Low Cal?") -> (T button?=w2538:bool)  [unwired: 2 in]
                }
              }
              n1006 = local read "Network disconnected"() -> (w2528:bool)
              n1007 = Subtract(x=w2534, y=w2533) -> (x-y=w2532:i32)
              n1008 = Decrement(x=w2532) -> (x-1=w2531:i32)
              n1009 = Wait (ms)(milliseconds to wait=u32 1000) -> ()  [unwired: 1 out]
              n1010 = Or(x=w2528, y=w2527) -> (x .or. y?=w2524:bool)
              n1011 = Select(t=0, s=w2524, f=w2531) -> (s? t:f=→"Low Cal 140 Torr\nFlush Time Remain (sec)":i32)
              n1012 = case shown="False" w2527 {
                selector: w2527 -> [w2536 _]
                frame False {
                  n1013 = local write "FGGA 140 Torr\nCalibration Abort"(w2536) -> ()
                }
                frame True {
                }
              }
            }
          }
          frame #3 {
            # "High to Low Flow"
            n1014 = flat-sequence {
              tunnel: w2544 -> [w2561]
              tunnel: w2543 -> [w2560]
              tunnel: [w2559] -> w2557
              tunnel: [w2558] -> w2556
              tunnel: [w2568] -> w2555
              tunnel: w2557 -> [w2568]
              tunnel: [w2567] -> w2554
              tunnel: w2556 -> [w2567]
              tunnel: w2545 -> [w2566]
              tunnel: w2555 -> [w2572]
              tunnel: w2554 -> [w2571]
              tunnel: [w2570] -> w2553
              tunnel: [w2569] -> w2552
              tunnel: [w2579] -> w2551
              tunnel: w2553 -> [w2579]
              tunnel: [w2578] -> w2550
              tunnel: w2552 -> [w2578]
              tunnel: w2545 -> [w2577]
              tunnel: w2551 -> [w2583]
              tunnel: w2550 -> [w2582]
              tunnel: [w2581] -> w2549
              tunnel: [w2580] -> w2548
              tunnel: [w2590] -> w2547
              tunnel: w2549 -> [w2590]
              tunnel: w2548 -> [w2589]
              tunnel: [w2589] -> w2546
              tunnel: w2545 -> [w2588]
              tunnel: w2547 -> [w2594]
              tunnel: w2546 -> [w2593]
              tunnel: [w2592] -> w2542
              tunnel: [w2591] -> w2541
              frame #0 {
                w2564 = FALSE
                n1015 = Bundle(cluster=T5 {"Message"="", "Message Data"=variant} ("Message Cluster"), "Message"="V10", "Message Data"=w2564) -> (w2563:T5)
                n1016 = local write "eV10"(w2564) -> ()
                n1017 = Enqueue Element(queue=w2561, element=w2563, error in (no error)=w2560) -> (queue out=w2559:refnum<queue>, error out=w2558:errorcluster)  [unwired: 1 in, 1 out]
              }
              frame #1 {
                n1018 = Wait (ms)(milliseconds to wait=w2566) -> ()  [unwired: 1 out]
              }
              frame #2 {
                w2573 = FALSE
                n1019 = local write "eV12"(w2573) -> ()
                n1020 = Bundle(cluster=T5 {"Message"="", "Message Data"=variant} ("Message Cluster"), "Message"="V12" ("Message 2"), "Message Data"=w2573) -> (w2576:T5)
                n1021 = Enqueue Element(queue=w2572, element=w2576, error in (no error)=w2571) -> (queue out=w2570:refnum<queue>, error out=w2569:errorcluster)  [unwired: 1 in, 1 out]
              }
              frame #3 {
                n1022 = Wait (ms)(milliseconds to wait=w2577) -> ()  [unwired: 1 out]
              }
              frame #4 {
                w2587 = TRUE
                n1023 = local write "eV11"(w2587) -> ()
                n1024 = Bundle(cluster=T5 {"Message"="", "Message Data"=variant} ("Message Cluster"), "Message"="V11" ("Message 2"), "Message Data"=w2587) -> (w2586:T5)
                n1025 = Enqueue Element(queue=w2583, element=w2586, error in (no error)=w2582) -> (queue out=w2580:refnum<queue>, error out=w2581:errorcluster)  [unwired: 1 in, 1 out]
              }
              frame #5 {
                n1026 = Wait (ms)(milliseconds to wait=w2588) -> ()  [unwired: 1 out]
              }
              frame #6 {
                n1027 = Bundle(cluster=T5 {"Message"="", "Message Data"=variant} ("Message Cluster"), "Message"="FGGA_pump", "Message Data"=TRUE) -> (w2595:T5)
                n1028 = Enqueue Element(queue=w2593, element=w2595, error in (no error)=w2594) -> (queue out=w2592:refnum<queue>, error out=w2591:errorcluster)  [unwired: 1 in, 1 out]
              }
            }
            n1029 = local read "Time delay (msec) between\nvalves switching"() -> (w2545:u32)
          }
          frame #4 {
            n1030 = local read "Span High, High, Low, Target  Cal\nContinue Flush Time (seconds)"() -> (w2606:i32)
            n1031 = for {
              N: w2606 -> [w2618]
              tunnel: w2605 -> [w2610]
              tunnel: w2604 -> [w2609]
              tunnel: [w2610] -> w2603
              tunnel: [w2609] -> w2602
              tunnel: [w2608] -> w2601
              i -> [w2617]
              stop <- w2608 stop-if-true
              n1032 = local read "FGGA 140 Torr\nCalibration Abort"() -> (w2613:bool)
              n1033 = case shown="True" w2613 {
                selector: w2613 -> [w2621 _]
                tunnel: [w2621 w2622] -> w2611
                frame False {
                }
                frame True {
                  n1034 = Two Button Dialog(message="Are you sure to abort FGGA Low Cal?") -> (T button?=w2622:bool)  [unwired: 2 in]
                }
              }
              n1035 = Subtract(x=w2618, y=w2617) -> (x-y=w2616:i32)
              n1036 = Decrement(x=w2616) -> (x-1=w2615:i32)
              n1037 = local read "Network disconnected"() -> (w2612:bool)
              n1038 = Wait (ms)(milliseconds to wait=u32 1000) -> ()  [unwired: 1 out]
              n1039 = Or(x=w2612, y=w2611) -> (x .or. y?=w2608:bool)
              n1040 = Select(t=0, s=w2608, f=w2615) -> (s? t:f=w2607:i32)
              n1041 = local write "Low Cal 140 Torr\nFlush Time Remain (sec)"(w2607) -> ()
              n1042 = case shown="False" w2611 {
                selector: w2611 -> [w2620 _]
                frame False {
                  n1043 = local write "FGGA 140 Torr\nCalibration Abort"(w2620) -> ()
                }
                frame True {
                }
              }
            }
            n1044 = Or(x=w2601, y=w2600) -> (x .or. y?=w2599:bool)
          }
          frame #5 {
            n1045 = case shown="False" w2624 {
              tunnel: w2626 -> [w2631 w2658]
              tunnel: w2625 -> [w2630 w2657]
              tunnel: [w2639 w2658] -> w2628
              tunnel: [w2638 w2657] -> w2627
              frame False {
                w2634 = TRUE
                # "Carry on if connection to cRIO is made\nor calibration not abort"
                n1046 = local read "Span High, High Low, Target\nCal Time (seconds)"() -> (w2629:i32)
                n1047 = Bundle(cluster=T5 {"Message"="", "Message Data"=variant} ("Message Cluster"), "Message"="V1", "Message Data"=w2634) -> (w2635:T5)
                n1048 = local write "eV1"(w2634) -> ()
                n1049 = Enqueue Element(queue=w2631, element=w2635, error in (no error)=w2630) -> (queue out=w2632:refnum<queue>, error out=w2633:errorcluster)  [unwired: 1 in, 1 out]
                n1050 = for {
                  N: w2629 -> [w2651]
                  tunnel: w2632 -> [w2642]
                  tunnel: [w2642] -> w2639
                  tunnel: w2633 -> [w2641]
                  tunnel: [w2641] -> w2638
                  i -> [w2650]
                  stop <- w2643 stop-if-true
                  n1051 = Subtract(x=w2651, y=w2650) -> (x-y=w2649:i32)
                  n1052 = local read "FGGA 140 Torr\nCalibration Abort"() -> (w2645:bool)
                  n1053 = case shown="True" w2645 {
                    selector: w2645 -> [w2654 _]
                    tunnel: [w2654 w2655] -> w2644
                    frame False {
                    }
                    frame True {
                      n1054 = Two Button Dialog(message="Are you sure to abort FGGA Low Cal?") -> (T button?=w2655:bool)  [unwired: 2 in]
                    }
                  }
                  n1055 = Decrement(x=w2649) -> (x-1=w2647:i32)
                  n1056 = local read "Network disconnected"() -> (w2646:bool)
                  n1057 = Wait (ms)(milliseconds to wait=u32 1000) -> ()  [unwired: 1 out]
                  n1058 = Or(x=w2646, y=w2644) -> (x .or. y?=w2643:bool)
                  n1059 = case shown="False" w2644 {
                    selector: w2644 -> [w2653 _]
                    frame False {
                      n1060 = local write "FGGA 140 Torr\nCalibration Abort"(w2653) -> ()
                    }
                    frame True {
                    }
                  }
                  n1061 = Select(t=0, s=w2643, f=w2647) -> (s? t:f=→"Low Cal 140 Torr\nCal Time Remain (sec)":i32)
                }
              }
              frame True {
              }
            }
          }
          frame #6 {
            w2661 = FALSE
            n1062 = Cluster To Array(cluster=T14 {"Message"="V2", "Message 3"="V4", "Message 4"="V1"}) -> (array=w2664:string[])
            n1063 = for {
              tunnel: w2664 -> [w2671] mode=indexing
              tunnel: [w2670] -> w2660
              tunnel: [w2669] -> w2659
              tunnel: w2661 -> [w2668]
              tunnel: w2663 -> [w2667]
              tunnel: w2662 -> [w2666]
              n1064 = Bundle(cluster=T5 {"Message"="", "Message Data"=variant} ("Message Cluster"), "Message"=w2671, "Message Data"=w2668) -> (w2673:T5)
              n1065 = Enqueue Element(queue=w2667, element=w2673, error in (no error)=w2666) -> (queue out=w2670:refnum<queue>, error out=w2669:errorcluster)  [unwired: 1 in, 1 out]
            }
            n1066 = local write "eV2"(w2661) -> ()
            n1067 = local write "eV4"(w2661) -> ()
            n1068 = local write "eV1"(w2661) -> ()
          }
          frame #7 {
            w2676 = 0.0 ("MFC_1\nSLPM Value")
            n1069 = local write "MFC_1\nSLPM Value"(w2676) -> ()
            n1070 = Bundle(cluster=T5 {"Message"="", "Message Data"=variant} ("Message Cluster"), "Message"="MFC_1", "Message Data"=w2676) -> (w2680:T5)
            n1071 = Enqueue Element(queue=w2678, element=w2680, error in (no error)=w2677) -> (queue out=w2674:refnum<queue>, error out=w2675:errorcluster)  [unwired: 1 in, 1 out]
          }
          frame #8 {
            # "Set back to high flow only if High Flow master switch is ON"
            n1072 = local read "Time delay (msec) between\nvalves switching"() -> (w2682:u32)
            n1073 = local read "HIGH FLOW MASTER SWITCH"() -> (w2685:bool)
            n1074 = case shown="True" w2685 {
              tunnel: w2686 -> [_ w2705]
              tunnel: w2684 -> [w2687 w2704]
              tunnel: [w2687 w2691] -> w2683
              tunnel: w2682 -> [_ w2690]
              tunnel: w2682 -> [_ w2689]
              tunnel: w2682 -> [_ w2688]
              frame False {
              }
              frame True {
                n1075 = flat-sequence {
                  tunnel: w2705 -> [w2709]
                  tunnel: w2704 -> [w2708]
                  tunnel: [w2707] -> w2702
                  tunnel: [w2706] -> w2700
                  tunnel: [w2716] -> w2703
                  tunnel: w2702 -> [w2716]
                  tunnel: [w2715] -> w2701
                  tunnel: w2700 -> [w2715]
                  tunnel: w2690 -> [w2714]
                  tunnel: w2703 -> [w2720]
                  tunnel: w2701 -> [w2719]
                  tunnel: [w2718] -> w2698
                  tunnel: [w2717] -> w2696
                  tunnel: [w2727] -> w2699
                  tunnel: w2698 -> [w2727]
                  tunnel: [w2726] -> w2697
                  tunnel: w2696 -> [w2726]
                  tunnel: w2689 -> [w2725]
                  tunnel: w2699 -> [w2732]
                  tunnel: w2697 -> [w2731]
                  tunnel: [w2730] -> w2694
                  tunnel: [w2729] -> w2692
                  tunnel: [w2738] -> w2695
                  tunnel: w2694 -> [w2738]
                  tunnel: [w2737] -> w2693
                  tunnel: w2692 -> [w2737]
                  tunnel: w2688 -> [w2736]
                  tunnel: w2695 -> [w2741]
                  tunnel: w2693 -> [w2740]
                  tunnel: [w2739] -> w2691
                  frame #0 {
                    n1076 = Bundle(cluster=T5 {"Message"="", "Message Data"=variant} ("Message Cluster"), "Message"="FGGA_pump", "Message Data"=FALSE) -> (w2710:T5)
                    n1077 = Enqueue Element(queue=w2709, element=w2710, error in (no error)=w2708) -> (queue out=w2707:refnum<queue>, error out=w2706:errorcluster)  [unwired: 1 in, 1 out]
                  }
                  frame #1 {
                    n1078 = Wait (ms)(milliseconds to wait=w2714) -> ()  [unwired: 1 out]
                  }
                  frame #2 {
                    w2724 = FALSE
                    n1079 = local write "eV11"(w2724) -> ()
                    n1080 = Bundle(cluster=T5 {"Message"="", "Message Data"=variant} ("Message Cluster"), "Message"="V11" ("Message 2"), "Message Data"=w2724) -> (w2723:T5)
                    n1081 = Enqueue Element(queue=w2720, element=w2723, error in (no error)=w2719) -> (queue out=w2717:refnum<queue>, error out=w2718:errorcluster)  [unwired: 1 in, 1 out]
                  }
                  frame #3 {
                    n1082 = Wait (ms)(milliseconds to wait=w2725) -> ()  [unwired: 1 out]
                  }
                  frame #4 {
                    w2728 = TRUE
                    n1083 = local write "eV12"(w2728) -> ()
                    n1084 = Bundle(cluster=T5 {"Message"="", "Message Data"=variant} ("Message Cluster"), "Message"="V12" ("Message 2"), "Message Data"=w2728) -> (w2735:T5)
                    n1085 = Enqueue Element(queue=w2731, element=w2735, error in (no error)=w2732) -> (queue out=w2730:refnum<queue>, error out=w2729:errorcluster)  [unwired: 1 in, 1 out]
                  }
                  frame #5 {
                    n1086 = Wait (ms)(milliseconds to wait=w2736) -> ()  [unwired: 1 out]
                  }
                  frame #6 {
                    w2742 = TRUE
                    n1087 = local write "eV10"(w2742) -> ()
                    n1088 = Bundle(cluster=T5 {"Message"="", "Message Data"=variant} ("Message Cluster"), "Message"="V10", "Message Data"=w2742) -> (w2745:T5)
                    n1089 = Enqueue Element(queue=w2741, element=w2745, error in (no error)=w2740) -> (error out=w2739:errorcluster)  [unwired: 1 in, 2 out]
                  }
                }
              }
            }
          }
          frame #9 {
            w2746 = FALSE ("High Cal")
            n1090 = local write "FGGA 140 Torr\nCalibration Abort"(w2746) -> ()
            n1091 = local write "Low Cal\n140 Torr"(w2746) -> ()
          }
        }
      }
      event "Target Cal": Value Change {
        n1092 = event-data() -> ()  [unwired: 1 in, 1 out]
        n1093 = flat-sequence {
          tunnel: w2759 -> [w2767]
          tunnel: w2758 -> [w2766]
          tunnel: [w2765] -> w2757
          tunnel: [w2764] -> w2756
          tunnel: w2757 -> [w2773]
          tunnel: w2756 -> [w2772]
          tunnel: [w2770] -> w2755
          tunnel: [w2769] -> w2754
          tunnel: w2754 -> [w2780]
          tunnel: w2755 -> [w2781]
          tunnel: [w2778] -> w2749
          tunnel: [w2777] -> w2748
          tunnel: [w2833] -> w2753
          tunnel: [w2834] -> w2752
          tunnel: w2749 -> [w2832]
          tunnel: w2748 -> [w2831]
          tunnel: w2753 -> [w2849]
          tunnel: w2752 -> [w2848]
          tunnel: [w2846] -> w2750
          tunnel: [w2854] -> w2751
          tunnel: w2750 -> [w2854]
          frame #0 {
            w2763 = TRUE
            n1094 = local write "eV4"(w2763) -> ()
            n1095 = Bundle(cluster=T5 {"Message"="", "Message Data"=variant} ("Message Cluster"), "Message"="V4" ("Message 3"), "Message Data"=w2763) -> (w2762:T5)
            n1096 = Enqueue Element(queue=w2767, element=w2762, error in (no error)=w2766) -> (queue out=w2765:refnum<queue>, error out=w2764:errorcluster)  [unwired: 1 in, 1 out]
          }
          frame #1 {
            n1097 = local read "MFC_1 User Set Value"() -> (w2768:dbl)
            n1098 = local write "MFC_1\nSLPM Value"(w2768) -> ()
            n1099 = Bundle(cluster=T5 {"Message"="", "Message Data"=variant} ("Message Cluster"), "Message"="MFC_1", "Message Data"=w2768) -> (w2771:T5)
            n1100 = Enqueue Element(queue=w2773, element=w2771, error in (no error)=w2772) -> (queue out=w2770:refnum<queue>, error out=w2769:errorcluster)  [unwired: 1 in, 1 out]
          }
          frame #2 {
            n1101 = for {
              N: 45 -> [w2825]
              tunnel: [w2816] -> w2782
              tunnel: w2781 -> [w2816]
              tunnel: [w2815] -> w2779
              tunnel: w2780 -> [w2815]
              tunnel: [w2814] -> w2776
              i -> [w2824]
              stop <- w2814 stop-if-true
              n1102 = Subtract(x=w2825, y=w2824) -> (x-y=w2823:i32)
              n1103 = Decrement(x=w2823) -> (x-1=w2820:i32)
              n1104 = local read "FGGA Calibration Abort"() -> (w2819:bool)
              n1105 = local read "Network disconnected"() -> (w2818:bool)
              n1106 = case shown="True" w2819 {
                selector: w2819 -> [w2828 _]
                tunnel: [w2828 w2829] -> w2817
                frame False {
                }
                frame True {
                  n1107 = Two Button Dialog(message="Are you sure to abort FGGA Target Cal?") -> (T button?=w2829:bool)  [unwired: 2 in]
                }
              }
              n1108 = Wait (ms)(milliseconds to wait=u32 1000) -> ()  [unwired: 1 out]
              n1109 = Or(x=w2818, y=w2817) -> (x .or. y?=w2814:bool)
              n1110 = Select(t=0, s=w2814, f=w2820) -> (s? t:f=→"Target Cal\nFlush Time Remain (sec)":i32)
              n1111 = case shown="False" w2817 {
                selector: w2817 -> [w2827 _]
                frame False {
                  n1112 = local write "FGGA Calibration Abort"(w2827) -> ()
                }
                frame True {
                }
              }
            }
            n1113 = case shown="False" w2776 {
              tunnel: w2782 -> [w2789 w2813]
              tunnel: w2779 -> [w2788 w2812]
              tunnel: [w2785 w2813] -> w2778
              tunnel: [w2784 w2812] -> w2777
              frame False {
                w2790 = TRUE
                # "Carry on if connection to cRIO is made\nor calibration not abort"
                n1114 = Bundle(cluster=T5 {"Message"="", "Message Data"=variant} ("Message Cluster"), "Message"="V1", "Message Data"=w2790) -> (w2791:T5)
                n1115 = local write "eV1"(w2790) -> ()
                n1116 = Enqueue Element(queue=w2789, element=w2791, error in (no error)=w2788) -> (queue out=w2787:refnum<queue>, error out=w2786:errorcluster)  [unwired: 1 in, 1 out]
                n1117 = for {
                  N: 60 -> [w2806]
                  tunnel: w2787 -> [w2796]
                  tunnel: w2786 -> [w2795]
                  tunnel: [w2796] -> w2785
                  tunnel: [w2795] -> w2784
                  i -> [w2805]
                  stop <- w2797 stop-if-true
                  n1118 = Subtract(x=w2806, y=w2805) -> (x-y=w2804:i32)
                  n1119 = Decrement(x=w2804) -> (x-1=w2802:i32)
                  n1120 = local read "FGGA Calibration Abort"() -> (w2800:bool)
                  n1121 = Wait (ms)(milliseconds to wait=u32 1000) -> ()  [unwired: 1 out]
                  n1122 = local read "Network disconnected"() -> (w2799:bool)
                  n1123 = case shown="True" w2800 {
                    selector: w2800 -> [w2809 _]
                    tunnel: [w2809 w2810] -> w2798
                    frame False {
                    }
                    frame True {
                      n1124 = Two Button Dialog(message="Are you sure to abort FGGA Target Cal?") -> (T button?=w2810:bool)  [unwired: 2 in]
                    }
                  }
                  n1125 = Or(x=w2799, y=w2798) -> (x .or. y?=w2797:bool)
                  n1126 = case shown="False" w2798 {
                    selector: w2798 -> [w2808 _]
                    frame False {
                      n1127 = local write "FGGA Calibration Abort"(w2808) -> ()
                    }
                    frame True {
                    }
                  }
                  n1128 = Select(t=0, s=w2797, f=w2802) -> (s? t:f=→"Target Cal\nCal Time Remain (sec)":i32)
                }
              }
              frame True {
              }
            }
          }
          frame #3 {
            w2837 = FALSE
            n1129 = Cluster To Array(cluster=cluster{"Message 3":string, "Message":string} {"Message 3"="V4", "Message"="V1"}) -> (array=w2835:string[])
            n1130 = for {
              tunnel: w2835 -> [w2843] mode=indexing
              tunnel: [w2842] -> w2833
              tunnel: [w2841] -> w2834
              tunnel: w2837 -> [w2840]
              tunnel: w2832 -> [w2839]
              tunnel: w2831 -> [w2838]
              n1131 = Bundle(cluster=T5 {"Message"="", "Message Data"=variant} ("Message Cluster"), "Message"=w2843, "Message Data"=w2840) -> (w2845:T5)
              n1132 = Enqueue Element(queue=w2839, element=w2845, error in (no error)=w2838) -> (queue out=w2842:refnum<queue>, error out=w2841:errorcluster)  [unwired: 1 in, 1 out]
            }
            n1133 = local write "eV4"(w2837) -> ()
            n1134 = local write "eV1"(w2837) -> ()
          }
          frame #4 {
            w2847 = 0.0 ("MFC_1\nSLPM Value")
            n1135 = local write "MFC_1\nSLPM Value"(w2847) -> ()
            n1136 = Bundle(cluster=T5 {"Message"="", "Message Data"=variant} ("Message Cluster"), "Message"="MFC_1", "Message Data"=w2847) -> (w2851:T5)
            n1137 = Enqueue Element(queue=w2849, element=w2851, error in (no error)=w2848) -> (error out=w2846:errorcluster)  [unwired: 1 in, 2 out]
          }
          frame #5 {
            w2853 = FALSE ("High Cal")
            n1138 = local write "Target Cal"(w2853) -> ()
            n1139 = local write "FGGA Calibration Abort"(w2853) -> ()
          }
        }
      }
      event "Target Cal\n140 Torr": Value Change {
        n1140 = event-data() -> ()  [unwired: 1 in, 1 out]
        n1141 = flat-sequence {
          tunnel: w2877 -> [w2885]
          tunnel: w2876 -> [w2884]
          tunnel: [w2883] -> w2875
          tunnel: [w2882] -> w2874
          tunnel: w2875 -> [w2891]
          tunnel: w2874 -> [w2890]
          tunnel: [w2888] -> w2864
          tunnel: [w2887] -> w2865
          tunnel: w2865 -> [w2897]
          tunnel: w2864 -> [w2898]
          tunnel: [w2896] -> w2863
          tunnel: [w2895] -> w2862
          tunnel: [w2894] -> w2856
          tunnel: w2863 -> [w2921]
          tunnel: w2862 -> [w2920]
          tunnel: [w2919] -> w2861
          tunnel: [w2918] -> w2860
          tunnel: [w2917] -> w2857
          tunnel: w2856 -> [w2917]
          tunnel: w2861 -> [w2982]
          tunnel: w2860 -> [w2981]
          tunnel: [w2980] -> w2859
          tunnel: [w2979] -> w2858
          tunnel: w2857 -> [w2977]
          tunnel: [w2976] -> w2855
          tunnel: [w3005] -> w2870
          tunnel: [w3004] -> w2869
          tunnel: w2859 -> [w3003]
          tunnel: w2858 -> [w3002]
          tunnel: w2855 -> [w3001]
          tunnel: [w3038] -> w2873
          tunnel: [w3039] -> w2872
          tunnel: w2870 -> [w3037]
          tunnel: w2869 -> [w3036]
          tunnel: w2873 -> [w3055]
          tunnel: w2872 -> [w3054]
          tunnel: [w3052] -> w2868
          tunnel: [w3051] -> w2866
          tunnel: w2868 -> [w3063]
          tunnel: [w3060] -> w2867
          tunnel: w2866 -> [w3062]
          tunnel: [w3124] -> w2871
          tunnel: w2867 -> [w3124]
          frame #0 {
            w2881 = TRUE
            n1142 = local write "eV4"(w2881) -> ()
            n1143 = Bundle(cluster=T5 {"Message"="", "Message Data"=variant} ("Message Cluster"), "Message"="V4" ("Message 3"), "Message Data"=w2881) -> (w2880:T5)
            n1144 = Enqueue Element(queue=w2885, element=w2880, error in (no error)=w2884) -> (queue out=w2883:refnum<queue>, error out=w2882:errorcluster)  [unwired: 1 in, 1 out]
          }
          frame #1 {
            n1145 = local read "MFC_1 140 Torr\nUser Set Value"() -> (w2886:dbl)
            n1146 = local write "MFC_1\nSLPM Value"(w2886) -> ()
            n1147 = Bundle(cluster=T5 {"Message"="", "Message Data"=variant} ("Message Cluster"), "Message"="MFC_1", "Message Data"=w2886) -> (w2889:T5)
            n1148 = Enqueue Element(queue=w2891, element=w2889, error in (no error)=w2890) -> (queue out=w2888:refnum<queue>, error out=w2887:errorcluster)  [unwired: 1 in, 1 out]
          }
          frame #2 {
            n1149 = local read "Span High, High, Low, Target Cal\nFlush Start Time (seconds)"() -> (w2899:i32)
            n1150 = for {
              N: w2899 -> [w2911]
              tunnel: [w2903] -> w2896
              tunnel: w2898 -> [w2903]
              tunnel: [w2902] -> w2895
              tunnel: w2897 -> [w2902]
              tunnel: [w2901] -> w2894
              i -> [w2910]
              stop <- w2901 stop-if-true
              n1151 = Subtract(x=w2911, y=w2910) -> (x-y=w2909:i32)
              n1152 = Decrement(x=w2909) -> (x-1=w2907:i32)
              n1153 = Wait (ms)(milliseconds to wait=u32 1000) -> ()  [unwired: 1 out]
              n1154 = local read "FGGA 140 Torr\nCalibration Abort"() -> (w2906:bool)
              n1155 = case shown="True" w2906 {
                selector: w2906 -> [w2914 _]
                tunnel: [w2914 w2915] -> w2904
                frame False {
                }
                frame True {
                  n1156 = Two Button Dialog(message="Are you sure to abort FGGA Target Cal?") -> (T button?=w2915:bool)  [unwired: 2 in]
                }
              }
              n1157 = local read "Network disconnected"() -> (w2905:bool)
              n1158 = Or(x=w2905, y=w2904) -> (x .or. y?=w2901:bool)
              n1159 = case shown="False" w2904 {
                selector: w2904 -> [w2913 _]
                frame False {
                  n1160 = local write "FGGA 140 Torr\nCalibration Abort"(w2913) -> ()
                }
                frame True {
                }
              }
              n1161 = Select(t=0, s=w2901, f=w2907) -> (s? t:f=→"Target Cal 140 Torr\nFlush Time Remain (sec)":i32)
            }
          }
          frame #3 {
            # "High to Low Flow"
            n1162 = flat-sequence {
              tunnel: w2921 -> [w2938]
              tunnel: [w2937] -> w2934
              tunnel: w2920 -> [w2936]
              tunnel: [w2935] -> w2933
              tunnel: [w2945] -> w2932
              tunnel: w2934 -> [w2945]
              tunnel: [w2944] -> w2931
              tunnel: w2933 -> [w2944]
              tunnel: w2922 -> [w2943]
              tunnel: w2932 -> [w2949]
              tunnel: [w2948] -> w2930
              tunnel: w2931 -> [w2947]
              tunnel: [w2946] -> w2929
              tunnel: [w2956] -> w2928
              tunnel: w2930 -> [w2956]
              tunnel: [w2955] -> w2927
              tunnel: w2929 -> [w2955]
              tunnel: w2922 -> [w2954]
              tunnel: w2928 -> [w2960]
              tunnel: [w2959] -> w2926
              tunnel: w2927 -> [w2958]
              tunnel: [w2957] -> w2925
              tunnel: [w2967] -> w2924
              tunnel: w2926 -> [w2967]
              tunnel: [w2966] -> w2923
              tunnel: w2925 -> [w2966]
              tunnel: w2922 -> [w2965]
              tunnel: w2924 -> [w2971]
              tunnel: w2923 -> [w2970]
              tunnel: [w2969] -> w2918
              tunnel: [w2968] -> w2919
              frame #0 {
                w2939 = FALSE
                n1163 = Bundle(cluster=T5 {"Message"="", "Message Data"=variant} ("Message Cluster"), "Message"="V10", "Message Data"=w2939) -> (w2942:T5)
                n1164 = local write "eV10"(w2939) -> ()
                n1165 = Enqueue Element(queue=w2938, element=w2942, error in (no error)=w2936) -> (queue out=w2937:refnum<queue>, error out=w2935:errorcluster)  [unwired: 1 in, 1 out]
              }
              frame #1 {
                n1166 = Wait (ms)(milliseconds to wait=w2943) -> ()  [unwired: 1 out]
              }
              frame #2 {
                w2950 = FALSE
                n1167 = local write "eV12"(w2950) -> ()
                n1168 = Bundle(cluster=T5 {"Message"="", "Message Data"=variant} ("Message Cluster"), "Message"="V12" ("Message 2"), "Message Data"=w2950) -> (w2953:T5)
                n1169 = Enqueue Element(queue=w2949, element=w2953, error in (no error)=w2947) -> (queue out=w2948:refnum<queue>, error out=w2946:errorcluster)  [unwired: 1 in, 1 out]
              }
              frame #3 {
                n1170 = Wait (ms)(milliseconds to wait=w2954) -> ()  [unwired: 1 out]
              }
              frame #4 {
                w2961 = TRUE
                n1171 = local write "eV11"(w2961) -> ()
                n1172 = Bundle(cluster=T5 {"Message"="", "Message Data"=variant} ("Message Cluster"), "Message"="V11" ("Message 2"), "Message Data"=w2961) -> (w2962:T5)
                n1173 = Enqueue Element(queue=w2960, element=w2962, error in (no error)=w2958) -> (queue out=w2959:refnum<queue>, error out=w2957:errorcluster)  [unwired: 1 in, 1 out]
              }
              frame #5 {
                n1174 = Wait (ms)(milliseconds to wait=w2965) -> ()  [unwired: 1 out]
              }
              frame #6 {
                n1175 = Bundle(cluster=T5 {"Message"="", "Message Data"=variant} ("Message Cluster"), "Message"="FGGA_pump", "Message Data"=TRUE) -> (w2975:T5)
                n1176 = Enqueue Element(queue=w2971, element=w2975, error in (no error)=w2970) -> (queue out=w2968:refnum<queue>, error out=w2969:errorcluster)  [unwired: 1 in, 1 out]
              }
            }
            n1177 = local read "Time delay (msec) between\nvalves switching"() -> (w2922:u32)
          }
          frame #4 {
            n1178 = local read "Span High, High, Low, Target  Cal\nContinue Flush Time (seconds)"() -> (w2983:i32)
            n1179 = for {
              N: w2983 -> [w2995]
              tunnel: [w2987] -> w2980
              tunnel: w2982 -> [w2987]
              tunnel: [w2986] -> w2979
              tunnel: w2981 -> [w2986]
              tunnel: [w2985] -> w2978
              i -> [w2994]
              stop <- w2985 stop-if-true
              n1180 = Subtract(x=w2995, y=w2994) -> (x-y=w2993:i32)
              n1181 = Decrement(x=w2993) -> (x-1=w2991:i32)
              n1182 = Wait (ms)(milliseconds to wait=u32 1000) -> ()  [unwired: 1 out]
              n1183 = local read "FGGA 140 Torr\nCalibration Abort"() -> (w2990:bool)
              n1184 = case shown="True" w2990 {
                selector: w2990 -> [w2998 _]
                tunnel: [w2998 w2999] -> w2988
                frame False {
                }
                frame True {
                  n1185 = Two Button Dialog(message="Are you sure to abort FGGA Target Cal?") -> (T button?=w2999:bool)  [unwired: 2 in]
                }
              }
              n1186 = local read "Network disconnected"() -> (w2989:bool)
              n1187 = Or(x=w2989, y=w2988) -> (x .or. y?=w2985:bool)
              n1188 = case shown="False" w2988 {
                selector: w2988 -> [w2997 _]
                frame False {
                  n1189 = local write "FGGA 140 Torr\nCalibration Abort"(w2997) -> ()
                }
                frame True {
                }
              }
              n1190 = Select(t=0, s=w2985, f=w2991) -> (s? t:f=w2984:i32)
              n1191 = local write "Target Cal 140 Torr\nFlush Time Remain (sec)"(w2984) -> ()
            }
            n1192 = Or(x=w2978, y=w2977) -> (x .or. y?=w2976:bool)
          }
          frame #5 {
            n1193 = case shown="True" w3001 {
              tunnel: [w3016 w3035] -> w3005
              tunnel: [w3015 w3034] -> w3004
              tunnel: w3003 -> [w3008 w3035]
              tunnel: w3002 -> [w3007 w3034]
              frame False {
                w3011 = TRUE
                # "Carry on if connection to cRIO is made\nor calibration not abort"
                n1194 = Bundle(cluster=T5 {"Message"="", "Message Data"=variant} ("Message Cluster"), "Message"="V1", "Message Data"=w3011) -> (w3012:T5)
                n1195 = local write "eV1"(w3011) -> ()
                n1196 = local read "Span High, High Low, Target\nCal Time (seconds)"() -> (w3006:i32)
                n1197 = Enqueue Element(queue=w3008, element=w3012, error in (no error)=w3007) -> (queue out=w3010:refnum<queue>, error out=w3009:errorcluster)  [unwired: 1 in, 1 out]
                n1198 = for {
                  N: w3006 -> [w3028]
                  tunnel: w3010 -> [w3019]
                  tunnel: w3009 -> [w3018]
                  tunnel: [w3019] -> w3016
                  tunnel: [w3018] -> w3015
                  i -> [w3027]
                  stop <- w3020 stop-if-true
                  n1199 = Subtract(x=w3028, y=w3027) -> (x-y=w3026:i32)
                  n1200 = Decrement(x=w3026) -> (x-1=w3024:i32)
                  n1201 = local read "FGGA 140 Torr\nCalibration Abort"() -> (w3023:bool)
                  n1202 = case shown="True" w3023 {
                    selector: w3023 -> [w3031 _]
                    tunnel: [w3031 w3032] -> w3021
                    frame False {
                    }
                    frame True {
                      n1203 = Two Button Dialog(message="Are you sure to abort FGGA Target Cal?") -> (T button?=w3032:bool)  [unwired: 2 in]
                    }
                  }
                  n1204 = Wait (ms)(milliseconds to wait=u32 1000) -> ()  [unwired: 1 out]
                  n1205 = local read "Network disconnected"() -> (w3022:bool)
                  n1206 = Or(x=w3022, y=w3021) -> (x .or. y?=w3020:bool)
                  n1207 = case shown="False" w3021 {
                    selector: w3021 -> [w3030 _]
                    frame False {
                      n1208 = local write "FGGA 140 Torr\nCalibration Abort"(w3030) -> ()
                    }
                    frame True {
                    }
                  }
                  n1209 = Select(t=0, s=w3020, f=w3024) -> (s? t:f=→"Target Cal 140 Torr\nCal Time Remain (sec)":i32)
                }
              }
              frame True {
              }
            }
          }
          frame #6 {
            w3042 = FALSE
            n1210 = Cluster To Array(cluster=cluster{"Message 3":string, "Message":string} {"Message 3"="V4", "Message"="V1"}) -> (array=w3040:string[])
            n1211 = for {
              tunnel: w3040 -> [w3048] mode=indexing
              tunnel: [w3047] -> w3038
              tunnel: [w3046] -> w3039
              tunnel: w3042 -> [w3045]
              tunnel: w3037 -> [w3044]
              tunnel: w3036 -> [w3043]
              n1212 = Bundle(cluster=T5 {"Message"="", "Message Data"=variant} ("Message Cluster"), "Message"=w3048, "Message Data"=w3045) -> (w3050:T5)
              n1213 = Enqueue Element(queue=w3044, element=w3050, error in (no error)=w3043) -> (queue out=w3047:refnum<queue>, error out=w3046:errorcluster)  [unwired: 1 in, 1 out]
            }
            n1214 = local write "eV4"(w3042) -> ()
            n1215 = local write "eV1"(w3042) -> ()
          }
          frame #7 {
            w3053 = 0.0 ("MFC_1\nSLPM Value")
            n1216 = local write "MFC_1\nSLPM Value"(w3053) -> ()
            n1217 = Bundle(cluster=T5 {"Message"="", "Message Data"=variant} ("Message Cluster"), "Message"="MFC_1", "Message Data"=w3053) -> (w3057:T5)
            n1218 = Enqueue Element(queue=w3055, element=w3057, error in (no error)=w3054) -> (queue out=w3051:refnum<queue>, error out=w3052:errorcluster)  [unwired: 1 in, 1 out]
          }
          frame #8 {
            # "Set back to high flow only if High Flow master switch is ON"
            n1219 = local read "HIGH FLOW MASTER SWITCH"() -> (w3061:bool)
            n1220 = local read "Time delay (msec) between\nvalves switching"() -> (w3059:u32)
            n1221 = case shown="True" w3061 {
              tunnel: w3062 -> [_ w3082]
              tunnel: w3063 -> [w3064 w3081]
              tunnel: [w3064 w3070] -> w3060
              tunnel: w3059 -> [_ w3067]
              tunnel: w3059 -> [_ w3066]
              tunnel: w3059 -> [_ w3065]
              frame False {
              }
              frame True {
                n1222 = flat-sequence {
                  tunnel: w3082 -> [w3086]
                  tunnel: w3081 -> [w3085]
                  tunnel: [w3084] -> w3079
                  tunnel: [w3083] -> w3077
                  tunnel: [w3093] -> w3080
                  tunnel: w3079 -> [w3093]
                  tunnel: [w3092] -> w3078
                  tunnel: w3077 -> [w3092]
                  tunnel: w3067 -> [w3091]
                  tunnel: w3080 -> [w3097]
                  tunnel: w3078 -> [w3096]
                  tunnel: [w3095] -> w3075
                  tunnel: [w3094] -> w3073
                  tunnel: [w3104] -> w3076
                  tunnel: w3075 -> [w3104]
                  tunnel: [w3103] -> w3074
                  tunnel: w3073 -> [w3103]
                  tunnel: w3066 -> [w3102]
                  tunnel: w3076 -> [w3108]
                  tunnel: w3074 -> [w3107]
                  tunnel: [w3106] -> w3071
                  tunnel: [w3105] -> w3068
                  tunnel: [w3115] -> w3072
                  tunnel: w3071 -> [w3115]
                  tunnel: [w3114] -> w3069
                  tunnel: w3068 -> [w3114]
                  tunnel: w3065 -> [w3113]
                  tunnel: w3072 -> [w3118]
                  tunnel: [w3117] -> w3070
                  tunnel: w3069 -> [w3116]
                  frame #0 {
                    n1223 = Bundle(cluster=T5 {"Message"="", "Message Data"=variant} ("Message Cluster"), "Message"="FGGA_pump", "Message Data"=FALSE) -> (w3087:T5)
                    n1224 = Enqueue Element(queue=w3086, element=w3087, error in (no error)=w3085) -> (queue out=w3083:refnum<queue>, error out=w3084:errorcluster)  [unwired: 1 in, 1 out]
                  }
                  frame #1 {
                    n1225 = Wait (ms)(milliseconds to wait=w3091) -> ()  [unwired: 1 out]
                  }
                  frame #2 {
                    w3101 = FALSE
                    n1226 = local write "eV11"(w3101) -> ()
                    n1227 = Bundle(cluster=T5 {"Message"="", "Message Data"=variant} ("Message Cluster"), "Message"="V11" ("Message 2"), "Message Data"=w3101) -> (w3100:T5)
                    n1228 = Enqueue Element(queue=w3096, element=w3100, error in (no error)=w3097) -> (queue out=w3095:refnum<queue>, error out=w3094:errorcluster)  [unwired: 1 in, 1 out]
                  }
                  frame #3 {
                    n1229 = Wait (ms)(milliseconds to wait=w3102) -> ()  [unwired: 1 out]
                  }
                  frame #4 {
                    w3112 = TRUE
                    n1230 = local write "eV12"(w3112) -> ()
                    n1231 = Bundle(cluster=T5 {"Message"="", "Message Data"=variant} ("Message Cluster"), "Message"="V12" ("Message 2"), "Message Data"=w3112) -> (w3110:T5)
                    n1232 = Enqueue Element(queue=w3108, element=w3110, error in (no error)=w3107) -> (queue out=w3105:refnum<queue>, error out=w3106:errorcluster)  [unwired: 1 in, 1 out]
                  }
                  frame #5 {
                    n1233 = Wait (ms)(milliseconds to wait=w3113) -> ()  [unwired: 1 out]
                  }
                  frame #6 {
                    w3119 = TRUE
                    n1234 = Bundle(cluster=T5 {"Message"="", "Message Data"=variant} ("Message Cluster"), "Message"="V10", "Message Data"=w3119) -> (w3122:T5)
                    n1235 = local write "eV10"(w3119) -> ()
                    n1236 = Enqueue Element(queue=w3116, element=w3122, error in (no error)=w3118) -> (error out=w3117:errorcluster)  [unwired: 1 in, 2 out]
                  }
                }
              }
            }
          }
          frame #9 {
            w3123 = FALSE ("High Cal")
            n1237 = local write "Target Cal\n140 Torr"(w3123) -> ()
            n1238 = local write "FGGA 140 Torr\nCalibration Abort"(w3123) -> ()
          }
        }
      }
      event "MFC_1\nSLPM Value": Value Change {
        n1239 = event-data() -> ()  [unwired: 1 in, 1 out]
        n1240 = local read "MFC_1\nSLPM Value"() -> (w3125:dbl)
        n1241 = Bundle(cluster=T5 {"Message"="", "Message Data"=variant} ("Message Cluster"), "Message"="MFC_1", "Message Data"=w3125) -> (w3129:T5)
        n1242 = Enqueue Element(queue=w3128, element=w3129, error in (no error)=w3127) -> (error out=w3126:errorcluster)  [unwired: 1 in, 2 out]
      }
      event "FGGA UDP Time Offset": Value Change {
        n1243 = event-data() -> ("NewVal"=w3132:i32)  [unwired: 1 in, 5 out]
        n1244 = Bundle(cluster=T5 {"Message"="", "Message Data"=variant} ("Message Cluster"), "Message"="UDP Time Offset", "Message Data"=w3132) -> (w3136:T5)
        n1245 = Enqueue Element(queue=w3135, element=w3136, error in (no error)=w3134) -> (error out=w3133:errorcluster)  [unwired: 1 in, 2 out]
      }
    }
    "FGGA Event Error out" <- w806
  }
  n1246 = node-c288(w25) -> ()  [unwired: 1 out]
  n1247 = Obtain Queue(name (unnamed)="FGGA_Scroll_Pump_Command", element data type=w3) -> (queue out=w2:refnum<queue>, error out=w1:errorcluster)  [unwired: 3 in, 1 out]
  n1248 = Create Network Stream Writer Endpoint(6:w8, 7:10 ("writer buffer size"), 9:w3, 10:"//192.168.101.17/command/reader/FGGA_Scroll_Pump" ("reader url"), 11:"/command/writer/FGGA_Scroll_Pump" ("writer name")) -> (0:w7:errorcluster, 3:w6:refnum<k21>)  [unwired: 2 in]
  n1249 = while {
    tunnel: w2 -> [w3141]
    tunnel: w1 -> [w3140]
    stop <- FALSE stop-if-true
    # "FGGA Scroll Pump Event Loop"
    n1250 = event shown="[0] \"Use Standby Speed\": Value Change" {
      selector: _ -> [_ _ _ _ _]
      dyn-events: _ -> [_ _ _ _ _]
      timeout: _ -> [_ _ _ _ _]
      tunnel: w3141 -> [w3145 w3151 w3157 w3163 w3169]
      tunnel: w3140 -> [w3144 w3150 w3156 w3162 w3168]
      event "Use Standby Speed": Value Change {
        n1251 = event-data() -> ("NewVal"=w3142:bool)  [unwired: 1 in, 5 out]
        n1252 = Bundle(cluster=T5 {"Message"="", "Message Data"=variant} ("Message Cluster"), "Message"="Use_Standby_Speed", "Message Data"=w3142) -> (w3146:T5)
        n1253 = Enqueue Element(queue=w3145, element=w3146, error in (no error)=w3144) -> ()  [unwired: 1 in, 3 out]
      }
      event "Normal Speed Threshold": Value Change {
        n1254 = event-data() -> ("NewVal"=w3148:u32)  [unwired: 1 in, 5 out]
        n1255 = Bundle(cluster=T5 {"Message"="", "Message Data"=variant} ("Message Cluster"), "Message"="Normal_Speed_Threshold", "Message Data"=w3148) -> (w3152:T5)
        n1256 = Enqueue Element(queue=w3151, element=w3152, error in (no error)=w3150) -> ()  [unwired: 1 in, 3 out]
      }
      event "Scroll Pump On/Off": Value Change {
        n1257 = event-data() -> ("NewVal"=w3154:bool)  [unwired: 1 in, 5 out]
        n1258 = Bundle(cluster=T5 {"Message"="", "Message Data"=variant} ("Message Cluster"), "Message"="Scroll_Pump_On_Off", "Message Data"=w3154) -> (w3158:T5)
        n1259 = Enqueue Element(queue=w3157, element=w3158, error in (no error)=w3156) -> ()  [unwired: 1 in, 3 out]
      }
      event "Standby Speed\n66% - 100%": Value Change {
        n1260 = event-data() -> ("NewVal"=w3160:u32)  [unwired: 1 in, 5 out]
        n1261 = Bundle(cluster=T5 {"Message"="", "Message Data"=variant} ("Message Cluster"), "Message"="Standby_Speed_Threshold", "Message Data"=w3160) -> (w3164:T5)
        n1262 = Enqueue Element(queue=w3163, element=w3164, error in (no error)=w3162) -> ()  [unwired: 1 in, 3 out]
      }
      event "Standby Speed %\nDefault Set Value": Value Change {
        n1263 = event-data() -> ("NewVal"=w3166:u32)  [unwired: 1 in, 5 out]
        n1264 = Bundle(cluster=T5 {"Message"="", "Message Data"=variant} ("Message Cluster"), "Message"="Standby_Speed_Default", "Message Data"=w3166) -> (w3170:T5)
        n1265 = Enqueue Element(queue=w3169, element=w3170, error in (no error)=w3168) -> ()  [unwired: 1 in, 3 out]
      }
    }
  }
  n1266 = while {
    tunnel: w2 -> [w3179]
    shift-right: [w3174] -> _
    shift-left: w6 -> [w3176]
    shift-right: [w3172] -> w4
    shift-left: w7 -> [w3178]
    tunnel: w1 -> [w3173]
    stop <- w3172 stop-if-true
    # "FGGA UI Command Sender"
    n1267 = Dequeue Element(queue=w3179, error in (no error)=w3173) -> (element=w3175:T5)  [unwired: 1 in, 3 out]
    n1268 = Unbundle By Name(w3175) -> ("Message"=w3177:string)
    n1269 = case shown="\"Normal_Speed_Threshold\"" w3177 {
      tunnel: w3178 -> [w3180 w3184 w3191 w3198 w3205 w3212]
      tunnel: w3176 -> [w3181 w3187 w3194 w3201 w3208 w3215]
      tunnel: w3175 -> [_ w3186 w3193 w3200 w3207 w3214]
      tunnel: [w3180 w3183 w3190 w3197 w3204 w3211] -> w3172
      tunnel: [w3181 w3182 w3189 w3196 w3203 w3210] -> w3174
      frame "False", Default {
      }
      frame "Use_Standby_Speed" {
        n1270 = shared-variable-write(w3187, w3184, w3186) -> (w3185:refnum<k21>, w3188:errorcluster)  [unwired: 1 in, 1 out]
        n1271 = Flush Stream(8:w3188, 11:w3185) -> (0:w3183:errorcluster, 3:w3182:refnum<k21>)  [unwired: 2 in, 1 out]
      }
      frame "Standby_Speed_Threshold" {
        n1272 = shared-variable-write(w3194, w3191, w3193) -> (w3192:refnum<k21>, w3195:errorcluster)  [unwired: 1 in, 1 out]
        n1273 = Flush Stream(8:w3195, 11:w3192) -> (0:w3190:errorcluster, 3:w3189:refnum<k21>)  [unwired: 2 in, 1 out]
      }
      frame "Normal_Speed_Threshold" {
        n1274 = shared-variable-write(w3201, w3198, w3200) -> (w3199:refnum<k21>, w3202:errorcluster)  [unwired: 1 in, 1 out]
        n1275 = Flush Stream(8:w3202, 11:w3199) -> (0:w3197:errorcluster, 3:w3196:refnum<k21>)  [unwired: 2 in, 1 out]
      }
      frame "Standby_Speed_Default" {
        n1276 = shared-variable-write(w3208, w3205, w3207) -> (w3206:refnum<k21>, w3209:errorcluster)  [unwired: 1 in, 1 out]
        n1277 = Flush Stream(8:w3209, 11:w3206) -> (0:w3204:errorcluster, 3:w3203:refnum<k21>)  [unwired: 2 in, 1 out]
      }
      frame "Scroll_Pump_On_Off" {
        n1278 = shared-variable-write(w3215, w3212, w3214) -> (w3213:refnum<k21>, w3216:errorcluster)  [unwired: 1 in, 1 out]
        n1279 = Flush Stream(8:w3216, 11:w3213) -> (0:w3211:errorcluster, 3:w3210:refnum<k21>)  [unwired: 2 in, 1 out]
      }
    }
  }
  "FGGA Scroll Pump\ncommand sender error out" <- w4
  n1280 = Create Network Stream Writer Endpoint(6:w65, 7:10 ("writer buffer size"), 9:w67, 10:"//192.168.101.17/command/reader/FGGA" ("reader url"), 11:"/command/writer/FGGA" ("writer name")) -> (0:w64:errorcluster, 3:w63:refnum<k21>)  [unwired: 2 in]
  n1281 = while {
    tunnel: w17 -> [w3224]
    shift-right: [w3219] -> _
    shift-left: w63 -> [w3221]
    shift-right: [w3217] -> w60
    shift-left: w64 -> [w3223]
    tunnel: w16 -> [w3218]
    stop <- w3217 stop-if-true
    # "FGGA UI Command Sender"
    n1282 = Dequeue Element(queue=w3224, error in (no error)=w3218) -> (element=w3220:T5)  [unwired: 1 in, 3 out]
    n1283 = Unbundle By Name(w3220) -> ("Message"=w3222:string)
    n1284 = case shown="\"High_Flow\"" w3222 {
      tunnel: w3223 -> [w3225 w3229 w3236 w3243 w3250 w3257 w3264 w3271 w3278 w3285 w3292 w3299 w3306 w3313 w3320 w3327 w3334]
      tunnel: w3221 -> [w3226 w3232 w3239 w3246 w3253 w3260 w3267 w3274 w3281 w3288 w3295 w3302 w3309 w3316 w3323 w3330 w3337]
      tunnel: w3220 -> [_ w3231 w3238 w3245 w3252 w3259 w3266 w3273 w3280 w3287 w3294 w3301 w3308 w3315 w3322 w3329 w3336]
      tunnel: [w3225 w3228 w3235 w3242 w3249 w3256 w3263 w3270 w3277 w3284 w3291 w3298 w3305 w3312 w3319 w3326 w3333] -> w3217
      tunnel: [w3226 w3227 w3234 w3241 w3248 w3255 w3262 w3269 w3276 w3283 w3290 w3297 w3304 w3311 w3318 w3325 w3332] -> w3219
      frame "False", Default {
      }
      frame "V1" {
        n1285 = shared-variable-write(w3232, w3229, w3231) -> (w3230:refnum<k21>, w3233:errorcluster)  [unwired: 1 in, 1 out]
        n1286 = Flush Stream(8:w3233, 11:w3230) -> (0:w3228:errorcluster, 3:w3227:refnum<k21>)  [unwired: 2 in, 1 out]
      }
      frame "MFC_1" {
        n1287 = shared-variable-write(w3239, w3236, w3238) -> (w3237:refnum<k21>, w3240:errorcluster)  [unwired: 1 in, 1 out]
        n1288 = Flush Stream(8:w3240, 11:w3237) -> (0:w3235:errorcluster, 3:w3234:refnum<k21>)  [unwired: 2 in, 1 out]
      }
      frame "UDP Time Offset" {
        n1289 = shared-variable-write(w3246, w3243, w3245) -> (w3244:refnum<k21>, w3247:errorcluster)  [unwired: 1 in, 1 out]
        n1290 = Flush Stream(8:w3247, 11:w3244) -> (0:w3242:errorcluster, 3:w3241:refnum<k21>)  [unwired: 2 in, 1 out]
      }
      frame "V2" {
        n1291 = shared-variable-write(w3253, w3250, w3252) -> (w3251:refnum<k21>, w3254:errorcluster)  [unwired: 1 in, 1 out]
        n1292 = Flush Stream(8:w3254, 11:w3251) -> (0:w3249:errorcluster, 3:w3248:refnum<k21>)  [unwired: 2 in, 1 out]
      }
      frame "V3" {
        n1293 = shared-variable-write(w3260, w3257, w3259) -> (w3258:refnum<k21>, w3261:errorcluster)  [unwired: 1 in, 1 out]
        n1294 = Flush Stream(8:w3261, 11:w3258) -> (0:w3256:errorcluster, 3:w3255:refnum<k21>)  [unwired: 2 in, 1 out]
      }
      frame "V4" {
        n1295 = shared-variable-write(w3267, w3264, w3266) -> (w3265:refnum<k21>, w3268:errorcluster)  [unwired: 1 in, 1 out]
        n1296 = Flush Stream(8:w3268, 11:w3265) -> (0:w3263:errorcluster, 3:w3262:refnum<k21>)  [unwired: 2 in, 1 out]
      }
      frame "V10" {
        n1297 = shared-variable-write(w3274, w3271, w3273) -> (w3272:refnum<k21>, w3275:errorcluster)  [unwired: 1 in, 1 out]
        n1298 = Flush Stream(8:w3275, 11:w3272) -> (0:w3270:errorcluster, 3:w3269:refnum<k21>)  [unwired: 2 in, 1 out]
      }
      frame "V11" {
        n1299 = shared-variable-write(w3281, w3278, w3280) -> (w3279:refnum<k21>, w3282:errorcluster)  [unwired: 1 in, 1 out]
        n1300 = Flush Stream(8:w3282, 11:w3279) -> (0:w3277:errorcluster, 3:w3276:refnum<k21>)  [unwired: 2 in, 1 out]
      }
      frame "V12" {
        n1301 = shared-variable-write(w3288, w3285, w3287) -> (w3286:refnum<k21>, w3289:errorcluster)  [unwired: 1 in, 1 out]
        n1302 = Flush Stream(8:w3289, 11:w3286) -> (0:w3284:errorcluster, 3:w3283:refnum<k21>)  [unwired: 2 in, 1 out]
      }
      frame "Low_Flow" {
        n1303 = shared-variable-write(w3295, w3292, w3294) -> (w3293:refnum<k21>, w3296:errorcluster)  [unwired: 1 in, 1 out]
        n1304 = Flush Stream(8:w3296, 11:w3293) -> (0:w3291:errorcluster, 3:w3290:refnum<k21>)  [unwired: 2 in, 1 out]
      }
      frame "No_Flow" {
        n1305 = shared-variable-write(w3302, w3299, w3301) -> (w3300:refnum<k21>, w3303:errorcluster)  [unwired: 1 in, 1 out]
        n1306 = Flush Stream(8:w3303, 11:w3300) -> (0:w3298:errorcluster, 3:w3297:refnum<k21>)  [unwired: 2 in, 1 out]
      }
      frame "High_Flow" {
        n1307 = shared-variable-write(w3309, w3306, w3308) -> (w3307:refnum<k21>, w3310:errorcluster)  [unwired: 1 in, 1 out]
        n1308 = Flush Stream(8:w3310, 11:w3307) -> (0:w3305:errorcluster, 3:w3304:refnum<k21>)  [unwired: 2 in, 1 out]
      }
      frame "FGGA_pump" {
        n1309 = shared-variable-write(w3316, w3313, w3315) -> (w3314:refnum<k21>, w3317:errorcluster)  [unwired: 1 in, 1 out]
        n1310 = Flush Stream(8:w3317, 11:w3314) -> (0:w3312:errorcluster, 3:w3311:refnum<k21>)  [unwired: 2 in, 1 out]
      }
      frame "Flight Number" {
        n1311 = shared-variable-write(w3323, w3320, w3322) -> (w3321:refnum<k21>, w3324:errorcluster)  [unwired: 1 in, 1 out]
        n1312 = Flush Stream(8:w3324, 11:w3321) -> (0:w3319:errorcluster, 3:w3318:refnum<k21>)  [unwired: 2 in, 1 out]
      }
      frame "FGGA_restart" {
        n1313 = shared-variable-write(w3330, w3327, w3329) -> (w3328:refnum<k21>, w3331:errorcluster)  [unwired: 1 in, 1 out]
        n1314 = Flush Stream(8:w3331, 11:w3328) -> (0:w3326:errorcluster, 3:w3325:refnum<k21>)  [unwired: 2 in, 1 out]
      }
      frame "Stop File Write" {
        n1315 = shared-variable-write(w3337, w3334, w3336) -> (w3335:refnum<k21>, w3338:errorcluster)  [unwired: 1 in, 1 out]
        n1316 = Flush Stream(8:w3338, 11:w3335) -> (0:w3333:errorcluster, 3:w3332:refnum<k21>)  [unwired: 2 in, 1 out]
      }
    }
  }
  "FGGA command sender error out" <- w60
  n1317 = while {
    stop <- FALSE stop-if-true
    # "Auto restart communication to the pump server"
    n1318 = TCP Open Connection(address="Target IP Address", remote port or service name=u16 8001 ("remote port")) -> (connection ID=w3353:refnum<k5>, error out=w3352:errorcluster)  [unwired: 1 in, 2 out]
    n1319 = call-poly <vilib>:"Read Meta Data.vi"("error in"=w3352, "connection ID"=w3353) -> ("error out"=w3348:errorcluster, "connection info out"=w3349:T15)  [unwired: 1 in, 7 out]
    n1320 = node-c288() -> (w3355:T6)  [unwired: 4 in]
    n1321 = timed-loop {
      timing: w3355 -> [_]
      timing-out: [_] -> w3354
      tunnel: w3349 -> [w3376]
      tunnel: w3348 -> [w3379]
      tunnel: [w3384] -> w3346
      tunnel: [w3373] -> w3345
      shift-right: [w3362] -> _
      shift-left: "Standby Speed %\nDefault Set Value" -> [w3363]
      i -> [w3372]
      stop <- w3373 stop-if-true
      # "Receive Scroll pump data from cRIO"
      n1322 = node-c288() -> ()  [unwired: 1 in, 1 out]
      n1323 = call-poly <vilib>:"Read Message.vi"("error in"=w3379, "connection info in"=w3376) -> ("error out"=w3378:errorcluster, "data string"=w3375:string, "connection info out"=w3377:T15)  [unwired: 1 in, 6 out]
      n1324 = Unflatten From String(type=0, binary string=w3375) -> (value=w3367:i32, error out=w3371:errorcluster)  [unwired: 1 in, 3 out]
      n1325 = for {
        N: w3367 -> [_]
        shift-right: [w3477] -> w3384
        shift-left: w3377 -> [w3479]
        shift-right: [w3476] -> w3373
        shift-left: w3378 -> [w3478]
        tunnel: [w3475] -> _ mode=indexing
        tunnel: [w3472] -> w3383 mode=indexing
        tunnel: [w3471] -> w3380 mode=indexing
        n1326 = call-poly <vilib>:"Read Message.vi"("error in"=w3478, "connection info in"=w3479) -> ("error out"=w3476:errorcluster, "data string"=w3473:string, "connection info out"=w3477:T15, "data info"=w3475:T17)  [unwired: 1 in, 5 out]
        n1327 = Unflatten From String(type="", binary string=w3473) -> (value=w3472:string, error out=w3471:errorcluster)  [unwired: 1 in, 3 out]
      }
      "FGGA Scroll Pump Monitoring" <- w3383
      "Scroll Pump Read Error" <- w3380
      n1328 = case shown="Error" w3371 {
        selector: w3371 -> [w3467 w3468]
        tunnel: [w3467 w3468] -> w3358
        frame No Error {
        }
        frame Error {
          n1329 = property on="Scroll Pump \nat Fault" class="Bool (strict)"("Blinking"=TRUE) -> ()  [unwired: 2 in, 2 out]
          "Scroll Pump not running" <- "Pump NOT fitted or Pump power is OFF" ("message")
        }
      }
      n1330 = Index Array(array=w3383) -> (element #1=w3370:string, element #2=w3382:string, element #3=w3381:string, element #4=w3361:string, element #5=w3360:string)  [unwired: 5 in]
      n1331 = Equal?(x=w3367, y=1) -> (x = y?=w3366:bool)
      n1332 = Equal?(x=w3370, y="Read Error") -> (x = y?=w3365:bool)
      n1333 = Or(x=w3366, y=w3365) -> (x .or. y?=w3364:bool)
      n1334 = case shown="False" w3364 {
        tunnel: w3370 -> [w3411 _]
        tunnel: w3382 -> [w3410 _]
        tunnel: w3381 -> [w3409 _]
        tunnel: w3372 -> [w3408 _]
        tunnel: w3363 -> [w3407 w3466]
        tunnel: [w3406 w3466] -> w3362
        tunnel: w3361 -> [w3394 _]
        tunnel: w3360 -> [w3393 _]
        tunnel: [w3386 FALSE] -> w3359
        frame False {
          n1335 = local read "Standby Speed %\nDefault Set Value"() -> (w3406:u32)
          n1336 = Match Pattern(string=w3411, regular expression="=V802") -> (after substring=w3412:string)  [unwired: 1 in, 3 out]
          n1337 = Match Pattern(string=w3410, regular expression="=V808") -> (after substring=w3452:string)  [unwired: 1 in, 3 out]
          n1338 = Match Pattern(string=w3409, regular expression="=V809") -> (after substring=w3443:string)  [unwired: 1 in, 3 out]
          n1339 = Match Pattern(string=w3393, regular expression="=S805") -> (after substring=w3402:string)  [unwired: 1 in, 3 out]
          n1340 = Match Pattern(string=w3394, regular expression="=S804") -> (after substring=w3403:string)  [unwired: 1 in, 3 out]
          n1341 = Equal To 0?(x=w3408) -> (x = 0?=w3398:bool)
          n1342 = Equal?(x=w3408, y=1) -> (x = y?=w3399:bool)
          n1343 = Not Equal?(x=w3407, y=w3406) -> (x != y?=w3395:bool)
          n1344 = Spreadsheet String To Array(delimiter (Tab)=";", format string="%s", spreadsheet string=w3412, array type (2D Dbl)=string[] []) -> (array=w3424:string[])
          n1345 = String Subset(string=w3452) -> (substring=w3454:string)  [unwired: 2 in]
          n1346 = String Subset(string=w3443) -> (substring=w3445:string)  [unwired: 2 in]
          n1347 = Decimal String To Number(string=w3402) -> (number=w3401:i32)  [unwired: 2 in, 1 out]
          n1348 = Decimal String To Number(string=w3403) -> (number=w3400:i32)  [unwired: 2 in, 1 out]
          n1349 = Compound Arithmetic op=OR(w3398, w3399, w3395) -> (w3397:bool)
          n1350 = Index Array(array=w3424, index=0) -> (element=w3422:string)
          n1351 = Array Subset(array=w3424, index=1) -> (w3425:string[])  [unwired: 1 in]
          n1352 = case shown="True" w3397 {
            tunnel: w3401 -> [_ w3459]
            tunnel: w3400 -> [_ w3460]
            frame False {
            }
            frame True {
              n1353 = local write "Normal Speed Threshold"(w3460) -> ()
              n1354 = local write "Standby Speed\n66% - 100%"(w3459) -> ()
            }
          }
          n1355 = Spreadsheet String To Array(delimiter (Tab)=";", format string="%s", spreadsheet string=w3454, array type (2D Dbl)=string[] []) -> (array=w3451:string[])
          n1356 = Spreadsheet String To Array(delimiter (Tab)=";", format string="%s", spreadsheet string=w3445, array type (2D Dbl)=string[] []) -> (array=w3442:string[])
          n1357 = Decimal String To Number(string=w3422) -> (number=→"Motor Frequency":i32)  [unwired: 2 in, 1 out]
          n1358 = for {
            tunnel: w3425 -> [w3464] mode=indexing
            tunnel: [w3461] -> w3414 mode=indexing
            n1359 = Hexadecimal String To Number(string=w3464, default (0uL)=u16 0 ("default (0 U32)")) -> (number=w3462:u16)  [unwired: 1 in, 1 out]
            n1360 = Number To Boolean Array(number=w3462) -> (Boolean array=w3461:bool[])
          }
          n1361 = Index Array(array=w3451) -> (element #2=w3450:string)  [unwired: 2 in, 1 out]
          n1362 = Index Array(array=w3442) -> (element #1=w3441:string, element #2=w3440:string, element #3=w3439:string)  [unwired: 3 in]
          n1363 = Decimal String To Number(string=w3450) -> (number=→"Pump Controller Temperature":i32)  [unwired: 2 in, 1 out]
          n1364 = Decimal String To Number(string=w3441) -> (number=w3438:i32)  [unwired: 2 in, 1 out]
          n1365 = Decimal String To Number(string=w3440) -> (number=w3434:i32)  [unwired: 2 in, 1 out]
          n1366 = Decimal String To Number(string=w3439) -> (number=w3431:i32)  [unwired: 2 in, 1 out]
          n1367 = Divide(x=w3438, y=10) -> (x/y=→"Measured Link Voltage (V)":dbl)
          n1368 = Divide(x=w3434, y=10) -> (x/y=→"Measured Motor Current (A)":dbl)
          n1369 = Divide(x=w3431, y=10) -> (x/y=→"Measured Motor Power (W)":dbl)
          n1370 = Index Array(array=w3414, index (row)=3) -> (element=→"Fault register":bool[])  [unwired: 1 in]
          n1371 = Index Array(array=w3414, index (row)=2) -> (element=→"Warning register":bool[])  [unwired: 1 in]
          n1372 = Index Array(array=w3414, index (row)=0) -> (element=→"System status register":bool[])  [unwired: 1 in]
          n1373 = Index Array(array=w3414, index (row)=1) -> (element=w3390:bool[])  [unwired: 1 in]
          "System status register 2" <- w3390
          n1374 = Index Array(array=w3390, index #1=6 ("index")) -> (element #1=w3389:bool, element #2=w3388:bool)  [unwired: 1 in]
          n1375 = Or(x=w3389, y=w3388) -> (x .or. y?=w3387:bool)
          n1376 = Not(x=w3387) -> (.not. x?=w3386:bool)
          n1377 = case shown="True" w3387 {
            selector: w3387 -> [_ w3458]
            frame False {
            }
            frame True {
              n1378 = property on="Scroll Pump \nat Fault" class="Bool (strict)"("Blinking"=w3458) -> ()  [unwired: 2 in, 2 out]
            }
          }
        }
        frame True {
        }
      }
      n1379 = Not(x=w3358) -> (.not. x?=w3356:bool)
      n1380 = Compound Arithmetic op=AND(w3356, w3359) -> (w3357:bool)
      n1381 = case shown="True" w3357 {
        frame False {
        }
        frame True {
          n1382 = property on="Scroll Pump \nat Fault" class="Bool (strict)"("Blinking"=FALSE) -> ()  [unwired: 2 in, 2 out]
        }
      }
      n1383 = node-c288() -> ()  [unwired: 1 in, 1 out]
      "Receiver Loop Count" <- w3372
    }
    n1384 = node-c288(w3354) -> ()  [unwired: 1 out]
    n1385 = call-poly <vilib>:"Get Connection Reference.vi"("error in"=w3345, "connection info in"=w3346) -> ("error out"=w3347:errorcluster, "connection ID out"=w3344:refnum<k5>)  [unwired: 8 out]
    n1386 = TCP Close Connection(connection ID=w3344, error in (no error)=w3347) -> (error out=→"Network error out":errorcluster)  [unwired: 2 out]
    n1387 = Wait (ms)(milliseconds to wait=u32 1000) -> ()  [unwired: 1 out]
    "Scroll Pump \nat Fault" <- FALSE ("Scroll Pump \nat Fault")
  }
  n1388 = while {
    stop <- FALSE stop-if-true
    # "Scroll Pump Fault Descriptions"
    n1389 = Wait (ms)(milliseconds to wait=u32 500) -> ()  [unwired: 1 out]
    n1390 = case shown="True" "Scroll Pump Faults" {
      frame False {
      }
      frame True {
        n1391 = local read "Warning register"() -> (w3489:bool[])
        n1392 = local read "Scroll Pump not running"() -> (w3487:string)
        n1393 = local read "Fault register"() -> (w3488:bool[])
        n1394 = call "Scroll_Pump_Error_Message.vi"("Scroll Pump Message"=w3487, "Fault register"=w3488, "Warning register"=w3489) -> ()  [unwired: 9 in]
      }
    }
  }
  n1395 = local write "FGGA Calibration Abort"(FALSE ("FGGA Calibration Abort")) -> ()
  n1396 = Obtain Queue(name (unnamed)="SO2_Command", element data type=w51) -> (queue out=w15:refnum<queue>, error out=w14:errorcluster)  [unwired: 3 in, 1 out]
  n1397 = while {
    tunnel: w15 -> [w3493]
    tunnel: w14 -> [w3492]
    tunnel: [w3490] -> _
    stop <- FALSE stop-if-true
    # "SO2 UI Event Handler Loop"
    n1398 = event shown="[7] \"SO2 Zero Calibration\": Value Change" {
      selector: _ -> [_ _ _ _ _ _ _ _ _ _ _ _ _ _ _ _ _ _ _ _ _ _ _ _ _ _ _ _ _ _]
      dyn-events: _ -> [_ _ _ _ _ _ _ _ _ _ _ _ _ _ _ _ _ _ _ _ _ _ _ _ _ _ _ _ _ _]
      timeout: _ -> [_ _ _ _ _ _ _ _ _ _ _ _ _ _ _ _ _ _ _ _ _ _ _ _ _ _ _ _ _ _]
      tunnel: w3493 -> [w3500 w3512 w3559 w3570 w3613 w3648 w3759 w3907 w4033 w4039 w4050 w4053 w4061 w4067 w4074 w4080 w4086 w4096 w4100 w4107 w4114 w4121 w4128 w4135 w4142 w4149 w4156 w4163 w4171 w4185]
      tunnel: w3492 -> [w3499 w3511 w3558 w3569 w3612 w3647 w3758 w3906 w4032 w4038 w4049 w4052 w4059 w4066 w4073 w4079 w4085 w4095 w4099 w4106 w4113 w4120 w4127 w4134 w4141 w4148 w4155 w4162 w4170 w4184]
      tunnel: [w3494 w3510 _ w3568 w3611 _ _ _ _ _ w4044 w4051 w4058 _ w4072 _ _ w4090 w4098 w4105 w4112 w4119 w4126 w4133 w4140 w4147 w4154 w4161 w4169 w4183] -> w3490
      event "eV9": Value Change {
        n1399 = event-data() -> ("NewVal"=w3497:bool)  [unwired: 1 in]
        n1400 = Bundle(cluster=T5 {"Message"="", "Message Data"=variant} ("Message Cluster"), "Message"="V9", "Message Data"=w3497) -> (w3495:T5)
        n1401 = Enqueue Element(queue=w3500, element=w3495, error in (no error)=w3499) -> (error out=w3494:errorcluster)  [unwired: 1 in, 2 out]
      }
      event "SO2 Flush": Value Change {
        n1402 = event-data() -> ()  [unwired: 1 in, 1 out]
        n1403 = flat-sequence {
          tunnel: w3512 -> [w3520]
          tunnel: w3511 -> [w3519]
          tunnel: [w3515] -> w3507
          tunnel: [w3513] -> w3505
          tunnel: w3507 -> [w3522]
          tunnel: [w3524] -> w3506
          tunnel: w3505 -> [w3523]
          tunnel: [w3525] -> w3504
          tunnel: w3506 -> [w3531]
          tunnel: [w3531] -> w3509
          tunnel: [w3529] -> w3508
          tunnel: w3504 -> [w3529]
          tunnel: w3509 -> [w3543]
          tunnel: [w3542] -> w3503
          tunnel: w3508 -> [w3544]
          tunnel: [w3540] -> w3501
          tunnel: w3503 -> [w3550]
          tunnel: [w3551] -> w3502
          tunnel: w3501 -> [w3549]
          tunnel: [w3556] -> w3510
          tunnel: w3502 -> [w3556]
          frame #0 {
            w3514 = TRUE ("SO2 Flush")
            n1404 = Bundle(cluster=T5 {"Message"="", "Message Data"=variant} ("Message Cluster"), "Message"="V9", "Message Data"=w3514) -> (w3516:T5)
            n1405 = local write "eV9"(w3514) -> ()
            n1406 = Enqueue Element(queue=w3520, element=w3516, error in (no error)=w3519) -> (queue out=w3513:refnum<queue>, error out=w3515:errorcluster)  [unwired: 1 in, 1 out]
          }
          frame #1 {
            n1407 = local read "MFC_2 User Set Value"() -> (w3521:dbl)
            n1408 = local write "MFC_2\nSLPM Value"(w3521) -> ()
            n1409 = Bundle(cluster=T5 {"Message"="", "Message Data"=variant} ("Message Cluster"), "Message"="MFC_2", "Message Data"=w3521) -> (w3526:T5)
            n1410 = Enqueue Element(queue=w3523, element=w3526, error in (no error)=w3522) -> (queue out=w3525:refnum<queue>, error out=w3524:errorcluster)  [unwired: 1 in, 1 out]
          }
          frame #2 {
            n1411 = for {
              N: "eV9 Flush User\nset time (sec)" -> [w3538]
              i -> [w3537]
              stop <- w3532 stop-if-true
              n1412 = local read "Network disconnected"() -> (w3532:bool)
              n1413 = Subtract(x=w3538, y=w3537) -> (x-y=w3536:i32)
              n1414 = Decrement(x=w3536) -> (x-1=w3534:i32)
              n1415 = Wait (ms)(milliseconds to wait=u32 1000) -> ()  [unwired: 1 out]
              n1416 = Select(t=0, s=w3532, f=w3534) -> (s? t:f=w3533:i32)
              n1417 = local write "SO2 Flush\nTime Remain (sec)"(w3533) -> ()
            }
          }
          frame #3 {
            w3541 = FALSE
            n1418 = Bundle(cluster=T5 {"Message"="", "Message Data"=variant} ("Message Cluster"), "Message"="V9", "Message Data"=w3541) -> (w3545:T5)
            n1419 = local write "eV9"(w3541) -> ()
            n1420 = Enqueue Element(queue=w3544, element=w3545, error in (no error)=w3543) -> (queue out=w3540:refnum<queue>, error out=w3542:errorcluster)  [unwired: 1 in, 1 out]
          }
          frame #4 {
            w3548 = 0.0 ("MFC_2\nSLPM Value")
            n1421 = local write "MFC_2\nSLPM Value"(w3548) -> ()
            n1422 = Bundle(cluster=T5 {"Message"="", "Message Data"=variant} ("Message Cluster"), "Message"="MFC_2", "Message Data"=w3548) -> (w3552:T5)
            n1423 = Enqueue Element(queue=w3549, element=w3552, error in (no error)=w3550) -> (error out=w3551:errorcluster)  [unwired: 1 in, 2 out]
          }
          frame #5 {
            n1424 = local write "SO2 Flush"(FALSE ("SO2 Flush")) -> ()
          }
        }
      }
      event "Auto Zeroing \ninterval (sec)": Value Change {
        n1425 = event-data() -> ("NewVal"=w3557:i32)  [unwired: 1 in]
        n1426 = Bundle(cluster=T5 {"Message"="", "Message Data"=variant} ("Message Cluster"), "Message"="zeroing_interval", "Message Data"=w3557) -> (w3560:T5)
        n1427 = Enqueue Element(queue=w3559, element=w3560, error in (no error)=w3558) -> ()  [unwired: 1 in, 3 out]
      }
      event "SO2 GND Zeroing": Value Change {
        n1428 = event-data() -> ()  [unwired: 1 in, 1 out]
        n1429 = flat-sequence {
          tunnel: w3570 -> [w3578]
          tunnel: w3569 -> [w3577]
          tunnel: [w3573] -> w3567
          tunnel: [w3571] -> w3563
          tunnel: w3567 -> [w3581]
          tunnel: [w3581] -> w3566
          tunnel: [w3580] -> w3564
          tunnel: w3563 -> [w3580]
          tunnel: w3566 -> [w3599]
          tunnel: [w3598] -> w3565
          tunnel: w3564 -> [w3600]
          tunnel: [w3605] -> w3568
          tunnel: w3565 -> [w3605]
          frame #0 {
            w3572 = TRUE ("SO2 Flush")
            n1430 = local write "SO2 eV6"(w3572) -> ()
            n1431 = Bundle(cluster=T5 {"Message"="", "Message Data"=variant} ("Message Cluster"), "Message"="V6", "Message Data"=w3572) -> (w3574:T5)
            n1432 = Enqueue Element(queue=w3578, element=w3574, error in (no error)=w3577) -> (queue out=w3571:refnum<queue>, error out=w3573:errorcluster)  [unwired: 1 in, 1 out]
          }
          frame #1 {
            # "10 Mins Count down"
            n1433 = for {
              N: "eV6 User\nset time (sec)" -> [w3591]
              i -> [w3590]
              stop <- w3582 stop-if-true
              n1434 = local read "SO2 Calibration Abort"() -> (w3588:bool)
              n1435 = case shown="True" w3588 {
                selector: w3588 -> [w3594 _]
                tunnel: [w3594 w3595] -> w3583
                frame False {
                }
                frame True {
                  n1436 = Two Button Dialog(message="Are you sure to abort SO2 Zeroing?") -> (T button?=w3595:bool)  [unwired: 2 in]
                }
              }
              n1437 = Subtract(x=w3591, y=w3590) -> (x-y=w3589:i32)
              n1438 = Decrement(x=w3589) -> (x-1=w3585:i32)
              n1439 = Wait (ms)(milliseconds to wait=u32 1000) -> ()  [unwired: 1 out]
              n1440 = local read "Network disconnected"() -> (w3586:bool)
              n1441 = Or(x=w3586, y=w3583) -> (x .or. y?=w3582:bool)
              n1442 = case shown="False" w3583 {
                selector: w3583 -> [w3593 _]
                frame False {
                  n1443 = local write "SO2 Calibration Abort"(w3593) -> ()
                }
                frame True {
                }
              }
              n1444 = Select(t=0, s=w3582, f=w3585) -> (s? t:f=w3584:i32)
              n1445 = local write "SO2 Zeroing\nTime Remain (sec)"(w3584) -> ()
            }
          }
          frame #2 {
            w3597 = FALSE
            n1446 = Bundle(cluster=T5 {"Message"="", "Message Data"=variant} ("Message Cluster"), "Message"="V6", "Message Data"=w3597) -> (w3601:T5)
            n1447 = local write "SO2 eV6"(w3597) -> ()
            n1448 = Enqueue Element(queue=w3600, element=w3601, error in (no error)=w3599) -> (error out=w3598:errorcluster)  [unwired: 1 in, 2 out]
          }
          frame #3 {
            n1449 = local write "SO2 GND Zeroing"(FALSE ("SO2 Flush")) -> ()
          }
        }
      }
      event "SO2 Inflight \nZeroing": Value Change {
        n1450 = event-data() -> ()  [unwired: 1 in, 1 out]
        n1451 = flat-sequence {
          tunnel: w3613 -> [w3621]
          tunnel: w3612 -> [w3620]
          tunnel: [w3616] -> w3610
          tunnel: [w3614] -> w3606
          tunnel: w3610 -> [w3624]
          tunnel: [w3624] -> w3609
          tunnel: [w3623] -> w3607
          tunnel: w3606 -> [w3623]
          tunnel: w3609 -> [w3632]
          tunnel: [w3631] -> w3608
          tunnel: w3607 -> [w3633]
          tunnel: [w3638] -> w3611
          tunnel: w3608 -> [w3638]
          frame #0 {
            w3615 = TRUE ("SO2 Flush")
            n1452 = local write "SO2 eV6"(w3615) -> ()
            n1453 = Bundle(cluster=T5 {"Message"="", "Message Data"=variant} ("Message Cluster"), "Message"="V6", "Message Data"=w3615) -> (w3617:T5)
            n1454 = Enqueue Element(queue=w3621, element=w3617, error in (no error)=w3620) -> (queue out=w3614:refnum<queue>, error out=w3616:errorcluster)  [unwired: 1 in, 1 out]
          }
          frame #1 {
            n1455 = for {
              N: "eV6 User set time \n(Inflight) (sec)" -> [w3628]
              i -> [w3627]
              n1456 = Subtract(x=w3628, y=w3627) -> (x-y=w3626:i32)
              n1457 = Decrement(x=w3626) -> (x-1=w3625:i32)
              n1458 = local write "SO2 Zeroing (Inflight)\nTime Remain (sec)"(w3625) -> ()
              n1459 = Wait (ms)(milliseconds to wait=u32 1000) -> ()  [unwired: 1 out]
            }
          }
          frame #2 {
            w3630 = FALSE
            n1460 = Bundle(cluster=T5 {"Message"="", "Message Data"=variant} ("Message Cluster"), "Message"="V6", "Message Data"=w3630) -> (w3634:T5)
            n1461 = local write "SO2 eV6"(w3630) -> ()
            n1462 = Enqueue Element(queue=w3633, element=w3634, error in (no error)=w3632) -> (error out=w3631:errorcluster)  [unwired: 1 in, 2 out]
          }
          frame #3 {
            n1463 = local write "SO2 Inflight \nZeroing"(FALSE ("SO2 Flush")) -> ()
          }
        }
      }
      event "SO2 Zero CAL": Value Change {
        n1464 = event-data() -> ()  [unwired: 1 in, 1 out]
        n1465 = flat-sequence {
          tunnel: [w3651] -> w3646
          tunnel: [w3650] -> w3644
          tunnel: w3648 -> [w3656]
          tunnel: w3647 -> [w3655]
          tunnel: w3646 -> [w3660]
          tunnel: [w3659] -> w3645
          tunnel: w3644 -> [w3661]
          tunnel: [w3657] -> w3643
          tunnel: [w3667] -> w3642
          tunnel: [w3666] -> w3641
          tunnel: w3643 -> [w3671]
          tunnel: w3645 -> [w3669]
          tunnel: w3642 -> [w3723]
          tunnel: w3641 -> [w3722]
          tunnel: [w3721] -> w3640
          tunnel: [w3720] -> w3639
          tunnel: w3640 -> [w3737]
          tunnel: w3639 -> [w3736]
          frame #0 {
            w3649 = TRUE ("SO2 Flush")
            n1466 = Bundle(cluster=T5 {"Message"="", "Message Data"=variant} ("Message Cluster"), "Message"="V9", "Message Data"=w3649) -> (w3652:T5)
            n1467 = local write "eV9"(w3649) -> ()
            n1468 = Enqueue Element(queue=w3656, element=w3652, error in (no error)=w3655) -> (queue out=w3650:refnum<queue>, error out=w3651:errorcluster)  [unwired: 1 in, 1 out]
          }
          frame #1 {
            n1469 = local read "MFC_2 User Set Value"() -> (w3658:dbl)
            n1470 = local write "MFC_2\nSLPM Value"(w3658) -> ()
            n1471 = Bundle(cluster=T5 {"Message"="", "Message Data"=variant} ("Message Cluster"), "Message"="MFC_2", "Message Data"=w3658) -> (w3662:T5)
            n1472 = Enqueue Element(queue=w3661, element=w3662, error in (no error)=w3660) -> (queue out=w3657:refnum<queue>, error out=w3659:errorcluster)  [unwired: 1 in, 1 out]
          }
          frame #2 {
            n1473 = for {
              N: "eV9 flush User\nset time (sec)" -> [w3714]
              tunnel: [w3705] -> w3670
              tunnel: w3671 -> [w3705]
              tunnel: [w3704] -> w3668
              tunnel: w3669 -> [w3704]
              tunnel: [w3703] -> w3665
              i -> [w3713]
              stop <- w3703 stop-if-true
              n1474 = local read "SO2 Calibration Abort"() -> (w3710:bool)
              n1475 = case shown="True" w3710 {
                selector: w3710 -> [w3717 _]
                tunnel: [w3717 w3718] -> w3708
                frame False {
                }
                frame True {
                  n1476 = Two Button Dialog(message="Are you sure to abort SO2 Cal?") -> (T button?=w3718:bool)  [unwired: 2 in]
                }
              }
              n1477 = Subtract(x=w3714, y=w3713) -> (x-y=w3712:i32)
              n1478 = Decrement(x=w3712) -> (x-1=w3706:i32)
              n1479 = Wait (ms)(milliseconds to wait=u32 1000) -> ()  [unwired: 1 out]
              n1480 = local read "Network disconnected"() -> (w3709:bool)
              n1481 = Or(x=w3709, y=w3708) -> (x .or. y?=w3703:bool)
              n1482 = Select(t=0, s=w3703, f=w3706) -> (s? t:f=w3707:i32)
              n1483 = local write "SO2 Zero CAL Flush\nTime Remain (sec)"(w3707) -> ()
              n1484 = case shown="False" w3708 {
                selector: w3708 -> [w3716 _]
                frame False {
                  n1485 = local write "SO2 Calibration Abort"(w3716) -> ()
                }
                frame True {
                }
              }
            }
            n1486 = case shown="False" w3665 {
              tunnel: w3670 -> [w3678 w3702]
              tunnel: w3668 -> [w3677 w3701]
              tunnel: [w3675 w3702] -> w3667
              tunnel: [w3673 w3701] -> w3666
              frame False {
                w3679 = TRUE ("SO2 Flush")
                # "carry on cal when no connection problem or abort not confirmed"
                n1487 = Bundle(cluster=T5 {"Message"="", "Message Data"=variant} ("Message Cluster"), "Message"="V8", "Message Data"=w3679) -> (w3680:T5)
                n1488 = local write "eV8"(w3679) -> ()
                n1489 = Enqueue Element(queue=w3678, element=w3680, error in (no error)=w3677) -> (queue out=w3676:refnum<queue>, error out=w3674:errorcluster)  [unwired: 1 in, 1 out]
                n1490 = for {
                  N: "eV8 User\nset time (sec)" -> [w3695]
                  tunnel: [w3685] -> w3675
                  tunnel: w3676 -> [w3685]
                  tunnel: [w3684] -> w3673
                  tunnel: w3674 -> [w3684]
                  i -> [w3694]
                  stop <- w3686 stop-if-true
                  n1491 = local read "SO2 Calibration Abort"() -> (w3692:bool)
                  n1492 = case shown="True" w3692 {
                    selector: w3692 -> [w3698 _]
                    tunnel: [w3698 w3699] -> w3689
                    frame False {
                    }
                    frame True {
                      n1493 = Two Button Dialog(message="Are you sure to abort SO2 Cal?") -> (T button?=w3699:bool)  [unwired: 2 in]
                    }
                  }
                  n1494 = Subtract(x=w3695, y=w3694) -> (x-y=w3693:i32)
                  n1495 = local read "Network disconnected"() -> (w3690:bool)
                  n1496 = Decrement(x=w3693) -> (x-1=w3688:i32)
                  n1497 = Or(x=w3690, y=w3689) -> (x .or. y?=w3686:bool)
                  n1498 = Select(t=0, s=w3686, f=w3688) -> (s? t:f=w3687:i32)
                  n1499 = case shown="False" w3689 {
                    selector: w3689 -> [w3697 _]
                    frame False {
                      n1500 = local write "SO2 Calibration Abort"(w3697) -> ()
                    }
                    frame True {
                    }
                  }
                  n1501 = local write "SO2 Zero CAL\nTime Remain (sec)"(w3687) -> ()
                  n1502 = Wait (ms)(milliseconds to wait=u32 1000) -> ()  [unwired: 1 out]
                }
              }
              frame True {
                # "Ignore the rest of the cal when there is connection problem or abort confirmed"
              }
            }
          }
          frame #3 {
            n1503 = Cluster To Array(cluster=cluster{"Message":string, "Message 2":string} {"Message"="V8", "Message 2"="V9"}) -> (array=w3725:string[])
            n1504 = for {
              tunnel: w3725 -> [w3732] mode=indexing
              tunnel: FALSE ("SO2 Flush") -> [w3731]
              tunnel: w3723 -> [w3730]
              tunnel: w3722 -> [w3729]
              tunnel: [w3728] -> w3721
              tunnel: [w3727] -> w3720
              n1505 = Bundle(cluster=T5 {"Message"="", "Message Data"=variant} ("Message Cluster"), "Message"=w3732, "Message Data"=w3731) -> (w3733:T5)
              n1506 = Enqueue Element(queue=w3730, element=w3733, error in (no error)=w3729) -> (queue out=w3728:refnum<queue>, error out=w3727:errorcluster)  [unwired: 1 in, 1 out]
            }
          }
          frame #4 {
            w3735 = 0.0 ("MFC_2\nSLPM Value")
            n1507 = local write "MFC_2\nSLPM Value"(w3735) -> ()
            n1508 = Bundle(cluster=T5 {"Message"="", "Message Data"=variant} ("Message Cluster"), "Message"="MFC_2", "Message Data"=w3735) -> (w3738:T5)
            n1509 = Enqueue Element(queue=w3737, element=w3738, error in (no error)=w3736) -> ()  [unwired: 1 in, 3 out]
          }
          frame #5 {
            w3741 = FALSE ("SO2 Flush")
            n1510 = local write "eV9"(w3741) -> ()
            n1511 = local write "eV8"(w3741) -> ()
            n1512 = local write "SO2 Zero CAL"(w3741) -> ()
            n1513 = local write "SO2 Calibration Abort"(w3741) -> ()
          }
        }
      }
      event "SO2 Span Calibration": Value Change {
        n1514 = event-data() -> ()  [unwired: 1 in, 1 out]
        n1515 = flat-sequence {
          tunnel: w3758 -> [w3763]
          tunnel: w3759 -> [w3764]
          tunnel: [w3761] -> w3747
          tunnel: [w3762] -> w3746
          tunnel: [w3771] -> w3745
          tunnel: [w3769] -> w3743
          tunnel: w3747 -> [w3772]
          tunnel: w3746 -> [w3773]
          tunnel: w3745 -> [w3780]
          tunnel: [w3779] -> w3744
          tunnel: w3743 -> [w3778]
          tunnel: [w3777] -> w3742
          tunnel: [w3794] -> w3757
          tunnel: [w3793] -> w3755
          tunnel: w3744 -> [w3798]
          tunnel: w3742 -> [w3791]
          tunnel: w3757 -> [w3802]
          tunnel: [w3801] -> w3756
          tunnel: w3755 -> [w3803]
          tunnel: [w3799] -> w3754
          tunnel: [w3810] -> w3753
          tunnel: [w3809] -> w3752
          tunnel: w3754 -> [w3814]
          tunnel: w3756 -> [w3812]
          tunnel: w3753 -> [w3865]
          tunnel: w3752 -> [w3864]
          tunnel: [w3863] -> w3751
          tunnel: [w3862] -> w3750
          tunnel: w3751 -> [w3881]
          tunnel: w3750 -> [w3880]
          tunnel: [w3878] -> w3749
          tunnel: [w3877] -> w3748
          tunnel: w3749 -> [w3886]
          tunnel: w3748 -> [w3885]
          frame #0 {
            n1516 = local write "SO2 Auto Zeroing"(FALSE ("SO2 Auto Zeroing")) -> ()
            n1517 = Bundle(cluster=T5 {"Message"="", "Message Data"=variant} ("Message Cluster"), "Message"="Auto_zero", "Message Data"=FALSE) -> (w3766:T5)
            n1518 = Enqueue Element(queue=w3764, element=w3766, error in (no error)=w3763) -> (queue out=w3761:refnum<queue>, error out=w3762:errorcluster)  [unwired: 1 in, 1 out]
          }
          frame #1 {
            n1519 = Bundle(cluster=T5 {"Message"="", "Message Data"=variant} ("Message Cluster"), "Message"="mean_cal_status", "Message Data"=FALSE) -> (w3774:T5)
            n1520 = Enqueue Element(queue=w3772, element=w3774, error in (no error)=w3773) -> (queue out=w3769:refnum<queue>, error out=w3771:errorcluster)  [unwired: 1 in, 1 out]
          }
          frame #2 {
            n1521 = node-c288() -> (w3782:T6)  [unwired: 4 in]
            n1522 = timed-loop {
              timing: w3782 -> [_]
              timing-out: [_] -> w3781
              tunnel: [w3784] -> w3779
              tunnel: w3780 -> [w3784]
              tunnel: w3778 -> [w3783]
              tunnel: [w3783] -> w3777
              stop <- w3785 stop-if-true
              n1523 = node-c288() -> ()  [unwired: 1 in, 1 out]
              n1524 = node-c288() -> ()  [unwired: 1 in, 1 out]
              n1525 = One Button Dialog(message="Is Span Gas connected to CALDECK?") -> (true=w3785:bool)  [unwired: 1 in]
            }
            n1526 = node-c288(w3781) -> ()  [unwired: 1 out]
          }
          frame #3 {
            w3792 = TRUE ("SO2 Flush")
            n1527 = Bundle(cluster=T5 {"Message"="", "Message Data"=variant} ("Message Cluster"), "Message"="V9", "Message Data"=w3792) -> (w3795:T5)
            n1528 = local write "eV9"(w3792) -> ()
            n1529 = Enqueue Element(queue=w3791, element=w3795, error in (no error)=w3798) -> (queue out=w3793:refnum<queue>, error out=w3794:errorcluster)  [unwired: 1 in, 1 out]
          }
          frame #4 {
            n1530 = local read "MFC_2 User Set Value"() -> (w3800:dbl)
            n1531 = local write "MFC_2\nSLPM Value"(w3800) -> ()
            n1532 = Bundle(cluster=T5 {"Message"="", "Message Data"=variant} ("Message Cluster"), "Message"="MFC_2", "Message Data"=w3800) -> (w3804:T5)
            n1533 = Enqueue Element(queue=w3803, element=w3804, error in (no error)=w3802) -> (queue out=w3799:refnum<queue>, error out=w3801:errorcluster)  [unwired: 1 in, 1 out]
          }
          frame #5 {
            n1534 = for {
              N: "eV9 span\nflush (sec)" -> [w3856]
              tunnel: [w3847] -> w3813
              tunnel: w3814 -> [w3847]
              tunnel: [w3846] -> w3811
              tunnel: w3812 -> [w3846]
              tunnel: [w3845] -> w3808
              i -> [w3855]
              stop <- w3845 stop-if-true
              n1535 = local read "SO2 Calibration Abort"() -> (w3852:bool)
              n1536 = case shown="True" w3852 {
                selector: w3852 -> [w3859 _]
                tunnel: [w3859 w3860] -> w3850
                frame False {
                }
                frame True {
                  n1537 = Two Button Dialog(message="Are you sure to abort SO2 Cal?") -> (T button?=w3860:bool)  [unwired: 2 in]
                }
              }
              n1538 = Subtract(x=w3856, y=w3855) -> (x-y=w3854:i32)
              n1539 = Decrement(x=w3854) -> (x-1=w3848:i32)
              n1540 = Wait (ms)(milliseconds to wait=u32 1000) -> ()  [unwired: 1 out]
              n1541 = local read "Network disconnected"() -> (w3851:bool)
              n1542 = Or(x=w3851, y=w3850) -> (x .or. y?=w3845:bool)
              n1543 = Select(t=0, s=w3845, f=w3848) -> (s? t:f=w3849:i32)
              n1544 = local write "SO2 Zero CAL Flush\nTime Remain (sec)"(w3849) -> ()
              n1545 = case shown="False" w3850 {
                selector: w3850 -> [w3858 _]
                frame False {
                  n1546 = local write "SO2 Calibration Abort"(w3858) -> ()
                }
                frame True {
                }
              }
            }
            n1547 = case shown="False" w3808 {
              tunnel: w3813 -> [w3821 w3844]
              tunnel: w3811 -> [w3820 w3843]
              tunnel: [w3818 w3844] -> w3810
              tunnel: [w3816 w3843] -> w3809
              frame False {
                w3822 = TRUE ("SO2 Flush")
                # "carry on cal when no connection problem or abort not confirmed"
                n1548 = Bundle(cluster=T5 {"Message"="", "Message Data"=variant} ("Message Cluster"), "Message"="V8", "Message Data"=w3822) -> (w3823:T5)
                n1549 = local write "eV8"(w3822) -> ()
                n1550 = Enqueue Element(queue=w3821, element=w3823, error in (no error)=w3820) -> (queue out=w3819:refnum<queue>, error out=w3817:errorcluster)  [unwired: 1 in, 1 out]
                n1551 = for {
                  N: "eV8 span\n(sec)" -> [w3837]
                  tunnel: [w3827] -> w3818
                  tunnel: w3819 -> [w3827]
                  tunnel: [w3826] -> w3816
                  tunnel: w3817 -> [w3826]
                  i -> [w3836]
                  stop <- w3828 stop-if-true
                  n1552 = local read "SO2 Calibration Abort"() -> (w3834:bool)
                  n1553 = case shown="True" w3834 {
                    selector: w3834 -> [w3840 _]
                    tunnel: [w3840 w3841] -> w3831
                    frame False {
                    }
                    frame True {
                      n1554 = Two Button Dialog(message="Are you sure to abort SO2 Cal?") -> (T button?=w3841:bool)  [unwired: 2 in]
                    }
                  }
                  n1555 = Subtract(x=w3837, y=w3836) -> (x-y=w3835:i32)
                  n1556 = local read "Network disconnected"() -> (w3832:bool)
                  n1557 = Decrement(x=w3835) -> (x-1=w3830:i32)
                  n1558 = Or(x=w3832, y=w3831) -> (x .or. y?=w3828:bool)
                  n1559 = Select(t=0, s=w3828, f=w3830) -> (s? t:f=w3829:i32)
                  n1560 = case shown="False" w3831 {
                    selector: w3831 -> [w3839 _]
                    frame False {
                      n1561 = local write "SO2 Calibration Abort"(w3839) -> ()
                    }
                    frame True {
                    }
                  }
                  n1562 = local write "SO2 Zero CAL\nTime Remain (sec)"(w3829) -> ()
                  n1563 = Wait (ms)(milliseconds to wait=u32 1000) -> ()  [unwired: 1 out]
                }
              }
              frame True {
                # "Ignore the rest of the cal when there is connection problem or abort confirmed"
              }
            }
          }
          frame #6 {
            n1564 = Cluster To Array(cluster=cluster{"Message":string, "Message 2":string} {"Message"="V8", "Message 2"="V9"}) -> (array=w3867:string[])
            n1565 = for {
              tunnel: w3867 -> [w3874] mode=indexing
              tunnel: FALSE ("SO2 Flush") -> [w3873]
              tunnel: w3865 -> [w3872]
              tunnel: w3864 -> [w3871]
              tunnel: [w3870] -> w3863
              tunnel: [w3869] -> w3862
              n1566 = Bundle(cluster=T5 {"Message"="", "Message Data"=variant} ("Message Cluster"), "Message"=w3874, "Message Data"=w3873) -> (w3875:T5)
              n1567 = Enqueue Element(queue=w3872, element=w3875, error in (no error)=w3871) -> (queue out=w3870:refnum<queue>, error out=w3869:errorcluster)  [unwired: 1 in, 1 out]
            }
          }
          frame #7 {
            w3879 = 0.0 ("MFC_2\nSLPM Value")
            n1568 = local write "MFC_2\nSLPM Value"(w3879) -> ()
            n1569 = Bundle(cluster=T5 {"Message"="", "Message Data"=variant} ("Message Cluster"), "Message"="MFC_2", "Message Data"=w3879) -> (w3882:T5)
            n1570 = Enqueue Element(queue=w3881, element=w3882, error in (no error)=w3880) -> (queue out=w3878:refnum<queue>, error out=w3877:errorcluster)  [unwired: 1 in, 1 out]
          }
          frame #8 {
            n1571 = Bundle(cluster=T5 {"Message"="", "Message Data"=variant} ("Message Cluster"), "Message"="mean_cal_status", "Message Data"=TRUE) -> (w3888:T5)
            n1572 = Enqueue Element(queue=w3886, element=w3888, error in (no error)=w3885) -> ()  [unwired: 1 in, 3 out]
          }
          frame #9 {
            w3891 = FALSE ("SO2 Flush")
            n1573 = local write "eV8"(w3891) -> ()
            n1574 = local write "eV9"(w3891) -> ()
            n1575 = local write "SO2 Span Calibration"(w3891) -> ()
            n1576 = local write "SO2 Calibration Abort"(w3891) -> ()
          }
        }
      }
      event "SO2 Zero Calibration": Value Change {
        n1577 = event-data() -> ()  [unwired: 1 in, 1 out]
        n1578 = flat-sequence {
          tunnel: w3906 -> [w3912]
          tunnel: w3907 -> [w3913]
          tunnel: [w3910] -> w3897
          tunnel: [w3911] -> w3896
          tunnel: [w3919] -> w3895
          tunnel: [w3917] -> w3893
          tunnel: w3897 -> [w3920]
          tunnel: w3896 -> [w3921]
          tunnel: w3895 -> [w3927]
          tunnel: [w3926] -> w3894
          tunnel: w3893 -> [w3928]
          tunnel: [w3925] -> w3892
          tunnel: [w3942] -> w3905
          tunnel: [w3941] -> w3903
          tunnel: w3894 -> [w3946]
          tunnel: w3892 -> [w3939]
          tunnel: w3905 -> [w3950]
          tunnel: [w3949] -> w3904
          tunnel: w3903 -> [w3951]
          tunnel: [w3947] -> w3902
          tunnel: [w3958] -> w3901
          tunnel: [w3957] -> w3900
          tunnel: w3902 -> [w3962]
          tunnel: w3904 -> [w3960]
          tunnel: w3901 -> [w4013]
          tunnel: w3900 -> [w4012]
          tunnel: [w4011] -> w3899
          tunnel: [w4010] -> w3898
          tunnel: w3899 -> [w4027]
          tunnel: w3898 -> [w4026]
          frame #0 {
            n1579 = local write "SO2 Auto Zeroing"(FALSE) -> ()
            n1580 = Bundle(cluster=T5 {"Message"="", "Message Data"=variant} ("Message Cluster"), "Message"="Auto_zero", "Message Data"=FALSE) -> (w3916:T5)
            n1581 = Enqueue Element(queue=w3913, element=w3916, error in (no error)=w3912) -> (queue out=w3910:refnum<queue>, error out=w3911:errorcluster)  [unwired: 1 in, 1 out]
          }
          frame #1 {
            n1582 = Bundle(cluster=T5 {"Message"="", "Message Data"=variant} ("Message Cluster"), "Message"="mean_cal_status", "Message Data"=TRUE) -> (w3922:T5)
            n1583 = Enqueue Element(queue=w3920, element=w3922, error in (no error)=w3921) -> (queue out=w3917:refnum<queue>, error out=w3919:errorcluster)  [unwired: 1 in, 1 out]
          }
          frame #2 {
            n1584 = node-c288() -> (w3930:T6)  [unwired: 4 in]
            n1585 = timed-loop {
              timing: w3930 -> [_]
              timing-out: [_] -> w3929
              tunnel: [w3932] -> w3926
              tunnel: w3927 -> [w3932]
              tunnel: w3928 -> [w3931]
              tunnel: [w3931] -> w3925
              stop <- w3933 stop-if-true
              n1586 = node-c288() -> ()  [unwired: 1 in, 1 out]
              n1587 = node-c288() -> ()  [unwired: 1 in, 1 out]
              n1588 = One Button Dialog(message="Is Zero Gas connected to CALDECK?") -> (true=w3933:bool)  [unwired: 1 in]
            }
            n1589 = node-c288(w3929) -> ()  [unwired: 1 out]
          }
          frame #3 {
            w3940 = TRUE ("SO2 Flush")
            n1590 = Bundle(cluster=T5 {"Message"="", "Message Data"=variant} ("Message Cluster"), "Message"="V9", "Message Data"=w3940) -> (w3943:T5)
            n1591 = local write "eV9"(w3940) -> ()
            n1592 = Enqueue Element(queue=w3939, element=w3943, error in (no error)=w3946) -> (queue out=w3941:refnum<queue>, error out=w3942:errorcluster)  [unwired: 1 in, 1 out]
          }
          frame #4 {
            n1593 = local read "MFC_2 User Set Value"() -> (w3948:dbl)
            n1594 = local write "MFC_2\nSLPM Value"(w3948) -> ()
            n1595 = Bundle(cluster=T5 {"Message"="", "Message Data"=variant} ("Message Cluster"), "Message"="MFC_2", "Message Data"=w3948) -> (w3952:T5)
            n1596 = Enqueue Element(queue=w3951, element=w3952, error in (no error)=w3950) -> (queue out=w3947:refnum<queue>, error out=w3949:errorcluster)  [unwired: 1 in, 1 out]
          }
          frame #5 {
            n1597 = for {
              N: "eV9 zero\nflush (sec)" -> [w4004]
              tunnel: [w3995] -> w3961
              tunnel: w3962 -> [w3995]
              tunnel: [w3994] -> w3959
              tunnel: w3960 -> [w3994]
              tunnel: [w3993] -> w3956
              i -> [w4003]
              stop <- w3993 stop-if-true
              n1598 = local read "SO2 Calibration Abort"() -> (w4000:bool)
              n1599 = case shown="True" w4000 {
                selector: w4000 -> [w4007 _]
                tunnel: [w4007 w4008] -> w3998
                frame False {
                }
                frame True {
                  n1600 = Two Button Dialog(message="Are you sure to abort SO2 Cal?") -> (T button?=w4008:bool)  [unwired: 2 in]
                }
              }
              n1601 = Subtract(x=w4004, y=w4003) -> (x-y=w4002:i32)
              n1602 = Decrement(x=w4002) -> (x-1=w3996:i32)
              n1603 = Wait (ms)(milliseconds to wait=u32 1000) -> ()  [unwired: 1 out]
              n1604 = local read "Network disconnected"() -> (w3999:bool)
              n1605 = Or(x=w3999, y=w3998) -> (x .or. y?=w3993:bool)
              n1606 = Select(t=0, s=w3993, f=w3996) -> (s? t:f=w3997:i32)
              n1607 = local write "SO2 Zero CAL Flush\nTime Remain (sec)"(w3997) -> ()
              n1608 = case shown="False" w3998 {
                selector: w3998 -> [w4006 _]
                frame False {
                  n1609 = local write "SO2 Calibration Abort"(w4006) -> ()
                }
                frame True {
                }
              }
            }
            n1610 = case shown="False" w3956 {
              tunnel: w3961 -> [w3969 w3992]
              tunnel: w3959 -> [w3968 w3991]
              tunnel: [w3966 w3992] -> w3958
              tunnel: [w3964 w3991] -> w3957
              frame False {
                w3970 = TRUE ("SO2 Flush")
                # "carry on cal when no connection problem or abort not confirmed"
                n1611 = Bundle(cluster=T5 {"Message"="", "Message Data"=variant} ("Message Cluster"), "Message"="V8", "Message Data"=w3970) -> (w3971:T5)
                n1612 = local write "eV8"(w3970) -> ()
                n1613 = Enqueue Element(queue=w3969, element=w3971, error in (no error)=w3968) -> (queue out=w3967:refnum<queue>, error out=w3965:errorcluster)  [unwired: 1 in, 1 out]
                n1614 = for {
                  N: "eV8 zero\n(sec)" -> [w3985]
                  tunnel: [w3975] -> w3966
                  tunnel: w3967 -> [w3975]
                  tunnel: [w3974] -> w3964
                  tunnel: w3965 -> [w3974]
                  i -> [w3984]
                  stop <- w3976 stop-if-true
                  n1615 = local read "SO2 Calibration Abort"() -> (w3982:bool)
                  n1616 = case shown="True" w3982 {
                    selector: w3982 -> [w3988 _]
                    tunnel: [w3988 w3989] -> w3979
                    frame False {
                    }
                    frame True {
                      n1617 = Two Button Dialog(message="Are you sure to abort SO2 Cal?") -> (T button?=w3989:bool)  [unwired: 2 in]
                    }
                  }
                  n1618 = Subtract(x=w3985, y=w3984) -> (x-y=w3983:i32)
                  n1619 = local read "Network disconnected"() -> (w3980:bool)
                  n1620 = Decrement(x=w3983) -> (x-1=w3978:i32)
                  n1621 = Or(x=w3980, y=w3979) -> (x .or. y?=w3976:bool)
                  n1622 = Select(t=0, s=w3976, f=w3978) -> (s? t:f=w3977:i32)
                  n1623 = case shown="False" w3979 {
                    selector: w3979 -> [w3987 _]
                    frame False {
                      n1624 = local write "SO2 Calibration Abort"(w3987) -> ()
                    }
                    frame True {
                    }
                  }
                  n1625 = local write "SO2 Zero CAL\nTime Remain (sec)"(w3977) -> ()
                  n1626 = Wait (ms)(milliseconds to wait=u32 1000) -> ()  [unwired: 1 out]
                }
              }
              frame True {
                # "Ignore the rest of the cal when there is connection problem or abort confirmed"
              }
            }
          }
          frame #6 {
            n1627 = Cluster To Array(cluster=cluster{"Message":string, "Message 2":string} {"Message"="V8", "Message 2"="V9"}) -> (array=w4015:string[])
            n1628 = for {
              tunnel: w4015 -> [w4022] mode=indexing
              tunnel: FALSE ("SO2 Flush") -> [w4021]
              tunnel: w4013 -> [w4020]
              tunnel: w4012 -> [w4019]
              tunnel: [w4018] -> w4011
              tunnel: [w4017] -> w4010
              n1629 = Bundle(cluster=T5 {"Message"="", "Message Data"=variant} ("Message Cluster"), "Message"=w4022, "Message Data"=w4021) -> (w4023:T5)
              n1630 = Enqueue Element(queue=w4020, element=w4023, error in (no error)=w4019) -> (queue out=w4018:refnum<queue>, error out=w4017:errorcluster)  [unwired: 1 in, 1 out]
            }
          }
          frame #7 {
            w4025 = 0.0 ("MFC_2\nSLPM Value")
            n1631 = local write "MFC_2\nSLPM Value"(w4025) -> ()
            n1632 = Bundle(cluster=T5 {"Message"="", "Message Data"=variant} ("Message Cluster"), "Message"="MFC_2", "Message Data"=w4025) -> (w4028:T5)
            n1633 = Enqueue Element(queue=w4027, element=w4028, error in (no error)=w4026) -> ()  [unwired: 1 in, 3 out]
          }
          frame #8 {
            w4031 = FALSE ("SO2 Flush")
            n1634 = local write "eV8"(w4031) -> ()
            n1635 = local write "eV9"(w4031) -> ()
            n1636 = local write "SO2 Zero Calibration"(w4031) -> ()
            n1637 = local write "SO2 Calibration Abort"(w4031) -> ()
          }
        }
      }
      event "eV8 User\nset time (sec)": Value Change {
        n1638 = event-data() -> ("NewVal"=w4034:i32)  [unwired: 1 in]
        n1639 = Bundle(cluster=T5 {"Message"="", "Message Data"=variant} ("Message Cluster"), "Message"="eV8_user_set_time", "Message Data"=w4034) -> (w4035:T5)
        n1640 = Enqueue Element(queue=w4033, element=w4035, error in (no error)=w4032) -> ()  [unwired: 1 in, 3 out]
      }
      event "Offset Mean Zero Calculation (default = ON)\nOFF = User input\nOn = Mean zero calculated with ev8": Value Change {
        n1641 = event-data() -> ("NewVal"=w4040:bool)  [unwired: 1 in]
        n1642 = Bundle(cluster=T5 {"Message"="", "Message Data"=variant} ("Message Cluster"), "Message"="mean_cal_status", "Message Data"=w4040) -> (w4041:T5)
        n1643 = Enqueue Element(queue=w4039, element=w4041, error in (no error)=w4038) -> ()  [unwired: 1 in, 3 out]
      }
      event "MFC_2\nSLPM Value": Value Change {
        n1644 = event-data() -> ("NewVal"=w4047:dbl)  [unwired: 1 in]
        n1645 = Bundle(cluster=T5 {"Message"="", "Message Data"=variant} ("Message Cluster"), "Message"="MFC_2", "Message Data"=w4047) -> (w4045:T5)
        n1646 = Enqueue Element(queue=w4050, element=w4045, error in (no error)=w4049) -> (error out=w4044:errorcluster)  [unwired: 1 in, 2 out]
      }
      event "SO2 Inflight MOCCA Alarm\n(default = OFF)": Value Change {
        n1647 = event-data() -> ("NewVal"=w4054:bool)  [unwired: 1 in]
        n1648 = Bundle(cluster=T5 {"Message"="", "Message Data"=variant} ("Message Cluster"), "Message"="SO2_MOCCA_Alarm", "Message Data"=w4054) -> (w4055:T5)
        n1649 = Enqueue Element(queue=w4053, element=w4055, error in (no error)=w4052) -> (error out=w4051:errorcluster)  [unwired: 1 in, 2 out]
      }
      event "MOCCA window \ndelay time (sec)": Value Change {
        n1650 = event-data() -> ("NewVal"=w4060:i32)  [unwired: 1 in]
        n1651 = Bundle(cluster=T5 {"Message"="", "Message Data"=variant} ("Message Cluster"), "Message"="MOCCA_window_delay_time", "Message Data"=w4060) -> (w4062:T5)
        n1652 = Enqueue Element(queue=w4061, element=w4062, error in (no error)=w4059) -> (error out=w4058:errorcluster)  [unwired: 1 in, 2 out]
      }
      event "MOCCA Limit": Value Change {
        n1653 = event-data() -> ("NewVal"=w4065:i32)  [unwired: 1 in]
        n1654 = Bundle(cluster=T5 {"Message"="", "Message Data"=variant} ("Message Cluster"), "Message"="MOCCA_limit", "Message Data"=w4065) -> (w4068:T5)
        n1655 = Enqueue Element(queue=w4067, element=w4068, error in (no error)=w4066) -> ()  [unwired: 1 in, 3 out]
      }
      event "Save Calibration gas\ncylinder concentration to file": Value Change {
        n1656 = event-data() -> ("NewVal"=w4071:bool)  [unwired: 1 in]
        n1657 = Bundle(cluster=T5 {"Message"="", "Message Data"=variant} ("Message Cluster"), "Message"="calcon_save", "Message Data"=w4071) -> (w4075:T5)
        n1658 = Enqueue Element(queue=w4074, element=w4075, error in (no error)=w4073) -> (error out=w4072:errorcluster)  [unwired: 1 in, 2 out]
      }
      event "Calibration gas cylinder \nconcentration (ppb)": Value Change {
        n1659 = event-data() -> ("NewVal"=w4078:dbl)  [unwired: 1 in]
        n1660 = Bundle(cluster=T5 {"Message"="", "Message Data"=variant} ("Message Cluster"), "Message"="cal_gas_cylin_conc", "Message Data"=w4078) -> (w4081:T5)
        n1661 = Enqueue Element(queue=w4080, element=w4081, error in (no error)=w4079) -> ()  [unwired: 1 in, 3 out]
      }
      event "Simulate MOCCA Conc": Value Change {
        n1662 = event-data() -> ("NewVal"=w4084:dbl)  [unwired: 1 in]
        n1663 = Bundle(cluster=T5 {"Message"="", "Message Data"=variant} ("Message Cluster"), "Message"="sim_MOCCA_conc", "Message Data"=w4084) -> (w4087:T5)
        n1664 = Enqueue Element(queue=w4086, element=w4087, error in (no error)=w4085) -> ()  [unwired: 1 in, 3 out]
      }
      event "MFC_3\nSLPM Value": Value Change {
        n1665 = event-data() -> ("NewVal"=w4093:dbl)  [unwired: 1 in]
        n1666 = Bundle(cluster=T5 {"Message"="", "Message Data"=variant} ("Message Cluster"), "Message"="MFC_3", "Message Data"=w4093) -> (w4091:T5)
        n1667 = Enqueue Element(queue=w4096, element=w4091, error in (no error)=w4095) -> (error out=w4090:errorcluster)  [unwired: 1 in, 2 out]
      }
      event "eV8": Value Change {
        n1668 = event-data() -> ("NewVal"=w4097:bool)  [unwired: 1 in]
        n1669 = Bundle(cluster=T5 {"Message"="", "Message Data"=variant} ("Message Cluster"), "Message"="V8", "Message Data"=w4097) -> (w4101:T5)
        n1670 = Enqueue Element(queue=w4100, element=w4101, error in (no error)=w4099) -> (error out=w4098:errorcluster)  [unwired: 1 in, 2 out]
      }
      event "SO2 eV6": Value Change {
        n1671 = event-data() -> ("NewVal"=w4104:bool)  [unwired: 1 in]
        n1672 = Bundle(cluster=T5 {"Message"="", "Message Data"=variant} ("Message Cluster"), "Message"="V6", "Message Data"=w4104) -> (w4108:T5)
        n1673 = Enqueue Element(queue=w4107, element=w4108, error in (no error)=w4106) -> (error out=w4105:errorcluster)  [unwired: 1 in, 2 out]
      }
      event "Simulate Conc": Value Change {
        n1674 = event-data() -> ("NewVal"=w4111:bool)  [unwired: 1 in]
        n1675 = Bundle(cluster=T5 {"Message"="", "Message Data"=variant} ("Message Cluster"), "Message"="Simulate Conc", "Message Data"=w4111) -> (w4115:T5)
        n1676 = Enqueue Element(queue=w4114, element=w4115, error in (no error)=w4113) -> (error out=w4112:errorcluster)  [unwired: 1 in, 2 out]
      }
      event "SO2 UDP Time Offset": Value Change {
        n1677 = event-data() -> ("NewVal"=w4118:i32)  [unwired: 1 in]
        n1678 = Bundle(cluster=T5 {"Message"="", "Message Data"=variant} ("Message Cluster"), "Message"="UDP Time Offset", "Message Data"=w4118) -> (w4122:T5)
        n1679 = Enqueue Element(queue=w4121, element=w4122, error in (no error)=w4120) -> (error out=w4119:errorcluster)  [unwired: 1 in, 2 out]
      }
      event "Simulate STEL Conc": Value Change {
        n1680 = event-data() -> ("NewVal"=w4125:dbl)  [unwired: 1 in]
        n1681 = Bundle(cluster=T5 {"Message"="", "Message Data"=variant} ("Message Cluster"), "Message"="Simulate STEL Conc", "Message Data"=w4125) -> (w4129:T5)
        n1682 = Enqueue Element(queue=w4128, element=w4129, error in (no error)=w4127) -> (error out=w4126:errorcluster)  [unwired: 1 in, 2 out]
      }
      event "Simulate TWA Conc": Value Change {
        n1683 = event-data() -> ("NewVal"=w4132:dbl)  [unwired: 1 in]
        n1684 = Bundle(cluster=T5 {"Message"="", "Message Data"=variant} ("Message Cluster"), "Message"="Simulate TWA Conc", "Message Data"=w4132) -> (w4136:T5)
        n1685 = Enqueue Element(queue=w4135, element=w4136, error in (no error)=w4134) -> (error out=w4133:errorcluster)  [unwired: 1 in, 2 out]
      }
      event "10mins STEL Limit": Value Change {
        n1686 = event-data() -> ("NewVal"=w4139:i32)  [unwired: 1 in]
        n1687 = Bundle(cluster=T5 {"Message"="", "Message Data"=variant} ("Message Cluster"), "Message"="10mins STEL Limit", "Message Data"=w4139) -> (w4143:T5)
        n1688 = Enqueue Element(queue=w4142, element=w4143, error in (no error)=w4141) -> (error out=w4140:errorcluster)  [unwired: 1 in, 2 out]
      }
      event "8hr TWA Limit": Value Change {
        n1689 = event-data() -> ("NewVal"=w4146:i32)  [unwired: 1 in]
        n1690 = Bundle(cluster=T5 {"Message"="", "Message Data"=variant} ("Message Cluster"), "Message"="8hr TWA Limit", "Message Data"=w4146) -> (w4150:T5)
        n1691 = Enqueue Element(queue=w4149, element=w4150, error in (no error)=w4148) -> (error out=w4147:errorcluster)  [unwired: 1 in, 2 out]
      }
      event "SO2 Zero": Value Change {
        n1692 = event-data() -> ("NewVal"=w4153:dbl)  [unwired: 1 in]
        n1693 = Bundle(cluster=T5 {"Message"="", "Message Data"=variant} ("Message Cluster"), "Message"="Offset", "Message Data"=w4153) -> (w4157:T5)
        n1694 = Enqueue Element(queue=w4156, element=w4157, error in (no error)=w4155) -> (error out=w4154:errorcluster)  [unwired: 1 in, 2 out]
      }
      event "SO2 Sensitivity": Value Change {
        n1695 = event-data() -> ("NewVal"=w4160:dbl)  [unwired: 1 in]
        n1696 = Bundle(cluster=T5 {"Message"="", "Message Data"=variant} ("Message Cluster"), "Message"="Slope", "Message Data"=w4160) -> (w4164:T5)
        n1697 = Enqueue Element(queue=w4163, element=w4164, error in (no error)=w4162) -> (error out=w4161:errorcluster)  [unwired: 1 in, 2 out]
      }
      event "Confirm Flight Number": Value Change {
        n1698 = event-data() -> ()  [unwired: 1 in, 6 out]
        n1699 = flat-sequence {
          tunnel: w4170 -> [w4173]
          tunnel: w4171 -> [w4174]
          tunnel: [w4174] -> w4168
          tunnel: [w4173] -> w4167
          tunnel: [w4176] -> w4169
          tunnel: w4168 -> [w4178]
          tunnel: w4167 -> [w4177]
          frame #0 {
            n1700 = local write "cRIO File IO Stop\n(USB Flash Drive Unmount)"(FALSE ("cRIO File IO Stop\n(USB Flash Drive Unmount)")) -> ()
          }
          frame #1 {
            n1701 = local read "Flight Number"() -> (w4175:string)
            n1702 = Bundle(cluster=T5 {"Message"="", "Message Data"=variant} ("Message Cluster"), "Message"="Flight Number", "Message Data"=w4175) -> (w4179:T5)
            n1703 = Enqueue Element(queue=w4178, element=w4179, error in (no error)=w4177) -> (error out=w4176:errorcluster)  [unwired: 1 in, 2 out]
          }
        }
      }
      event "cRIO File IO Stop\n(USB Flash Drive Unmount)": Value Change {
        n1704 = event-data() -> ("NewVal"=w4182:bool)  [unwired: 1 in]
        n1705 = Bundle(cluster=T5 {"Message"="", "Message Data"=variant} ("Message Cluster"), "Message"="Stop File Write", "Message Data"=w4182) -> (w4186:T5)
        n1706 = Enqueue Element(queue=w4185, element=w4186, error in (no error)=w4184) -> (error out=w4183:errorcluster)  [unwired: 1 in, 2 out]
      }
    }
    "SO2 Event error out" <- w3490
  }
  n1707 = Create Network Stream Writer Endpoint(6:w56, 7:10 ("writer buffer size"), 9:w51, 10:"//192.168.101.17/command/reader/SO2" ("reader url"), 11:"/command/writer/SO2" ("writer name")) -> (0:w55:errorcluster, 3:w54:refnum<k21>)  [unwired: 2 in]
  n1708 = while {
    tunnel: w15 -> [w4193]
    tunnel: w14 -> [w4192]
    stop <- FALSE stop-if-true
    # "SO2 Auto Zero Handler Loop"
    n1709 = local read "Network disconnected"() -> (w4190:bool)
    n1710 = local read "SO2 Zero CAL"() -> (w4197:bool)
    n1711 = Equal?(x=w4197, y=FALSE) -> (x = y?=w4195:bool)
    n1712 = Equal?(x=w4190, y=FALSE) -> (x = y?=w4189:bool)
    n1713 = Compound Arithmetic op=AND("SO2 Auto Zeroing", w4195, w4189) -> (w4198:bool)
    n1714 = case shown="False" w4198 {
      tunnel: w4193 -> [_ w4217]
      tunnel: w4192 -> [_ w4216]
      frame False {
        n1715 = local write "Auto Zero\nIndicator"("Auto Zero Inactive; Manual Zero Allow" ("Auto Zero Indicator")) -> ()
        n1716 = local write "SO2 Pause\nAuto Zeroing"(FALSE ("SO2 Pause\nAuto Zeroing")) -> ()
        n1717 = property on="SO2 Zero CAL" class="Bool (strict)"("Visible"=TRUE) -> ()  [unwired: 2 in, 2 out]
      }
      frame True {
        n1718 = flat-sequence {
          tunnel: w4216 -> [w4226]
          tunnel: w4217 -> [w4227]
          tunnel: [w4227] -> w4215
          tunnel: [w4226] -> w4214
          tunnel: w4215 -> [w4236]
          tunnel: w4214 -> [w4235]
          tunnel: [w4234] -> w4213
          tunnel: [w4233] -> w4212
          tunnel: [w4242] -> w4223
          tunnel: [w4241] -> w4222
          tunnel: w4213 -> [w4246]
          tunnel: w4212 -> [w4247]
          tunnel: w4223 -> [w4251]
          tunnel: [w4250] -> w4221
          tunnel: w4222 -> [w4252]
          tunnel: [w4249] -> w4220
          tunnel: w4221 -> [w4260]
          tunnel: w4220 -> [w4262]
          tunnel: [w4258] -> w4205
          tunnel: [w4257] -> w4204
          tunnel: [w4312] -> w4219
          tunnel: [w4311] -> w4218
          tunnel: w4205 -> [w4314]
          tunnel: w4204 -> [w4313]
          tunnel: w4219 -> [w4330]
          tunnel: w4218 -> [w4329]
          tunnel: [w4327] -> w4210
          tunnel: [w4326] -> w4209
          tunnel: [w4335] -> w4211
          tunnel: w4210 -> [w4335]
          tunnel: w4209 -> [w4334]
          tunnel: [w4334] -> w4208
          tunnel: [w4340] -> w4207
          tunnel: w4208 -> [w4339]
          tunnel: w4211 -> [w4340]
          tunnel: [w4339] -> w4206
          tunnel: w4207 -> [w4374]
          tunnel: w4206 -> [w4373]
          frame #0 {
            n1719 = local write "Auto Zero\nIndicator"("Auto Zero In Progress" ("Auto Zero\nIndicator")) -> ()
            n1720 = while {
              stop <- w4228 stop-if-true
              n1721 = local read "eV9"() -> (w4230:bool)
              n1722 = Equal?(x=w4230, y=FALSE) -> (x = y?=w4228:bool)
              n1723 = Wait (ms)(milliseconds to wait=u32 1000) -> ()  [unwired: 1 out]
            }
            n1724 = property on="SO2 Zero CAL" class="Bool (strict)"("Visible"=FALSE) -> ()  [unwired: 2 in, 2 out]
          }
          frame #1 {
            n1725 = Bundle(cluster=T5 {"Message"="", "Message Data"=variant} ("Message Cluster"), "Message"="Auto_zero", "Message Data"=TRUE) -> (w4237:T5)
            n1726 = Enqueue Element(queue=w4236, element=w4237, error in (no error)=w4235) -> (queue out=w4233:refnum<queue>, error out=w4234:errorcluster)  [unwired: 1 in, 1 out]
          }
          frame #2 {
            w4240 = TRUE ("SO2 Flush")
            n1727 = Bundle(cluster=T5 {"Message"="", "Message Data"=variant} ("Message Cluster"), "Message"="V9", "Message Data"=w4240) -> (w4243:T5)
            n1728 = local write "eV9"(w4240) -> ()
            n1729 = Enqueue Element(queue=w4247, element=w4243, error in (no error)=w4246) -> (queue out=w4241:refnum<queue>, error out=w4242:errorcluster)  [unwired: 1 in, 1 out]
          }
          frame #3 {
            n1730 = local read "MFC_2 User Set Value"() -> (w4248:dbl)
            n1731 = local write "MFC_2 User Set Value"(w4248) -> ()
            n1732 = Bundle(cluster=T5 {"Message"="", "Message Data"=variant} ("Message Cluster"), "Message"="MFC_2", "Message Data"=w4248) -> (w4253:T5)
            n1733 = Enqueue Element(queue=w4252, element=w4253, error in (no error)=w4251) -> (queue out=w4249:refnum<queue>, error out=w4250:errorcluster)  [unwired: 1 in, 1 out]
          }
          frame #4 {
            n1734 = local read "eV9 flush User\nset time (sec)"() -> (w4263:i32)
            n1735 = for {
              N: w4263 -> [w4305]
              tunnel: [w4296] -> w4261
              tunnel: w4262 -> [w4296]
              tunnel: [w4295] -> w4259
              tunnel: w4260 -> [w4295]
              tunnel: [w4294] -> w4256
              i -> [w4304]
              stop <- w4294 stop-if-true
              n1736 = local read "Network disconnected"() -> (w4298:bool)
              n1737 = local read "SO2 Calibration Abort"() -> (w4299:bool)
              n1738 = case shown="True" w4299 {
                selector: w4299 -> [w4308 _]
                tunnel: [w4308 w4309] -> w4297
                frame False {
                }
                frame True {
                  n1739 = Two Button Dialog(message="Are you sure to abort SO2 Cal?") -> (T button?=w4309:bool)  [unwired: 2 in]
                }
              }
              n1740 = Subtract(x=w4305, y=w4304) -> (x-y=w4303:i32)
              n1741 = Decrement(x=w4303) -> (x-1=w4301:i32)
              n1742 = Or(x=w4297, y=w4298) -> (x .or. y?=w4294:bool)
              n1743 = Wait (ms)(milliseconds to wait=u32 1000) -> ()  [unwired: 1 out]
              n1744 = Select(t=0, s=w4294, f=w4301) -> (s? t:f=w4300:i32)
              n1745 = local write "SO2 Zero CAL Flush\nTime Remain (sec)"(w4300) -> ()
              n1746 = case shown="False" w4297 {
                selector: w4297 -> [w4307 _]
                frame False {
                  n1747 = local write "SO2 Calibration Abort"(w4307) -> ()
                }
                frame True {
                }
              }
            }
            n1748 = case shown="False" w4256 {
              tunnel: w4261 -> [w4269 w4293]
              tunnel: w4259 -> [w4268 w4292]
              tunnel: [w4267 w4293] -> w4258
              tunnel: [w4265 w4292] -> w4257
              frame False {
                w4270 = TRUE ("SO2 Flush")
                # "carry on cal when no connection problem or abort not confirmed"
                n1749 = Bundle(cluster=T5 {"Message"="", "Message Data"=variant} ("Message Cluster"), "Message"="V8", "Message Data"=w4270) -> (w4271:T5)
                n1750 = local write "eV8"(w4270) -> ()
                n1751 = Enqueue Element(queue=w4269, element=w4271, error in (no error)=w4268) -> (queue out=w4266:refnum<queue>, error out=w4264:errorcluster)  [unwired: 1 in, 1 out]
                n1752 = local read "eV8 User\nset time (sec)"() -> (w4274:i32)
                n1753 = for {
                  N: w4274 -> [w4286]
                  tunnel: w4266 -> [w4276]
                  tunnel: [w4276] -> w4267
                  tunnel: w4264 -> [w4275]
                  tunnel: [w4275] -> w4265
                  i -> [w4285]
                  stop <- w4277 stop-if-true
                  n1754 = local read "Network disconnected"() -> (w4281:bool)
                  n1755 = local read "SO2 Calibration Abort"() -> (w4283:bool)
                  n1756 = case shown="True" w4283 {
                    selector: w4283 -> [w4289 _]
                    tunnel: [w4289 w4290] -> w4278
                    frame False {
                    }
                    frame True {
                      n1757 = Two Button Dialog(message="Are you sure to abort SO2 Cal?") -> (T button?=w4290:bool)  [unwired: 2 in]
                    }
                  }
                  n1758 = Subtract(x=w4286, y=w4285) -> (x-y=w4284:i32)
                  n1759 = Decrement(x=w4284) -> (x-1=w4279:i32)
                  n1760 = Or(x=w4278, y=w4281) -> (x .or. y?=w4277:bool)
                  n1761 = Wait (ms)(milliseconds to wait=u32 1000) -> ()  [unwired: 1 out]
                  n1762 = Select(t=0, s=w4277, f=w4279) -> (s? t:f=w4280:i32)
                  n1763 = case shown="False" w4278 {
                    selector: w4278 -> [w4288 _]
                    frame False {
                      n1764 = local write "SO2 Calibration Abort"(w4288) -> ()
                    }
                    frame True {
                    }
                  }
                  n1765 = local write "SO2 Zero CAL\nTime Remain (sec)"(w4280) -> ()
                }
              }
              frame True {
                # "Ignore cal when connection problem or abort confirmed"
              }
            }
          }
          frame #5 {
            n1766 = Cluster To Array(cluster=cluster{"Message":string, "Message 2":string} {"Message"="V8", "Message 2"="V9"}) -> (array=w4316:string[])
            n1767 = for {
              tunnel: w4316 -> [w4323] mode=indexing
              tunnel: FALSE ("SO2 Flush") -> [w4322]
              tunnel: w4314 -> [w4321]
              tunnel: w4313 -> [w4320]
              tunnel: [w4319] -> w4312
              tunnel: [w4318] -> w4311
              n1768 = Bundle(cluster=T5 {"Message"="", "Message Data"=variant} ("Message Cluster"), "Message"=w4323, "Message Data"=w4322) -> (w4324:T5)
              n1769 = Enqueue Element(queue=w4321, element=w4324, error in (no error)=w4320) -> (queue out=w4319:refnum<queue>, error out=w4318:errorcluster)  [unwired: 1 in, 1 out]
            }
          }
          frame #6 {
            w4328 = 0.0 ("MFC_2\nSLPM Value")
            n1770 = local write "MFC_2\nSLPM Value"(w4328) -> ()
            n1771 = Bundle(cluster=T5 {"Message"="", "Message Data"=variant} ("Message Cluster"), "Message"="MFC_2", "Message Data"=w4328) -> (w4331:T5)
            n1772 = Enqueue Element(queue=w4330, element=w4331, error in (no error)=w4329) -> (queue out=w4327:refnum<queue>, error out=w4326:errorcluster)  [unwired: 1 in, 1 out]
          }
          frame #7 {
            w4336 = FALSE ("SO2 Flush")
            n1773 = local write "eV8"(w4336) -> ()
            n1774 = local write "eV9"(w4336) -> ()
          }
          frame #8 {
            n1775 = for {
              N: "Auto Zeroing \ninterval (sec)" -> [w4352]
              tunnel: [w4347] -> w4337
              i -> [w4351]
              stop <- w4347 stop-if-true
              n1776 = local read "SO2 Pause\nAuto Zeroing"() -> (w4345:bool)
              n1777 = Subtract(x=w4352, y=w4351) -> (x-y=w4353:i32)
              n1778 = Equal?(x=w4345, y=TRUE) -> (x = y?=w4343:bool)
              n1779 = Decrement(x=w4353) -> (x-1=→"Next Auto Zero\nStarts in (sec)":i32)
              n1780 = Wait (ms)(milliseconds to wait=u32 1000) -> ()  [unwired: 1 out]
              n1781 = case shown="True" w4343 {
                selector: w4343 -> [w4355 _]
                tunnel: [w4355 FALSE] -> w4342
                frame False {
                }
                frame True {
                  n1782 = for {
                    N: "Pause Auto Zero Count \nDown set time (sec)" -> [w4369]
                    tunnel: [w4361] -> w4357
                    i -> [w4368]
                    stop <- w4361 stop-if-true
                    w4362 = FALSE
                    n1783 = local read "SO2 Pause\nAuto Zeroing"() -> (w4364:bool)
                    n1784 = local read "SO2 Auto Zeroing"() -> (w4365:bool)
                    n1785 = Subtract(x=w4369, y=w4368) -> (x-y=w4370:i32)
                    n1786 = Decrement(x=w4370) -> (x-1=→"SO2 Resume Zeroing\nCount down timer (sec)":i32)
                    n1787 = Wait (ms)(milliseconds to wait=u32 1000) -> ()  [unwired: 1 out]
                    n1788 = Equal?(x=w4365, y=w4362) -> (x = y?=w4366:bool)
                    n1789 = Equal?(x=w4364, y=w4362) -> (x = y?=w4363:bool)
                    n1790 = Or(x=w4366, y=w4363) -> (x .or. y?=w4361:bool)
                  }
                  n1791 = case shown="True" w4357 {
                    frame False {
                    }
                    frame True {
                      n1792 = local write "SO2 Resume Zeroing\nCount down timer (sec)"(u32 0 ("SO2 Resume Zeroing\nCount down timer (sec)")) -> ()
                    }
                  }
                  n1793 = local write "Auto Zero\nIndicator"("Auto Zero Paused" ("Auto Zero\nIndicator")) -> ()
                }
              }
              n1794 = local write "Auto Zero\nIndicator"("Waiting For The Next Zeroing\nInterrupt Waiting by Pressing Pause Auto Zeroing button " ("Auto Zero\nIndicator")) -> ()
              n1795 = local read "SO2 Auto Zeroing"() -> (w4348:bool)
              n1796 = local write "SO2 Pause\nAuto Zeroing"(w4342) -> ()
              n1797 = Equal?(x=w4348, y=FALSE) -> (x = y?=w4347:bool)
            }
            n1798 = case shown="True" w4337 {
              frame False {
              }
              frame True {
                n1799 = local write "Next Auto Zero\nStarts in (sec)"(u32 0 ("Next Auto Zero\nStarts in (sec)")) -> ()
              }
            }
          }
          frame #9 {
            n1800 = local write "SO2 Calibration Abort"(FALSE) -> ()
            n1801 = Bundle(cluster=T5 {"Message"="", "Message Data"=variant} ("Message Cluster"), "Message"="Auto_zero", "Message Data"=FALSE) -> (w4377:T5)
            n1802 = Enqueue Element(queue=w4374, element=w4377, error in (no error)=w4373) -> ()  [unwired: 1 in, 3 out]
          }
        }
      }
    }
    n1803 = Wait (ms)(milliseconds to wait=u32 100) -> ()  [unwired: 1 out]
  }
  n1804 = while {
    tunnel: w15 -> [w4386]
    shift-right: [w4381] -> _
    shift-left: w54 -> [w4383]
    shift-right: [w4379] -> w52
    shift-left: w55 -> [w4385]
    tunnel: w14 -> [w4380]
    stop <- w4379 stop-if-true
    # "SO2 UI Command Sender"
    n1805 = Dequeue Element(queue=w4386, error in (no error)=w4380) -> (element=w4382:T5)  [unwired: 1 in, 3 out]
    n1806 = Unbundle By Name(w4382) -> ("Message"=w4384:string)
    n1807 = case shown="\"zeroing_interval\"" w4384 {
      tunnel: w4385 -> [w4387 w4391 w4398 w4405 w4412 w4419 w4426 w4433 w4440 w4447 w4454 w4461 w4468 w4475 w4482 w4489 w4496 w4503 w4510 w4517 w4524 w4531 w4538 w4545 w4552 w4559]
      tunnel: w4383 -> [w4388 w4394 w4401 w4408 w4415 w4422 w4429 w4436 w4443 w4450 w4457 w4464 w4471 w4478 w4485 w4492 w4499 w4506 w4513 w4520 w4527 w4534 w4541 w4548 w4555 w4562]
      tunnel: w4382 -> [_ w4393 w4400 w4407 w4414 w4421 w4428 w4435 w4442 w4449 w4456 w4463 w4470 w4477 w4484 w4491 w4498 w4505 w4512 w4519 w4526 w4533 w4540 w4547 w4554 w4561]
      tunnel: [w4387 w4390 w4397 w4404 w4411 w4418 w4425 w4432 w4439 w4446 w4453 w4460 w4467 w4474 w4481 w4488 w4495 w4502 w4509 w4516 w4523 w4530 w4537 w4544 w4551 w4558] -> w4379
      tunnel: [w4388 w4389 w4396 w4403 w4410 w4417 w4424 w4431 w4438 w4445 w4452 w4459 w4466 w4473 w4480 w4487 w4494 w4501 w4508 w4515 w4522 w4529 w4536 w4543 w4550 w4557] -> w4381
      frame "False", Default {
      }
      frame "V9" {
        n1808 = shared-variable-write(w4394, w4391, w4393) -> (w4392:refnum<k21>, w4395:errorcluster)  [unwired: 1 in, 1 out]
        n1809 = Flush Stream(8:w4395, 11:w4392) -> (0:w4390:errorcluster, 3:w4389:refnum<k21>)  [unwired: 2 in, 1 out]
      }
      frame "MFC_2" {
        n1810 = shared-variable-write(w4401, w4398, w4400) -> (w4399:refnum<k21>, w4402:errorcluster)  [unwired: 1 in, 1 out]
        n1811 = Flush Stream(8:w4402, 11:w4399) -> (0:w4397:errorcluster, 3:w4396:refnum<k21>)  [unwired: 2 in, 1 out]
      }
      frame "MFC_3" {
        n1812 = shared-variable-write(w4408, w4405, w4407) -> (w4406:refnum<k21>, w4409:errorcluster)  [unwired: 1 in, 1 out]
        n1813 = Flush Stream(8:w4409, 11:w4406) -> (0:w4404:errorcluster, 3:w4403:refnum<k21>)  [unwired: 2 in, 1 out]
      }
      frame "V6" {
        n1814 = shared-variable-write(w4415, w4412, w4414) -> (w4413:refnum<k21>, w4416:errorcluster)  [unwired: 1 in, 1 out]
        n1815 = Flush Stream(8:w4416, 11:w4413) -> (0:w4411:errorcluster, 3:w4410:refnum<k21>)  [unwired: 2 in, 1 out]
      }
      frame "Simulate Conc" {
        n1816 = shared-variable-write(w4422, w4419, w4421) -> (w4420:refnum<k21>, w4423:errorcluster)  [unwired: 1 in, 1 out]
        n1817 = Flush Stream(8:w4423, 11:w4420) -> (0:w4418:errorcluster, 3:w4417:refnum<k21>)  [unwired: 2 in, 1 out]
      }
      frame "Simulate STEL Conc" {
        n1818 = shared-variable-write(w4429, w4426, w4428) -> (w4427:refnum<k21>, w4430:errorcluster)  [unwired: 1 in, 1 out]
        n1819 = Flush Stream(8:w4430, 11:w4427) -> (0:w4425:errorcluster, 3:w4424:refnum<k21>)  [unwired: 2 in, 1 out]
      }
      frame "Simulate TWA Conc" {
        n1820 = shared-variable-write(w4436, w4433, w4435) -> (w4434:refnum<k21>, w4437:errorcluster)  [unwired: 1 in, 1 out]
        n1821 = Flush Stream(8:w4437, 11:w4434) -> (0:w4432:errorcluster, 3:w4431:refnum<k21>)  [unwired: 2 in, 1 out]
      }
      frame "10mins STEL Limit" {
        n1822 = shared-variable-write(w4443, w4440, w4442) -> (w4441:refnum<k21>, w4444:errorcluster)  [unwired: 1 in, 1 out]
        n1823 = Flush Stream(8:w4444, 11:w4441) -> (0:w4439:errorcluster, 3:w4438:refnum<k21>)  [unwired: 2 in, 1 out]
      }
      frame "8hr TWA Limit" {
        n1824 = shared-variable-write(w4450, w4447, w4449) -> (w4448:refnum<k21>, w4451:errorcluster)  [unwired: 1 in, 1 out]
        n1825 = Flush Stream(8:w4451, 11:w4448) -> (0:w4446:errorcluster, 3:w4445:refnum<k21>)  [unwired: 2 in, 1 out]
      }
      frame "Offset" {
        n1826 = shared-variable-write(w4457, w4454, w4456) -> (w4455:refnum<k21>, w4458:errorcluster)  [unwired: 1 in, 1 out]
        n1827 = Flush Stream(8:w4458, 11:w4455) -> (0:w4453:errorcluster, 3:w4452:refnum<k21>)  [unwired: 2 in, 1 out]
      }
      frame "eV8_user_set_time" {
        n1828 = shared-variable-write(w4464, w4461, w4463) -> (w4462:refnum<k21>, w4465:errorcluster)  [unwired: 1 in, 1 out]
        n1829 = Flush Stream(8:w4465, 11:w4462) -> (0:w4460:errorcluster, 3:w4459:refnum<k21>)  [unwired: 2 in, 1 out]
      }
      frame "mean_cal_status" {
        n1830 = shared-variable-write(w4471, w4468, w4470) -> (w4469:refnum<k21>, w4472:errorcluster)  [unwired: 1 in, 1 out]
        n1831 = Flush Stream(8:w4472, 11:w4469) -> (0:w4467:errorcluster, 3:w4466:refnum<k21>)  [unwired: 2 in, 1 out]
      }
      frame "SO2_MOCCA_Alarm" {
        n1832 = shared-variable-write(w4478, w4475, w4477) -> (w4476:refnum<k21>, w4479:errorcluster)  [unwired: 1 in, 1 out]
        n1833 = Flush Stream(8:w4479, 11:w4476) -> (0:w4474:errorcluster, 3:w4473:refnum<k21>)  [unwired: 2 in, 1 out]
      }
      frame "MOCCA_window_delay_time" {
        n1834 = shared-variable-write(w4485, w4482, w4484) -> (w4483:refnum<k21>, w4486:errorcluster)  [unwired: 1 in, 1 out]
        n1835 = Flush Stream(8:w4486, 11:w4483) -> (0:w4481:errorcluster, 3:w4480:refnum<k21>)  [unwired: 2 in, 1 out]
      }
      frame "MOCCA_limit" {
        n1836 = shared-variable-write(w4492, w4489, w4491) -> (w4490:refnum<k21>, w4493:errorcluster)  [unwired: 1 in, 1 out]
        n1837 = Flush Stream(8:w4493, 11:w4490) -> (0:w4488:errorcluster, 3:w4487:refnum<k21>)  [unwired: 2 in, 1 out]
      }
      frame "calcon_save" {
        n1838 = shared-variable-write(w4499, w4496, w4498) -> (w4497:refnum<k21>, w4500:errorcluster)  [unwired: 1 in, 1 out]
        n1839 = Flush Stream(8:w4500, 11:w4497) -> (0:w4495:errorcluster, 3:w4494:refnum<k21>)  [unwired: 2 in, 1 out]
      }
      frame "Auto_zero" {
        n1840 = shared-variable-write(w4506, w4503, w4505) -> (w4504:refnum<k21>, w4507:errorcluster)  [unwired: 1 in, 1 out]
        n1841 = Flush Stream(8:w4507, 11:w4504) -> (0:w4502:errorcluster, 3:w4501:refnum<k21>)  [unwired: 2 in, 1 out]
      }
      frame "zeroing_interval" {
        n1842 = shared-variable-write(w4513, w4510, w4512) -> (w4511:refnum<k21>, w4514:errorcluster)  [unwired: 1 in, 1 out]
        n1843 = Flush Stream(8:w4514, 11:w4511) -> (0:w4509:errorcluster, 3:w4508:refnum<k21>)  [unwired: 2 in, 1 out]
      }
      frame "cal_gas_cylin_conc" {
        n1844 = shared-variable-write(w4520, w4517, w4519) -> (w4518:refnum<k21>, w4521:errorcluster)  [unwired: 1 in, 1 out]
        n1845 = Flush Stream(8:w4521, 11:w4518) -> (0:w4516:errorcluster, 3:w4515:refnum<k21>)  [unwired: 2 in, 1 out]
      }
      frame "sim_MOCCA_conc" {
        n1846 = shared-variable-write(w4527, w4524, w4526) -> (w4525:refnum<k21>, w4528:errorcluster)  [unwired: 1 in, 1 out]
        n1847 = Flush Stream(8:w4528, 11:w4525) -> (0:w4523:errorcluster, 3:w4522:refnum<k21>)  [unwired: 2 in, 1 out]
      }
      frame "Slope" {
        n1848 = shared-variable-write(w4534, w4531, w4533) -> (w4532:refnum<k21>, w4535:errorcluster)  [unwired: 1 in, 1 out]
        n1849 = Flush Stream(8:w4535, 11:w4532) -> (0:w4530:errorcluster, 3:w4529:refnum<k21>)  [unwired: 2 in, 1 out]
      }
      frame "Flight Number" {
        n1850 = shared-variable-write(w4541, w4538, w4540) -> (w4539:refnum<k21>, w4542:errorcluster)  [unwired: 1 in, 1 out]
        n1851 = Flush Stream(8:w4542, 11:w4539) -> (0:w4537:errorcluster, 3:w4536:refnum<k21>)  [unwired: 2 in, 1 out]
      }
      frame "Stop File Write" {
        n1852 = shared-variable-write(w4548, w4545, w4547) -> (w4546:refnum<k21>, w4549:errorcluster)  [unwired: 1 in, 1 out]
        n1853 = Flush Stream(8:w4549, 11:w4546) -> (0:w4544:errorcluster, 3:w4543:refnum<k21>)  [unwired: 2 in, 1 out]
      }
      frame "UDP Time Offset" {
        n1854 = shared-variable-write(w4555, w4552, w4554) -> (w4553:refnum<k21>, w4556:errorcluster)  [unwired: 1 in, 1 out]
        n1855 = Flush Stream(8:w4556, 11:w4553) -> (0:w4551:errorcluster, 3:w4550:refnum<k21>)  [unwired: 2 in, 1 out]
      }
      frame "V8" {
        n1856 = shared-variable-write(w4562, w4559, w4561) -> (w4560:refnum<k21>, w4563:errorcluster)  [unwired: 1 in, 1 out]
        n1857 = Flush Stream(8:w4563, 11:w4560) -> (0:w4558:errorcluster, 3:w4557:refnum<k21>)  [unwired: 2 in, 1 out]
      }
    }
  }
  "SO2 command sender \nerror out" <- w52
  n1858 = Obtain Queue(name (unnamed)="TEi43c_Command", element data type=w40) -> (queue out=w49:refnum<queue>, error out=w42:errorcluster)  [unwired: 3 in, 1 out]
  n1859 = Create Network Stream Writer Endpoint(6:w46, 7:10 ("writer buffer size"), 9:w40, 10:"//192.168.101.17/command/reader/TEi43c" ("reader url"), 11:"/command/writer/TEi43c" ("writer name")) -> (0:w45:errorcluster, 3:w44:refnum<k21>)  [unwired: 2 in]
  n1860 = while {
    tunnel: w49 -> [w4567]
    tunnel: w42 -> [w4566]
    tunnel: [w4564] -> _
    stop <- FALSE stop-if-true
    # "TEi43c Ozone UI Event Handler Loop"
    n1861 = event shown="[0] \"Ozone Zeroing\": Value Change" {
      selector: _ -> [_ _ _ _ _]
      dyn-events: _ -> [_ _ _ _ _]
      timeout: _ -> [_ _ _ _ _]
      tunnel: w4567 -> [w4575 w4613 w4621 w4628 w4636]
      tunnel: w4566 -> [w4574 w4612 w4620 w4627 w4635]
      tunnel: [w4573 w4611 w4619 w4626 w4634] -> w4564
      event "Ozone Zeroing": Value Change {
        n1862 = event-data() -> ()  [unwired: 1 in, 6 out]
        n1863 = flat-sequence {
          tunnel: w4575 -> [w4580]
          tunnel: w4574 -> [w4579]
          tunnel: [w4578] -> w4572
          tunnel: [w4576] -> w4568
          tunnel: w4572 -> [w4586]
          tunnel: [w4586] -> w4571
          tunnel: [w4584] -> w4569
          tunnel: w4568 -> [w4584]
          tunnel: w4571 -> [w4604]
          tunnel: [w4603] -> w4570
          tunnel: w4569 -> [w4605]
          tunnel: [w4610] -> w4573
          tunnel: w4570 -> [w4610]
          frame #0 {
            w4577 = TRUE
            n1864 = local write "Ozone eV6"(w4577) -> ()
            n1865 = Bundle(cluster=T5 {"Message"="", "Message Data"=variant} ("Message Cluster"), "Message"="V6", "Message Data"=w4577) -> (w4581:T5)
            n1866 = Enqueue Element(queue=w4580, element=w4581, error in (no error)=w4579) -> (queue out=w4576:refnum<queue>, error out=w4578:errorcluster)  [unwired: 1 in, 1 out]
          }
          frame #1 {
            # "10 Mins Count down"
            n1867 = for {
              N: 600 -> [w4596]
              i -> [w4595]
              stop <- w4588 stop-if-true
              n1868 = local read "Ozone Zeroing Abort"() -> (w4590:bool)
              n1869 = Subtract(x=w4596, y=w4595) -> (x-y=w4594:i32)
              n1870 = Decrement(x=w4594) -> (x-1=w4592:i32)
              n1871 = Wait (ms)(milliseconds to wait=u32 1000) -> ()  [unwired: 1 out]
              n1872 = case shown="True" w4590 {
                selector: w4590 -> [w4599 _]
                tunnel: [w4599 w4600] -> w4587
                frame False {
                }
                frame True {
                  n1873 = Two Button Dialog(message="Are you sure to abort Ozone Zeroing?") -> (T button?=w4600:bool)  [unwired: 2 in]
                }
              }
              n1874 = local read "Network disconnected"() -> (w4589:bool)
              n1875 = Or(x=w4589, y=w4587) -> (x .or. y?=w4588:bool)
              n1876 = Select(t=0, s=w4588, f=w4592) -> (s? t:f=→"Ozone Zeroing\nTime Remain (sec)":i32)
              n1877 = case shown="False" w4587 {
                selector: w4587 -> [w4598 _]
                frame False {
                  n1878 = local write "Ozone Zeroing Abort"(w4598) -> ()
                }
                frame True {
                }
              }
            }
          }
          frame #2 {
            w4602 = FALSE
            n1879 = local write "Ozone eV6"(w4602) -> ()
            n1880 = Bundle(cluster=T5 {"Message"="", "Message Data"=variant} ("Message Cluster"), "Message"="V6", "Message Data"=w4602) -> (w4606:T5)
            n1881 = Enqueue Element(queue=w4605, element=w4606, error in (no error)=w4604) -> (error out=w4603:errorcluster)  [unwired: 1 in, 2 out]
          }
          frame #3 {
            w4609 = FALSE ("Ozone Zeroing")
            n1882 = local write "Ozone Zeroing Abort"(w4609) -> ()
            n1883 = local write "Ozone Zeroing"(w4609) -> ()
          }
        }
      }
      event "Ozone eV6": Value Change {
        n1884 = event-data() -> ("NewVal"=w4614:bool)  [unwired: 1 in]
        n1885 = Bundle(cluster=T5 {"Message"="", "Message Data"=variant} ("Message Cluster"), "Message"="V6", "Message Data"=w4614) -> (w4615:T5)
        n1886 = Enqueue Element(queue=w4613, element=w4615, error in (no error)=w4612) -> (error out=w4611:errorcluster)  [unwired: 1 in, 2 out]
      }
      event "cRIO File IO Stop\n(USB Flash Drive Unmount)": Value Change {
        n1887 = event-data() -> ("NewVal"=w4618:bool)  [unwired: 1 in]
        n1888 = Bundle(cluster=T5 {"Message"="", "Message Data"=variant} ("Message Cluster"), "Message"="Stop File Write", "Message Data"=w4618) -> (w4622:T5)
        n1889 = Enqueue Element(queue=w4621, element=w4622, error in (no error)=w4620) -> (error out=w4619:errorcluster)  [unwired: 1 in, 2 out]
      }
      event "Ozone UDP Time Offset": Value Change {
        n1890 = event-data() -> ("NewVal"=w4625:i32)  [unwired: 1 in]
        n1891 = Bundle(cluster=T5 {"Message"="", "Message Data"=variant} ("Message Cluster"), "Message"="UDP Time Offset", "Message Data"=w4625) -> (w4629:T5)
        n1892 = Enqueue Element(queue=w4628, element=w4629, error in (no error)=w4627) -> (error out=w4626:errorcluster)  [unwired: 1 in, 2 out]
      }
      event "Confirm Flight Number": Value Change {
        n1893 = event-data() -> ()  [unwired: 1 in, 5 out]
        n1894 = flat-sequence {
          tunnel: w4635 -> [w4638]
          tunnel: w4636 -> [w4639]
          tunnel: [w4639] -> w4633
          tunnel: [w4638] -> w4632
          tunnel: [w4641] -> w4634
          tunnel: w4633 -> [w4643]
          tunnel: w4632 -> [w4642]
          frame #0 {
            n1895 = local write "cRIO File IO Stop\n(USB Flash Drive Unmount)"(FALSE ("cRIO File IO Stop\n(USB Flash Drive Unmount)")) -> ()
          }
          frame #1 {
            n1896 = local read "Flight Number"() -> (w4640:string)
            n1897 = Bundle(cluster=T5 {"Message"="", "Message Data"=variant} ("Message Cluster"), "Message"="Flight Number", "Message Data"=w4640) -> (w4644:T5)
            n1898 = Enqueue Element(queue=w4643, element=w4644, error in (no error)=w4642) -> (error out=w4641:errorcluster)  [unwired: 1 in, 2 out]
          }
        }
      }
    }
    "Ozone Event error out" <- w4564
  }
  n1899 = while {
    tunnel: w49 -> [w4654]
    shift-right: [w4649] -> _
    shift-left: w44 -> [w4651]
    shift-right: [w4647] -> w41
    shift-left: w45 -> [w4653]
    tunnel: w42 -> [w4648]
    stop <- w4647 stop-if-true
    # "TEi43c Ozone UI Command Sender"
    n1900 = Dequeue Element(queue=w4654, error in (no error)=w4648) -> (element=w4650:T5)  [unwired: 1 in, 3 out]
    n1901 = Unbundle By Name(w4650) -> ("Message"=w4652:string)
    n1902 = case shown="\"UDP Time Offset\"" w4652 {
      tunnel: w4653 -> [w4655 w4659 w4666 w4673 w4680]
      tunnel: w4651 -> [w4656 w4662 w4669 w4676 w4683]
      tunnel: w4650 -> [_ w4661 w4668 w4675 w4682]
      tunnel: [w4655 w4658 w4665 w4672 w4679] -> w4647
      tunnel: [w4656 w4657 w4664 w4671 w4678] -> w4649
      frame "False", Default {
      }
      frame "V6" {
        n1903 = shared-variable-write(w4662, w4659, w4661) -> (w4660:refnum<k21>, w4663:errorcluster)  [unwired: 1 in, 1 out]
        n1904 = Flush Stream(8:w4663, 11:w4660) -> (0:w4658:errorcluster, 3:w4657:refnum<k21>)  [unwired: 2 in, 1 out]
      }
      frame "Stop File Write" {
        n1905 = shared-variable-write(w4669, w4666, w4668) -> (w4667:refnum<k21>, w4670:errorcluster)  [unwired: 1 in, 1 out]
        n1906 = Flush Stream(8:w4670, 11:w4667) -> (0:w4665:errorcluster, 3:w4664:refnum<k21>)  [unwired: 2 in, 1 out]
      }
      frame "Flight Number" {
        n1907 = shared-variable-write(w4676, w4673, w4675) -> (w4674:refnum<k21>, w4677:errorcluster)  [unwired: 1 in, 1 out]
        n1908 = Flush Stream(8:w4677, 11:w4674) -> (0:w4672:errorcluster, 3:w4671:refnum<k21>)  [unwired: 2 in, 1 out]
      }
      frame "UDP Time Offset" {
        n1909 = shared-variable-write(w4683, w4680, w4682) -> (w4681:refnum<k21>, w4684:errorcluster)  [unwired: 1 in, 1 out]
        n1910 = Flush Stream(8:w4684, 11:w4681) -> (0:w4679:errorcluster, 3:w4678:refnum<k21>)  [unwired: 2 in, 1 out]
      }
    }
  }
  "Ozone command sender error out" <- w41
  n1911 = Obtain Queue(name (unnamed)="2BOzone_Command", element data type=w28) -> (queue out=w37:refnum<queue>, error out=w30:errorcluster)  [unwired: 3 in, 1 out]
  n1912 = Create Network Stream Writer Endpoint(6:w34, 7:10 ("writer buffer size"), 9:w28, 10:"//192.168.101.17/command/reader/2BOzone" ("reader url"), 11:"/command/writer/2BOzone" ("writer name")) -> (0:w33:errorcluster, 3:w32:refnum<k21>)  [unwired: 2 in]
  n1913 = while {
    tunnel: w37 -> [w4688]
    tunnel: w30 -> [w4687]
    tunnel: [w4685] -> _
    stop <- FALSE stop-if-true
    # "2BOzone UI Event Handler Loop"
    n1914 = event shown="[2] \"Simulate Inst Conc\": Value Change" {
      selector: _ -> [_ _ _ _ _ _ _ _]
      dyn-events: _ -> [_ _ _ _ _ _ _ _]
      timeout: _ -> [_ _ _ _ _ _ _ _]
      tunnel: w4688 -> [w4692 w4699 w4706 w4713 w4720 w4727 w4734 w4742]
      tunnel: w4687 -> [w4691 w4698 w4705 w4712 w4719 w4726 w4733 w4741]
      tunnel: [w4690 w4697 w4704 w4711 w4718 w4725 w4732 w4740] -> w4685
      event "Ambient = OFF\nCabin = ON": Value Change {
        n1915 = event-data() -> ("NewVal"=w4689:bool)  [unwired: 1 in]
        n1916 = Bundle(cluster=T5 {"Message"="", "Message Data"=variant} ("Message Cluster"), "Message"="Ambient/Cabin", "Message Data"=w4689) -> (w4693:T5)
        n1917 = Enqueue Element(queue=w4692, element=w4693, error in (no error)=w4691) -> (error out=w4690:errorcluster)  [unwired: 1 in, 2 out]
      }
      event "Simulate 2B Conc": Value Change {
        n1918 = event-data() -> ("NewVal"=w4696:bool)  [unwired: 1 in]
        n1919 = Bundle(cluster=T5 {"Message"="", "Message Data"=variant} ("Message Cluster"), "Message"="Simulate_conc", "Message Data"=w4696) -> (w4700:T5)
        n1920 = Enqueue Element(queue=w4699, element=w4700, error in (no error)=w4698) -> (error out=w4697:errorcluster)  [unwired: 1 in, 2 out]
      }
      event "Simulate Inst Conc": Value Change {
        n1921 = event-data() -> ("NewVal"=w4703:i32)  [unwired: 1 in]
        n1922 = Bundle(cluster=T5 {"Message"="", "Message Data"=variant} ("Message Cluster"), "Message"="Simulate_inst_conc", "Message Data"=w4703) -> (w4707:T5)
        n1923 = Enqueue Element(queue=w4706, element=w4707, error in (no error)=w4705) -> (error out=w4704:errorcluster)  [unwired: 1 in, 2 out]
      }
      event "Inst_alm_thresh": Value Change {
        n1924 = event-data() -> ("NewVal"=w4710:i32)  [unwired: 1 in]
        n1925 = Bundle(cluster=T5 {"Message"="", "Message Data"=variant} ("Message Cluster"), "Message"="Inst_alm_thresh", "Message Data"=w4710) -> (w4714:T5)
        n1926 = Enqueue Element(queue=w4713, element=w4714, error in (no error)=w4712) -> (error out=w4711:errorcluster)  [unwired: 1 in, 2 out]
      }
      event "3hr_alm_thresh": Value Change {
        n1927 = event-data() -> ("NewVal"=w4717:i32)  [unwired: 1 in]
        n1928 = Bundle(cluster=T5 {"Message"="", "Message Data"=variant} ("Message Cluster"), "Message"="3hr_alm_thresh", "Message Data"=w4717) -> (w4721:T5)
        n1929 = Enqueue Element(queue=w4720, element=w4721, error in (no error)=w4719) -> (error out=w4718:errorcluster)  [unwired: 1 in, 2 out]
      }
      event "Simulate 3hr Average Conc": Value Change {
        n1930 = event-data() -> ("NewVal"=w4724:dbl)  [unwired: 1 in]
        n1931 = Bundle(cluster=T5 {"Message"="", "Message Data"=variant} ("Message Cluster"), "Message"="Simulate_3hr_av_conc", "Message Data"=w4724) -> (w4728:T5)
        n1932 = Enqueue Element(queue=w4727, element=w4728, error in (no error)=w4726) -> (error out=w4725:errorcluster)  [unwired: 1 in, 2 out]
      }
      event "cRIO File IO Stop\n(USB Flash Drive Unmount)": Value Change {
        n1933 = event-data() -> ("NewVal"=w4731:bool)  [unwired: 1 in]
        n1934 = Bundle(cluster=T5 {"Message"="", "Message Data"=variant} ("Message Cluster"), "Message"="Stop File Write", "Message Data"=w4731) -> (w4735:T5)
        n1935 = Enqueue Element(queue=w4734, element=w4735, error in (no error)=w4733) -> (error out=w4732:errorcluster)  [unwired: 1 in, 2 out]
      }
      event "Confirm Flight Number": Value Change {
        n1936 = event-data() -> ()  [unwired: 1 in, 5 out]
        n1937 = flat-sequence {
          tunnel: w4741 -> [w4744]
          tunnel: w4742 -> [w4745]
          tunnel: [w4745] -> w4739
          tunnel: [w4744] -> w4738
          tunnel: [w4747] -> w4740
          tunnel: w4739 -> [w4749]
          tunnel: w4738 -> [w4748]
          frame #0 {
            n1938 = local write "cRIO File IO Stop\n(USB Flash Drive Unmount)"(FALSE ("cRIO File IO Stop\n(USB Flash Drive Unmount)")) -> ()
          }
          frame #1 {
            n1939 = local read "Flight Number"() -> (w4746:string)
            n1940 = Bundle(cluster=T5 {"Message"="", "Message Data"=variant} ("Message Cluster"), "Message"="Flight Number", "Message Data"=w4746) -> (w4750:T5)
            n1941 = Enqueue Element(queue=w4749, element=w4750, error in (no error)=w4748) -> (error out=w4747:errorcluster)  [unwired: 1 in, 2 out]
          }
        }
      }
    }
    "2BOzone Event error out" <- w4685
  }
  n1942 = while {
    tunnel: w37 -> [w4760]
    shift-right: [w4755] -> _
    shift-left: w32 -> [w4757]
    shift-right: [w4753] -> w29
    shift-left: w33 -> [w4759]
    tunnel: w30 -> [w4754]
    stop <- w4753 stop-if-true
    # "2BOzone UI Command Sender"
    n1943 = Dequeue Element(queue=w4760, error in (no error)=w4754) -> (element=w4756:T5)  [unwired: 1 in, 3 out]
    n1944 = Unbundle By Name(w4756) -> ("Message"=w4758:string)
    n1945 = case shown="\"3hr_alm_thresh\"" w4758 {
      tunnel: w4759 -> [w4761 w4765 w4772 w4779 w4786 w4793 w4800 w4807 w4814]
      tunnel: w4757 -> [w4762 w4768 w4775 w4782 w4789 w4796 w4803 w4810 w4817]
      tunnel: w4756 -> [_ w4767 w4774 w4781 w4788 w4795 w4802 w4809 w4816]
      tunnel: [w4761 w4764 w4771 w4778 w4785 w4792 w4799 w4806 w4813] -> w4753
      tunnel: [w4762 w4763 w4770 w4777 w4784 w4791 w4798 w4805 w4812] -> w4755
      frame "False", Default {
      }
      frame "Ambient/Cabin" {
        n1946 = shared-variable-write(w4768, w4765, w4767) -> (w4766:refnum<k21>, w4769:errorcluster)  [unwired: 1 in, 1 out]
        n1947 = Flush Stream(8:w4769, 11:w4766) -> (0:w4764:errorcluster, 3:w4763:refnum<k21>)  [unwired: 2 in, 1 out]
      }
      frame "Simulate_conc" {
        n1948 = shared-variable-write(w4775, w4772, w4774) -> (w4773:refnum<k21>, w4776:errorcluster)  [unwired: 1 in, 1 out]
        n1949 = Flush Stream(8:w4776, 11:w4773) -> (0:w4771:errorcluster, 3:w4770:refnum<k21>)  [unwired: 2 in, 1 out]
      }
      frame "Simulate_inst_conc" {
        n1950 = shared-variable-write(w4782, w4779, w4781) -> (w4780:refnum<k21>, w4783:errorcluster)  [unwired: 1 in, 1 out]
        n1951 = Flush Stream(8:w4783, 11:w4780) -> (0:w4778:errorcluster, 3:w4777:refnum<k21>)  [unwired: 2 in, 1 out]
      }
      frame "Inst_alm_thresh" {
        n1952 = shared-variable-write(w4789, w4786, w4788) -> (w4787:refnum<k21>, w4790:errorcluster)  [unwired: 1 in, 1 out]
        n1953 = Flush Stream(8:w4790, 11:w4787) -> (0:w4785:errorcluster, 3:w4784:refnum<k21>)  [unwired: 2 in, 1 out]
      }
      frame "3hr_alm_thresh" {
        n1954 = shared-variable-write(w4796, w4793, w4795) -> (w4794:refnum<k21>, w4797:errorcluster)  [unwired: 1 in, 1 out]
        n1955 = Flush Stream(8:w4797, 11:w4794) -> (0:w4792:errorcluster, 3:w4791:refnum<k21>)  [unwired: 2 in, 1 out]
      }
      frame "Simulate_3hr_av_conc" {
        n1956 = shared-variable-write(w4803, w4800, w4802) -> (w4801:refnum<k21>, w4804:errorcluster)  [unwired: 1 in, 1 out]
        n1957 = Flush Stream(8:w4804, 11:w4801) -> (0:w4799:errorcluster, 3:w4798:refnum<k21>)  [unwired: 2 in, 1 out]
      }
      frame "Stop File Write" {
        n1958 = shared-variable-write(w4810, w4807, w4809) -> (w4808:refnum<k21>, w4811:errorcluster)  [unwired: 1 in, 1 out]
        n1959 = Flush Stream(8:w4811, 11:w4808) -> (0:w4806:errorcluster, 3:w4805:refnum<k21>)  [unwired: 2 in, 1 out]
      }
      frame "Flight Number" {
        n1960 = shared-variable-write(w4817, w4814, w4816) -> (w4815:refnum<k21>, w4818:errorcluster)  [unwired: 1 in, 1 out]
        n1961 = Flush Stream(8:w4818, 11:w4815) -> (0:w4813:errorcluster, 3:w4812:refnum<k21>)  [unwired: 2 in, 1 out]
      }
    }
  }
  "2BOzone command sender error out" <- w29
